vi "W7XBolo2017_Flo.vi"(1 "FPGA VI\nReference In":refnum<k20>) -> (0 "FPGA VI Reference Out":refnum<k20>)   [LabVIEW 2014]
uses:
  <vilib>/Platform/TimedLoop/XDataNode/timing_clust.ctl
  <vilib>/Platform/TimedLoop/XDataNode/nitl_modes.ctl
  <vilib>/Platform/TimedLoop/XDataNode/wakeup.ctl
  <vilib>/userdefined/High Color/nirio_resource_hc.ctl
  <vilib>/DAQmx/write.llb/DAQmx Write (Analog 1D DBL NChan 1Samp).vi
  <vilib>/FPGAPlugInAG/PCI-7813R/niLvFpga_Open_PCI-7813R.vi
  <vilib>/Utility/error.llb/Error Cluster From Error Code.vi
  <vilib>/rvi/errors/niLvFpgaAdjustHostInterfaceError.vi
  <vilib>/Utility/file.llb/Read From Spreadsheet File (I64).vi
  <vilib>/Utility/file.llb/Read From Spreadsheet File (DBL).vi
  <vilib>/DAQmx/create/channels.llb/DAQmx Create Channel (AO-Voltage-Basic).vi
  <vilib>/DAQmx/miscellaneous.llb/DAQmx Fill In Error Info.vi
  <vilib>/rvi/interface/common/niFpgaWaitOnOcc.vi
  <vilib>/httpClient/POSTBuffer.vi
  <vilib>/FPGAPlugInAG/PCI-7813R/niLvFpga_Close_PCI-7813R.vi
  <vilib>/Platform/TimedLoop/XDataNode/XDataNode.xnode
  <vilib>/rvi/interface/nirviOpenFPGA/nirviOpenFPGA.xnode
  FPGA Bitfiles/W7XBolo2017_FPGATarget_fmain2014_DACRangeVoltage.lvbitx
  f_main_2014.vi
  <vilib>/rvi/interface/nirviReadWriteControl/nirviReadWriteControl.xnode
  <vilib>/rvi/interface/nirviMethod/nirviMethod.xnode
  <vilib>/rvi/interface/nirviCloseFPGA/nirviCloseFPGA.xnode
  <vilib>/Platform/TimedLoop/XDataNode/XDNodeRunTimeDep.lvlib
  <vilib>/Analysis/NI_AALBase.lvlib
  <vilib>/httpClient/LabVIEWHTTPClient.lvlib
  <resource>/objmgr/daqmx.rc
  <vilib>/DAQmx/configure/timing.llb/DAQmx Timing (Sample Clock).vi
  <vilib>/DAQmx/write.llb/DAQmx Write (Analog 2D DBL NChan NSamp).vi
  NiFpgaLv.dll
  <vilib>/FPGAPlugInAG/PCI-7813R/niLvFpga_AcknowledgeIrq_PCI-7813R.vi
  <vilib>/FPGAPlugInAG/PCI-7813R/niLvFpga_ConfigureFifo_PCI-7813R.vi
  <vilib>/rvi/errors/niLvFpgaMergeErrorWithErrorCode.vi
panel:
  out "Time until Acqusition":dbl(slide)=60.0 scale=0.0..60.0
  out "DAQ Timer":dbl
  in  "Tab Control 7":T1(tab)
  in  "FreqSelRing":u16(ring)=1 items=["0.8 ms", "1.6 ms", "3.2 ms", "6.4 ms", "12.8 ms", "19.2 ms"]
  in  "SecondFilter":bool=TRUE
  out "SampleTime":sgl=0.0016
  in  "Global DAC Range Setting":u8(knob)=3 scale=0.0..3.0
  out "No. of Samples:":u32=26000
  out "Measured Time for DAQ [ms]":u32
  out "Take file for DAC?":bool
  in  "?":bool=TRUE
  out "Take Input for DAC?":bool
  out "single channel voltage":dbl format="%#_13g"
  in  "DAC and AD Settings":i32(slide)=3 scale=0.0..3.0
  out "Time of Acqusition [s]":dbl=40.0
  out "predicted time [ms] to finalize DAQ":dbl
  out "real time P_rad":dbl format="%#_13g"
  in  "single channel signal factor":dbl=20000.0
  out "voltage on\nsingle channel AO":bool=TRUE
  in  "single channel number":i64=7
  out "loop status":bool
  in  "Auto ECRH Time\nor manual control":bool=TRUE
  out "ECRH duration":dbl=30.0
  in  "manual & default\nDAQ time":dbl=30.0
  out "time needed to\nfind ECRH duration":i64
  in  "SavGol side points":i32=10
  in  "order polynomial":i32=2
  in  "RTPRad voltage factor":dbl=1.0
  out "voltage out state":string
  out "voltage errorsource":string
  out "AO error":errorcluster
  in  "source clock":tag="OnboardClock"
  in  "RegenMode":i32(ring)=10158 items=["Allow Regeneration"=10097, "Do Not Allow Regeneration"=10158]
  in  "AO.DataXferMech 2":i32(ring)=10054 items=["DMA"=10054, "Interrupts"=10204, "Programmed I/O"=10264, "USB Bulk"=12590]
  in  "AO.DataXferReqCond 2":i32(ring)=10242 items=["Onboard Memory Empty"=10235, "Onboard Memory Half Full or Less"=10239, "Onboard Memory Less than Full"=10242]
  in  "sample mode":i32(ring)=10123 items=["Finite Samples"=10178, "Continuous Samples"=10123, "Hardware Timed Single Point"=12522]
  in  "Manual Timing of AO":dbl=100000.0
  out "watchdog loop counter":i32
  out "loop counter":i32
  in  "SkipVoltageOut":bool
  out "Percentage of PC buffer occupied":u8(slide) scale=0.0..100.0
  out "Percentage of OnBoard buffer occupied":u8(slide) scale=0.0..100.0
  out "PC Buffer SpaceAvail":u32
  out "How many \"Write Chunk\" (periods of latency)\nstored in the PC buffer + board buffer?":dbl
  out "How many samples stored in the \nPC buffer + board buffer?":dbl
  in  "Samples per channel to write\n(write chunk)":u32=14
  in  "samples per channel":i32=28
  out "Output.OnbrdBufSize":u32
  out "PC Buffer CurrWritePos 2":dbl
  out "AO output loop timing":dbl
  out "Board TotalSampPerChanGenerated":dbl
  out "How many seconds to empty the \nPC buffer+ board buffer? 2":dbl
  out "RTPVO current val":dbl
  out "SCVO current val":dbl
  in  "Use Voltage or Power for\nsingel channel AO?":bool=TRUE
  in  "voltage watchdog stop":bool
  out "Output.BufSize":u32
  in  "Path to channel selection file":path=path "C:/Users/Administrator/Desktop/short.channel_selection.dat"
  out "file import":i64[][](array[numeric])
  in  "channel selection input":i32[][](array[numeric])=[[1]]
  in  "Read Channel Selection from file":bool=TRUE
  out "Channel Selection\nfrom input?":bool
  out "final channel selection":i64[][](array[numeric])=[[0], [1], [2], [3], [4], [5], [6], [7], [8], [9], [10], [11], [12], [13], [14], [15], [16], [17], [18], [19], [20], [21], [22], [23], [24], [25], [26], [27], [28], [29], [30], [31]]
  out "final channel\nselection size":i32
  in  "Trigger Source":i32(slide)=1 scale=0.0..3.0
  in  "Set Manual Time [ns]":i64=1503619200000000000
  out "Presamples If -1, then no trigger detected)":i32
  out "DAQ wait time (should be = TWT":i32=-1
  out "Countdown Time":u32
  out "Calibration Time":u32
  out "Total wait time (TWT) Typically 59 s":u32
  in  "Pre-start time (ms) of\nDAQ Typically set to 1000 ms":i32=10000
  in  "Fixed T-60sec before T1 = T0":i32=60000
  in  "Wait-Time until Trigger; published on CODAC":u32=10000
  out "current epoch time timestamp":timestamp
  out "Number of nanoseconds with offset to 1904":i64
  in  "samples to exclude":u32=1000
  out "final trigger time":i64
  out "last trigger time by codac":i64
  out "start time":i64
  out "T-Start [for Display)\nShould be -1 [s]":sgl=-1.0
  out "DAQ Start (epoch) [ns]":i64
  out "Downtime after T0 until DAQ [ns]":i64
  in  "timing of plots fix factor":sgl=1.0
  in  "AddOn time":dbl=5.0
  in  "Tau00":dbl[](array[numeric])=[0.11537597448635277, 0.11755685958822219, 0.1164214694473907, 0.11697577239117866, 0.110451, 0.12010942076824872, 0.11766714993048435, 0.11910426529905502, 0.10999582403545866, 0.11118469600664964, 0.10580731993585431, 0.11217289808087993, 0.11223398365603839, 0.11204749607224823, 0.11263624992738425, 0.11091290284745299, 0.11721868902521211, 0.11737061531613151, 0.11788987597885038, 0.11600007869942867, 0.11334307549251021, 0.11228572042130423, 0.1129521332802642, 0.11724104097990388, 0.11740306056822605, 0.11529467898123245, 0.11828175507687082, 0.11829012392284373, 0.11773460668621359, 0.1155776803231521, 0.11650421728110884, 0.11571658330095998, 0.11068789319935994, 0.10986016888144867, 0.10999340462233435, 0.11095550249493497, 0.11143937038853975, 0.11095468517729823, 0.11130783288802211, 0.11084408945769118, 0.10830137260394793, 0.10662335345199567, 0.10535002662491703, 0.10738515206651872, 0.10772145508062766, 0.1053368317440755, 0.10408446186375701, 0.10449038510758271, 0.11178895597256559, 0.11021628063681403, 0.11220331344682449, 0.11111721341359461, 0.10889811436206044, 0.11638094730098773, 0.11290278568076087, 0.11205006536853761, 0.1094907553786962, 0.11634433136641531, 0.11037702264320227, 0.1104223688763365, 0.11352480237507033, 0.11341744936097128, 0.10916961452972393, 0.11332789199343518, 0.11107001747086552, 0.1083853978889723, 0.11029711206697901, 0.11063487469805744, 0.10926615257922916, 0.10988377001368325, 0.10782095764307568, 0.1073886205272185, 0.10829341805096283, 0.10953345610425252, 0.10953147401563214, 0.10933747673483066, 0.1093210854374169, 0.10892908051404164, 0.10841565534876087, 0.10934867623657209, 0.11431979794745441, 0.11469548527952493, 0.11256319960938391, 0.11004758193350624, 0.1086775698186096, 0.10860163257332957, 0.10972644811806966, 0.1244329993560779, 0.10848514148619942, 0.10753497988240919, 0.11378450261362759, 0.11397799701939393, 0.10865166632049855, 0.10955778865143037, 0.11184264538711042, 0.11080028199806266, 0.11230419705417591, 0.11150150302047147, 0.10940920103499238, 0.0, 0.11018788195565775, 0.1109851624674225, 0.10888498891279576, 0.10950524535111039, 0.11209787924272374, 0.11180887164622381, 0.1110290995583749, 0.11040609393156747, 0.1103438351320269, 0.1101975468642728, 0.10923728746964355, 0.0, 0.11021638606642407, 0.0, 0.0, 0.0, 0.0, 0.0, 0.0, 0.0, 0.5609466646481899, 0.0, 0.0, 0.0, 0.0, 0.0, 0.0, 0.4058686463981613, 0.11537597448635277]
  in  "Kappa00":dbl[](array[numeric])=[0.0008396193201719739, 0.0008193409803026575, 0.0008327489337370494, 0.0008094925878469488, 0.00039367506543457065, 0.0008063058560714545, 0.0008451910365158945, 0.0007992358755606012, 0.0008323076933152601, 0.0008570762215527662, 0.0007628861690345087, 0.0008061906602308296, 0.0008540424353779365, 0.0008301118976821594, 0.0008577435335519969, 0.0008553747566925557, 0.000838644207815748, 0.0008273548270536888, 0.0008111923709406437, 0.0008317040544888235, 0.0002062919117538751, 0.0007971782754034694, 0.0007777938427968141, 0.0007983063012770449, 0.0007902138174646686, 0.0007777700527572154, 0.0008086241703327105, 0.0007894905085128677, 0.0008499052168857277, 0.0008231536154986703, 0.0008290108212352768, 0.0008015771948583539, 0.0004219784890145567, 0.0008028223447312654, 0.0007908997677950409, 0.0007688640721813007, 0.0007923143974006498, 0.0007943700234243013, 0.000794807683089336, 0.0007644407575630641, 0.0008256914284962689, 0.0008464663657085921, 0.0008525498714753285, 0.0008605939917038706, 0.0008075301142063146, 0.0008582080819176783, 0.0008833831995156997, 0.0008817750426330745, 0.0008736825873144331, 0.0008712555197947145, 0.0008599116319459445, 0.0008597288697454142, 0.0008850439198466119, 0.0008360600624626481, 0.0008729149198757765, 0.0008652970161905564, 0.000878176403644396, 0.000814669724061475, 0.0008492936703496222, 0.0008335090067364612, 0.0009020306039280142, 0.0009060889736233363, 0.000873120149823901, 0.0008865804075398461, 0.0008218319952538781, 0.0008647381541051004, 0.0008535415687509321, 0.000868609807906937, 0.0008544506047017487, 0.0008552184337763689, 0.0008772351584693919, 0.0008899531428744609, 0.0009049492537694576, 0.000908105157129488, 0.0009441675693280472, 0.0008666158415307141, 0.0008904383660716827, 0.00090533600441176, 0.0009193630525411423, 0.0009209094258700529, 0.0008671616817531277, 0.0008573033056411677, 0.0008894545060438134, 0.0008393076570230061, 0.0008809839906701387, 0.0008713273912310079, 0.0008529389904228485, 0.0008798583497112145, 0.0007606961064025662, 0.0007618681674480262, 0.0008830002472907413, 0.0008434447500347438, 0.0008157810403546725, 0.0008170412330426688, 0.000817539692314199, 0.0008060567476264818, 0.0007745714382802376, 0.0007738842512393123, 0.0007910139604008742, -1.9640688433259297e-10, 0.000780575223559956, 0.0007962779122750964, 0.000790630439080113, 0.0008189866992119251, 0.0008220353590981327, 0.0008259174124746273, 0.0008237041516630779, 0.0008128375228315313, 0.0008025139618430593, 0.0007891459070721132, 0.0007835394415130632, 1.4659311061625464e-11, 0.0007713911232202254, -1.136328152026204e-11, 7.33972615530204e-11, -5.807996136265078e-12, 1.50989391544806e-10, -2.091237015882531e-11, -2.2968171315336452e-11, 3.2003514158147334e-12, -1.18410213996469e-13, 3.9907860061368183e-13, 1.2900003061146403e-11, -7.996494711993759e-11, 1.2728268766879732e-10, -2.7124534936566837e-11, -1.0618681361847593e-11, 1.1300143559461795e-05]
  in  "RB000":dbl[](array[numeric])=[964.4665558152926, 984.0412138536651, 1001.0627256989599, 1012.7898525309201, 986.7279110070629, 993.5830261423998, 1133.718466702734, 1026.065541032409, 981.7525515631839, 976.6051330676225, 975.1369773387203, 983.6003740876943, 945.3052421117454, 944.0131212191011, 937.9865397688445, 924.775520494105, 1002.3909240348048, 1016.474188810108, 1008.3024841336951, 997.8517562562979, 1396.1357804303618, 1011.7052948010587, 1006.0858095523904, 1000.525119034801, 1016.071205963885, 1008.5531713944379, 1001.2101495655734, 1012.9539707105694, 909.9522463978296, 921.8611396886308, 930.8535575645451, 937.6736260749049, 1835.253905213153, 905.3151174073253, 915.4686408360067, 932.2842954450018, 878.6376527118448, 888.8892103361444, 896.5962281010978, 917.195767017641, 953.2009542047422, 949.8476734916919, 945.7180214798805, 934.1303098026676, 944.4309270141721, 922.393020385211, 908.2770101975661, 902.8479184676862, 997.7185120044248, 1004.633250147941, 1012.2992174178987, 1022.8972656361334, 988.1138139759116, 1012.5096483256309, 926.7526927543831, 940.6499588809413, 987.4981539235332, 1030.6093168535383, 996.69488158787, 998.6770565199763, 937.2653710614366, 942.0245103372197, 975.0990877775471, 954.8089604337308, 987.3564837474132, 941.2547128561528, 982.5095895382428, 979.0417371038707, 995.2373497220817, 994.8506309175264, 989.7979732647505, 986.9344569144992, 979.4724674608722, 951.8026661804106, 928.3096097998925, 980.4648125251251, 967.8736951300871, 960.399052288677, 950.3474867516031, 931.7877057694141, 925.6104123406642, 925.2905333073797, 925.2586242376997, 996.0089625341668, 969.8590336679081, 973.5395443351913, 978.7443359479869, 1329.6132687126426, 951.8837808548863, 946.7262849537287, 933.7058147126331, 940.8228530266879, 876.367589172054, 864.1420943242144, 855.6188139335973, 854.7591574173059, 955.1936774096923, 969.1826763753277, 970.8033011923455, 0.0, 935.2179320514933, 937.6581182076873, 940.1867678977421, 939.4080093580444, 850.4194498630884, 857.7406858104588, 867.3881837894808, 884.270800315495, 892.6618762043922, 899.3995556852765, 915.5186423922648, 0.0, 919.5685811076437, 0.0, 0.0, 0.0, 0.0, 0.0, 0.0, 0.0, 0.0, 0.0, 0.0, 0.0, 0.0, 0.0, 0.0, 0.0]
  in  "Switch to fixed \nCalibration Values":bool
  in  "Clear all Values \nfrom Beginning":bool
  in  "Cancel Button":bool
  out "Actual Depth":u32=256
  in  "Trigger No Choice from MDS+ Website\n0 for old 1 during OP":i32
  in  "AD 7730 Bit Settings":i32(slide) scale=0.0..1.0
  out "CODAC trigger time":i64
  out "date/time string":string
  out "Sucessfull HTTP return?":bool
  out "progId":dbl
  in  "Tab Control":T2(tab)
  out "real time P_rad array":dbl[](array[numeric])
  out "all plot":cluster{cluster{dbl, "element":dbl}[]}[](graph)
  out "full P_rad [MW] HBC":dbl[](array[numeric])
  out "single channel voltage array":dbl[](array[numeric])
  out "full P_rad [MW] VBC":dbl[](array[numeric])
  in  "Tab Control 4":enum32{"1 to 64", "65 to 128"}(tab)
  out "Raw 33-64":T3={"Channels 33 - 40"={"tstart"=-1.0, "FPGSampleTime"=0.0007999999797903001, []}, "Channels 41 - 48"={"tstart"=-1.0, "FPGSampleTime"=0.0007999999797903001, []}, "Channels 49 - 56"={"tstart"=-1.0, "FPGSampleTime"=0.0007999999797903001, []}, "Channels 57 - 64"={"tstart"=-1.0, "FPGSampleTime"=0.0007999999797903001, []}}
  out "Raw 1-32":T4={"Channels 1- 8"={"tstart"=-1.0, "FPGSampleTime"=0.0007999999797903001, []}, "Channels 9 - 16"={"tstart"=-1.0, "FPGSampleTime"=0.0007999999797903001, []}, "Channels 17 - 24"={"tstart"=-1.0, "FPGSampleTime"=0.0007999999797903001, []}, "Channels 25 - 32"={"tstart"=-1.0, "FPGSampleTime"=0.0007999999797903001, []}}
  out "Raw 97 - 128":T5
  out "Raw 65 - 97":T6={"Channels 65 - 71"={"tstart"=-1.0, "FPGSampleTime"=0.0007999999797903001, []}, "Channels 73 - 80"={"tstart"=0.0, "FPGSampleTime"=0.0, []}, "Channels 81 - 88"={"tstart"=0.0, "FPGSampleTime"=0.0, []}, "Channels 89- 96"={"tstart"=0.0, "FPGSampleTime"=0.0, []}}
  in  "Tab Control 13":enum32{"1 to 64", "65 to 128"}(tab)
  out "Adjusted 33-64":T3={"Channels 33 - 40"={"tstart"=-1.0, "FPGSampleTime"=0.0007999999797903001, []}, "Channels 41 - 48"={"tstart"=-1.0, "FPGSampleTime"=0.0007999999797903001, []}, "Channels 49 - 56"={"tstart"=-1.0, "FPGSampleTime"=0.0007999999797903001, []}, "Channels 57 - 64"={"tstart"=-1.0, "FPGSampleTime"=0.0007999999797903001, []}}
  out "Adjusted 1-32":T4={"Channels 1- 8"={"tstart"=-1.0, "FPGSampleTime"=0.0007999999797903001, []}, "Channels 9 - 16"={"tstart"=-1.0, "FPGSampleTime"=0.0007999999797903001, []}, "Channels 17 - 24"={"tstart"=-1.0, "FPGSampleTime"=0.0007999999797903001, []}, "Channels 25 - 32"={"tstart"=-1.0, "FPGSampleTime"=0.0007999999797903001, []}}
  out "Adjusted 97 - 129":T5
  out "Adjusted 65 - 98":T6={"Channels 65 - 71"={"tstart"=-1.0, "FPGSampleTime"=0.0007999999797903001, []}, "Channels 73 - 80"={"tstart"=0.0, "FPGSampleTime"=0.0, []}, "Channels 81 - 88"={"tstart"=0.0, "FPGSampleTime"=0.0, []}, "Channels 89- 96"={"tstart"=0.0, "FPGSampleTime"=0.0, []}}
  in  "Tab Control 6":enum32{"1 to 64", "65 to 128"}(tab)
  out "Pow 33-64":T3
  out "Pow 1-32":T4={"Channels 1- 8"={"tstart"=-1.0, "FPGSampleTime"=0.0007999999797903001, []}, "Channels 9 - 16"={"tstart"=-1.0, "FPGSampleTime"=0.0007999999797903001, []}, "Channels 17 - 24"={"tstart"=0.0, "FPGSampleTime"=0.0, []}, "Channels 25 - 32"={"tstart"=0.0, "FPGSampleTime"=0.0, []}}
  out "Pow 97 - 128":T5
  out "Pow 65 - 96":T6={"Channels 65 - 71"={"tstart"=-1.0, "FPGSampleTime"=0.0007999999797903001, []}, "Channels 73 - 80"={"tstart"=0.0, "FPGSampleTime"=0.0, []}, "Channels 81 - 88"={"tstart"=0.0, "FPGSampleTime"=0.0, []}, "Channels 89- 96"={"tstart"=0.0, "FPGSampleTime"=0.0, []}}
  out "full P_rad plot":T7(graph)
  out "CalibRefFoilFit path":string
  out "BoloCalibRefFoilFit Satus":bool
  out "Offset path":string
  out "Offset Status":bool
  out "RTau Path":string
  out "RTau Status":bool
  out "MKappa path":string
  out "RRes path":string
  out "MTau path":string
  out "RRes Status":bool
  out "MKappa Status":bool
  out "MTau status":bool
  out "BoloPower path":string
  out "QSBParms path":string
  out "BoloSignal path":string
  out "CalibMeasFoilCurrent path":string
  out "CalibRefFoilCurrent path":string
  out "MRes path":string
  out "RKappa path":string
  out "RKappa Status":bool
  out "CalibRefFoilCurrent status":bool
  out "CalibMeasFoilCurrent status":bool
  out "MRes status":bool
  out "BoloSignal status":bool
  out "QSBParms status":bool
  out "BoloPower status":bool
  out "SingleChannelFeedback status":bool
  out "SingleChannelFeedback path":string
  out "ChannelSelection status":bool
  out "ChannelSelection path":string
  out "Bolo_HBCmPrad path":string
  out "Bolo_HBCmPrad status":bool
  out "CalibMeasFoilFit path":string
  out "CalibMeasFoilFit status":bool
  out "Bolo_VBCPrad status":bool
  out "Bolo_VBCPrad path":string
  out "RT_P_rad path":string
  out "RT_P_rad status":bool
  out "MessStatus 65-96":bool[](array[boolean])
  out "MessStatus 97-128":bool[](array[boolean])
  out "MessStatus 33-64":bool[](array[boolean])
  out "MessStatus 1-32":bool[](array[boolean])
  out "RefStatus 97-128":bool[](array[boolean])
  out "RefStatus 1-32":bool[](array[boolean])
  out "RefStatus 33-64":bool[](array[boolean])
  out "RefStatus 65-96":bool[](array[boolean])
  out "voltage status":bool
  out "result":bool
  out "FilterTimeOut":bool
  out "Fehler READ U+P":bool
  out "Fehler":bool
  out "Timed Out":bool
  out "BoloAdjusted path":string
  out "BoloSignal status 2":bool
  in  "Tab Control 14":T8(tab)=enum."Parlog"
  out "BoloSignalErrorOut 2":errorcluster
  out "body Parlog 18":string
  out "headers parms 18":string
  out "headers 18":string
  out "body 18":string
  in  "Tab Control 12":T9(tab)=enum."Parlog"
  out "RT_P_rad ErrorOut":errorcluster
  out "body Parlog 17":string
  out "headers 17":string
  out "body 17":string
  out "headers parms 17":string
  in  "Tab Control 31":T10(tab)=enum."Parlog"
  out "parms error out":errorcluster
  out "QSB Parms Out body chanDesc":string
  out "QSB Parms Out headers chanDesc":string
  in  "Tab Control 30":T11(tab)=enum."Parlog"
  out "CalibMeasFoilFit 2":errorcluster
  out "body Parlog":string
  out "headers parms":string
  out "body":string
  out "headers":string
  in  "Tab Control 29":T12(tab)=enum."Parlog"
  out "RKappaErrorOut":errorcluster
  out "body Parlog 3":string
  out "headers parms 3":string
  out "body 3":string
  out "headers 3":string
  in  "Tab Control 28":enum32{"MTau ErrorOut", "Parlog", "Datastream"}(tab)=enum."Parlog"
  out "MTauErrorOut":errorcluster
  out "body Parlog 16":string
  out "headers parms 16":string
  out "body 16":string
  out "headers 16":string
  in  "Tab Control 27":enum32{"MRes ErrorOut", "Parlog", "Datastream"}(tab)=enum."Parlog"
  out "MResErrorOut":errorcluster
  out "body Parlog 6":string
  out "headers parms 6":string
  out "body 6":string
  out "headers 6":string
  in  "Tab Control 26":T13(tab)=enum."Parlog"
  out "BoloPowerRawErrorOut":errorcluster
  out "body Parlog 10":string
  out "headers parms 10":string
  out "body 10":string
  out "headers 10":string
  in  "Tab Control 25":T14(tab)=enum."Parlog"
  out "CalibMeasFoilCurrentErrorOut":errorcluster
  out "body Parlog 7":string
  out "headers parms 7":string
  out "body 7":string
  out "headers 7":string
  in  "Tab Control 24":T15(tab)=enum."Parlog"
  out "BoloSignalErrorOut":errorcluster
  out "body Parlog 9":string
  out "headers parms 9":string
  out "body 9":string
  out "headers 9":string
  in  "Tab Control 23":T16(tab)=enum."Parlog"
  out "CalibRefFoilCurrentErrorOut":errorcluster
  out "body Parlog 8":string
  out "headers parms 8":string
  out "body 8":string
  out "headers 8":string
  in  "Tab Control 22":T17(tab)=enum."Parlog"
  out "BoloCalibRefFoilFitErrorOut":errorcluster
  out "body Parlog 11":string
  out "headers parms 11":string
  out "body 11":string
  out "headers 11":string
  in  "Tab Control 21":enum32{"RRes ErrorOut", "Parlog", "Datastream"}(tab)=enum."Parlog"
  out "RResErrorOut":errorcluster
  out "body Parlog 5":string
  out "headers parms 5":string
  out "body 5":string
  out "headers 5":string
  in  "Tab Control 20":T18(tab)=enum."Parlog"
  out "OffsetErrorOut":errorcluster
  out "body Parlog 15":string
  out "headers parms 15":string
  out "body 15":string
  out "headers 15":string
  in  "Tab Control 19":T19(tab)=enum."Parlog"
  out "MKappaErrorOut":errorcluster
  out "body Parlog 2":string
  out "headers parms 2":string
  out "body 2":string
  out "headers 2":string
  in  "Tab Control 8":T20(tab)=enum."Parlog"
  out "ChannelSelection ErrorOut":errorcluster
  out "ChannelSelection body Parlog":string
  out "ChannelSelection headers parms":string
  out "ChannelSelection body":string
  out "ChannelSelection headers":string
  out "error out":errorcluster
  out "error out Cal":errorcluster
  in  "chanDescs":T21(array[cluster])=[{"name"="HBCm_U30_01", "active"=1, "physicalQuantity"={"type"="A"}}, {"name"="HBCm_U30_02", "active"=1, "physicalQuantity"={"type"="A"}}, {"name"="HBCm_U30_03", "active"=1, "physicalQuantity"={"type"="A"}}, {"name"="HBCm_U30_04", "active"=1, "physicalQuantity"={"type"="A"}}, {"name"="HBCm_U30_05", "active"=1, "physicalQuantity"={"type"="A"}}, {"name"="HBCm_U30_06", "active"=1, "physicalQuantity"={"type"="A"}}, {"name"="HBCm_U30_07", "active"=1, "physicalQuantity"={"type"="A"}}, {"name"="HBCm_U30_08", "active"=1, "physicalQuantity"={"type"="A"}}, {"name"="HBCm_U30_09", "active"=1, "physicalQuantity"={"type"="A"}}, {"name"="HBCm_U30_10", "active"=1, "physicalQuantity"={"type"="A"}}, {"name"="HBCm_U30_11", "active"=1, "physicalQuantity"={"type"="A"}}, {"name"="HBCm_U30_12", "active"=1, "physicalQuantity"={"type"="A"}}, {"name"="HBCm_U30_013", "active"=1, "physicalQuantity"={"type"="A"}}, {"name"="HBCm_U30_14", "active"=1, "physicalQuantity"={"type"="A"}}, {"name"="HBCm_U30_15", "active"=1, "physicalQuantity"={"type"="A"}}, {"name"="HBCm_U30_16", "active"=1, "physicalQuantity"={"type"="A"}}, {"name"="HBCm_U30_17", "active"=1, "physicalQuantity"={"type"="A"}}, {"name"="HBCm_U30_18", "active"=1, "physicalQuantity"={"type"="A"}}, {"name"="HBCm_U30_19", "active"=1, "physicalQuantity"={"type"="A"}}, {"name"="HBCm_U30_20", "active"=1, "physicalQuantity"={"type"="A"}}, {"name"="HBCm_U30_21", "active"=1, "physicalQuantity"={"type"="A"}}, {"name"="HBCm_U30_22", "active"=1, "physicalQuantity"={"type"="A"}}, {"name"="HBCm_U30_23", "active"=1, "physicalQuantity"={"type"="A"}}, {"name"="HBCm_U30_24", "active"=1, "physicalQuantity"={"type"="A"}}, {"name"="HBCm_U30_25", "active"=1, "physicalQuantity"={"type"="A"}}, {"name"="HBCm_U30_26", "active"=1, "physicalQuantity"={"type"="A"}}, {"name"="HBCm_U30_27", "active"=1, "physicalQuantity"={"type"="A"}}, {"name"="HBCm_U30_28", "active"=1, "physicalQuantity"={"type"="A"}}, {"name"="HBCm_U30_29", "active"=1, "physicalQuantity"={"type"="A"}}, {"name"="HBCm_U30_30", "active"=1, "physicalQuantity"={"type"="A"}}, {"name"="HBCm_U30_31", "active"=1, "physicalQuantity"={"type"="A"}}, {"name"="HBCm_U30_32", "active"=1, "physicalQuantity"={"type"="A"}}, {"name"="VBCm_V21_01", "active"=1, "physicalQuantity"={"type"="A"}}, {"name"="VBCm_V21_02", "active"=1, "physicalQuantity"={"type"="A"}}, {"name"="VBCm_V21_03", "active"=1, "physicalQuantity"={"type"="A"}}, {"name"="VBCm_V21_04", "active"=1, "physicalQuantity"={"type"="A"}}, {"name"="VBCm_V21_05", "active"=1, "physicalQuantity"={"type"="A"}}, {"name"="VBCm_V21_06", "active"=1, "physicalQuantity"={"type"="A"}}, {"name"="VBCm_V21_07", "active"=1, "physicalQuantity"={"type"="A"}}, {"name"="VBCm_V21_08", "active"=1, "physicalQuantity"={"type"="A"}}, {"name"="VBCm_V21_09", "active"=1, "physicalQuantity"={"type"="A"}}, {"name"="VBCm_V21_10", "active"=1, "physicalQuantity"={"type"="A"}}, {"name"="VBCm_V21_11", "active"=1, "physicalQuantity"={"type"="A"}}, {"name"="VBCm_V21_12", "active"=1, "physicalQuantity"={"type"="A"}}, {"name"="VBCm_V21_13", "active"=1, "physicalQuantity"={"type"="A"}}, {"name"="VBCm_V21_14", "active"=1, "physicalQuantity"={"type"="A"}}, {"name"="VBCm_V21_15", "active"=1, "physicalQuantity"={"type"="A"}}, {"name"="VBCm_V21_16", "active"=1, "physicalQuantity"={"type"="A"}}, {"name"="VBCm_V21_17", "active"=1, "physicalQuantity"={"type"="A"}}, {"name"="VBCm_V21_18", "active"=1, "physicalQuantity"={"type"="A"}}, {"name"="VBCm_V21_19", "active"=1, "physicalQuantity"={"type"="A"}}, {"name"="VBCm_V21_20", "active"=1, "physicalQuantity"={"type"="A"}}, {"name"="VBCm_V21_21", "active"=1, "physicalQuantity"={"type"="A"}}, {"name"="VBCm_V21_22", "active"=1, "physicalQuantity"={"type"="A"}}, {"name"="VBCm_V21_23", "active"=1, "physicalQuantity"={"type"="A"}}, {"name"="VBCm_V21_24", "active"=1, "physicalQuantity"={"type"="A"}}, {"name"="VBCm_V21_25", "active"=1, "physicalQuantity"={"type"="A"}}, {"name"="VBCm_V21_26", "active"=1, "physicalQuantity"={"type"="A"}}, {"name"="VBCm_V21_27", "active"=1, "physicalQuantity"={"type"="A"}}, {"name"="VBCm_V21_28", "active"=1, "physicalQuantity"={"type"="A"}}, {"name"="VBCm_V21_29", "active"=1, "physicalQuantity"={"type"="A"}}, {"name"="VBCm_V21_30", "active"=1, "physicalQuantity"={"type"="A"}}, {"name"="VBCm_V21_31", "active"=1, "physicalQuantity"={"type"="A"}}, {"name"="VBCm_V21_32", "active"=1, "physicalQuantity"={"type"="A"}}, {"name"="VBCm_V21_33", "active"=1, "physicalQuantity"={"type"="A"}}, {"name"="VBCm_V21_34", "active"=1, "physicalQuantity"={"type"="A"}}, {"name"="VBCm_V21_35", "active"=1, "physicalQuantity"={"type"="A"}}, {"name"="VBCm_V21_36", "active"=1, "physicalQuantity"={"type"="A"}}, {"name"="VBCm_V21_37", "active"=1, "physicalQuantity"={"type"="A"}}, {"name"="VBCm_V21_38", "active"=1, "physicalQuantity"={"type"="A"}}, {"name"="VBCm_V21_39", "active"=1, "physicalQuantity"={"type"="A"}}, {"name"="VBCm_V21_40", "active"=1, "physicalQuantity"={"type"="A"}}, {"name"="VBCs_V21_01", "active"=1, "physicalQuantity"={"type"="A"}}, {"name"="VBCs_V21_02", "active"=1, "physicalQuantity"={"type"="A"}}, {"name"="VBCs_V21_03", "active"=1, "physicalQuantity"={"type"="A"}}, {"name"="VBCs_V21_04", "active"=1, "physicalQuantity"={"type"="A"}}, {"name"="VBCs_V21_05", "active"=1, "physicalQuantity"={"type"="A"}}, {"name"="VBCs_V21_06", "active"=1, "physicalQuantity"={"type"="A"}}, {"name"="VBCs_V21_07", "active"=1, "physicalQuantity"={"type"="A"}}, {"name"="VBCs_V21_08", "active"=1, "physicalQuantity"={"type"="A"}}, {"name"="HBCs_U30_01", "active"=1, "physicalQuantity"={"type"="A"}}, {"name"="HBCs_U30_02", "active"=1, "physicalQuantity"={"type"="A"}}, {"name"="HBCs_U30_03", "active"=1, "physicalQuantity"={"type"="A"}}, {"name"="HBCs_U30_04", "active"=1, "physicalQuantity"={"type"="A"}}, {"name"="HBCs_U30_05", "active"=1, "physicalQuantity"={"type"="A"}}, {"name"="HBCs_U30_06", "active"=1, "physicalQuantity"={"type"="A"}}, {"name"="HBCs_U30_07", "active"=1, "physicalQuantity"={"type"="A"}}, {"name"="HBCs_U30_08", "active"=1, "physicalQuantity"={"type"="A"}}, {"name"="HBCs_U30_09", "active"=1, "physicalQuantity"={"type"="A"}}, {"name"="HBCs_U30_10", "active"=1, "physicalQuantity"={"type"="A"}}, {"name"="HBCs_U30_11", "active"=1, "physicalQuantity"={"type"="A"}}, {"name"="HBCs_U30_12", "active"=1, "physicalQuantity"={"type"="A"}}, {"name"="HBCs_U30_13", "active"=1, "physicalQuantity"={"type"="A"}}, {"name"="HBCs_U30_14", "active"=1, "physicalQuantity"={"type"="A"}}, {"name"="HBCs_U30_15", "active"=1, "physicalQuantity"={"type"="A"}}, {"name"="HBCs_U30_16", "active"=1, "physicalQuantity"={"type"="A"}}]
  in  "Tab Control 9":T22(tab)=enum."Parlog"
  out "Bolo_VBCPrad ErrorOut":errorcluster
  out "body Parlog 14":string
  out "headers parms 14":string
  out "body 14":string
  out "headers 14":string
  in  "Tab Control 11":enum32{"RTau ErrorOut", "Parlog", "Datastream"}(tab)=enum."Parlog"
  out "RTauErrorOut":errorcluster
  out "body Parlog 4":string
  out "headers parms 4":string
  out "body 4":string
  out "headers 4":string
  in  "Tab Control 18":T23(tab)=enum."Parlog"
  out "SingleChannelFeedbackErrorOut":errorcluster
  out "headers parms 12":string
  out "body Parlog 12":string
  out "body 12":string
  out "headers 12":string
  in  "Tab Control 10":T24(tab)=enum."Parlog"
  out "Bolo_HBCmPrad ErrorOut":errorcluster
  out "body Parlog 13":string
  out "headers parms 13":string
  out "body 13":string
  out "headers 13":string
  out "QSB Parms JSON string":string
  out "ChannelSelectionJSON":string
  out "SingleChannelFeedbackJSON":string
  out "PowerRawJSON":string
  out "BoloSignalJSON":string
  out "CalibRefFoilFitJSON":string
  out "MResJSON":string
  out "MKappaJSON":string
  out "CalibMeasFoilCurrentJSON":string
  out "RKappaJSON":string
  out "MTauJSON":string
  out "CalibMeasFoilFit":string
  out "CalibRefFoilCurrentJSON":string
  out "RResJSON":string
  out "RTauJSON":string
  out "OffsetJSON":string
  out "DimensionsD":i64[](array[numeric])
  out "DimensionsC":i64[](array[numeric])
  out "DimensionsB":i64[](array[numeric])
  out "DimensionsA":i64[](array[numeric])
  out "cluster array":T25(array[cluster])
  out "reduced cluster array":T26(array[cluster])
  out "cluster":T27
  out "reduced cluster":T28
  out "chanDescsInd":T21(array[cluster])=[{"name"="HBCm_U30_01", "active"=1, "physicalQuantity"={"type"="A"}}, {"name"="HBCm_U30_02", "active"=1, "physicalQuantity"={"type"="A"}}, {"name"="HBCm_U30_03", "active"=1, "physicalQuantity"={"type"="A"}}, {"name"="HBCm_U30_04", "active"=1, "physicalQuantity"={"type"="A"}}, {"name"="HBCm_U30_05", "active"=1, "physicalQuantity"={"type"="A"}}, {"name"="HBCm_U30_06", "active"=1, "physicalQuantity"={"type"="A"}}, {"name"="HBCm_U30_07", "active"=1, "physicalQuantity"={"type"="A"}}, {"name"="HBCm_U30_08", "active"=1, "physicalQuantity"={"type"="A"}}, {"name"="HBCm_U30_09", "active"=1, "physicalQuantity"={"type"="A"}}, {"name"="HBCm_U30_10", "active"=1, "physicalQuantity"={"type"="A"}}, {"name"="HBCm_U30_11", "active"=1, "physicalQuantity"={"type"="A"}}, {"name"="HBCm_U30_12", "active"=1, "physicalQuantity"={"type"="A"}}, {"name"="HBCm_U30_013", "active"=1, "physicalQuantity"={"type"="A"}}, {"name"="HBCm_U30_14", "active"=1, "physicalQuantity"={"type"="A"}}, {"name"="HBCm_U30_15", "active"=1, "physicalQuantity"={"type"="A"}}, {"name"="HBCm_U30_16", "active"=1, "physicalQuantity"={"type"="A"}}, {"name"="HBCm_U30_17", "active"=1, "physicalQuantity"={"type"="A"}}, {"name"="HBCm_U30_18", "active"=1, "physicalQuantity"={"type"="A"}}, {"name"="HBCm_U30_19", "active"=1, "physicalQuantity"={"type"="A"}}, {"name"="HBCm_U30_20", "active"=1, "physicalQuantity"={"type"="A"}}, {"name"="HBCm_U30_21", "active"=1, "physicalQuantity"={"type"="A"}}, {"name"="HBCm_U30_22", "active"=1, "physicalQuantity"={"type"="A"}}, {"name"="HBCm_U30_23", "active"=1, "physicalQuantity"={"type"="A"}}, {"name"="HBCm_U30_24", "active"=1, "physicalQuantity"={"type"="A"}}, {"name"="HBCm_U30_25", "active"=1, "physicalQuantity"={"type"="A"}}, {"name"="HBCm_U30_26", "active"=1, "physicalQuantity"={"type"="A"}}, {"name"="HBCm_U30_27", "active"=1, "physicalQuantity"={"type"="A"}}, {"name"="HBCm_U30_28", "active"=1, "physicalQuantity"={"type"="A"}}, {"name"="HBCm_U30_29", "active"=1, "physicalQuantity"={"type"="A"}}, {"name"="HBCm_U30_30", "active"=1, "physicalQuantity"={"type"="A"}}, {"name"="HBCm_U30_31", "active"=1, "physicalQuantity"={"type"="A"}}, {"name"="HBCm_U30_32", "active"=1, "physicalQuantity"={"type"="A"}}, {"name"="VBCm_V21_01", "active"=1, "physicalQuantity"={"type"="A"}}, {"name"="VBCm_V21_02", "active"=1, "physicalQuantity"={"type"="A"}}, {"name"="VBCm_V21_03", "active"=1, "physicalQuantity"={"type"="A"}}, {"name"="VBCm_V21_04", "active"=1, "physicalQuantity"={"type"="A"}}, {"name"="VBCm_V21_05", "active"=1, "physicalQuantity"={"type"="A"}}, {"name"="VBCm_V21_06", "active"=1, "physicalQuantity"={"type"="A"}}, {"name"="VBCm_V21_07", "active"=1, "physicalQuantity"={"type"="A"}}, {"name"="VBCm_V21_08", "active"=1, "physicalQuantity"={"type"="A"}}, {"name"="VBCm_V21_09", "active"=1, "physicalQuantity"={"type"="A"}}, {"name"="VBCm_V21_10", "active"=1, "physicalQuantity"={"type"="A"}}, {"name"="VBCm_V21_11", "active"=1, "physicalQuantity"={"type"="A"}}, {"name"="VBCm_V21_12", "active"=1, "physicalQuantity"={"type"="A"}}, {"name"="VBCm_V21_13", "active"=1, "physicalQuantity"={"type"="A"}}, {"name"="VBCm_V21_14", "active"=1, "physicalQuantity"={"type"="A"}}, {"name"="VBCm_V21_15", "active"=1, "physicalQuantity"={"type"="A"}}, {"name"="VBCm_V21_16", "active"=1, "physicalQuantity"={"type"="A"}}, {"name"="VBCm_V21_17", "active"=1, "physicalQuantity"={"type"="A"}}, {"name"="VBCm_V21_18", "active"=1, "physicalQuantity"={"type"="A"}}, {"name"="VBCm_V21_19", "active"=1, "physicalQuantity"={"type"="A"}}, {"name"="VBCm_V21_20", "active"=1, "physicalQuantity"={"type"="A"}}, {"name"="VBCm_V21_21", "active"=1, "physicalQuantity"={"type"="A"}}, {"name"="VBCm_V21_22", "active"=1, "physicalQuantity"={"type"="A"}}, {"name"="VBCm_V21_23", "active"=1, "physicalQuantity"={"type"="A"}}, {"name"="VBCm_V21_24", "active"=1, "physicalQuantity"={"type"="A"}}, {"name"="VBCm_V21_25", "active"=1, "physicalQuantity"={"type"="A"}}, {"name"="VBCm_V21_26", "active"=1, "physicalQuantity"={"type"="A"}}, {"name"="VBCm_V21_27", "active"=1, "physicalQuantity"={"type"="A"}}, {"name"="VBCm_V21_28", "active"=1, "physicalQuantity"={"type"="A"}}, {"name"="VBCm_V21_29", "active"=1, "physicalQuantity"={"type"="A"}}, {"name"="VBCm_V21_30", "active"=1, "physicalQuantity"={"type"="A"}}, {"name"="VBCm_V21_31", "active"=1, "physicalQuantity"={"type"="A"}}, {"name"="VBCm_V21_32", "active"=1, "physicalQuantity"={"type"="A"}}, {"name"="VBCm_V21_33", "active"=1, "physicalQuantity"={"type"="A"}}, {"name"="VBCm_V21_34", "active"=1, "physicalQuantity"={"type"="A"}}, {"name"="VBCm_V21_35", "active"=1, "physicalQuantity"={"type"="A"}}, {"name"="VBCm_V21_36", "active"=1, "physicalQuantity"={"type"="A"}}, {"name"="VBCm_V21_37", "active"=1, "physicalQuantity"={"type"="A"}}, {"name"="VBCm_V21_38", "active"=1, "physicalQuantity"={"type"="A"}}, {"name"="VBCm_V21_39", "active"=1, "physicalQuantity"={"type"="A"}}, {"name"="VBCm_V21_40", "active"=1, "physicalQuantity"={"type"="A"}}, {"name"="VBCs_V21_01", "active"=1, "physicalQuantity"={"type"="A"}}, {"name"="VBCs_V21_02", "active"=1, "physicalQuantity"={"type"="A"}}, {"name"="VBCs_V21_03", "active"=1, "physicalQuantity"={"type"="A"}}, {"name"="VBCs_V21_04", "active"=1, "physicalQuantity"={"type"="A"}}, {"name"="VBCs_V21_05", "active"=1, "physicalQuantity"={"type"="A"}}, {"name"="VBCs_V21_06", "active"=1, "physicalQuantity"={"type"="A"}}, {"name"="VBCs_V21_07", "active"=1, "physicalQuantity"={"type"="A"}}, {"name"="VBCs_V21_08", "active"=1, "physicalQuantity"={"type"="A"}}, {"name"="HBCs_U30_01", "active"=1, "physicalQuantity"={"type"="A"}}, {"name"="HBCs_U30_02", "active"=1, "physicalQuantity"={"type"="A"}}, {"name"="HBCs_U30_03", "active"=1, "physicalQuantity"={"type"="A"}}, {"name"="HBCs_U30_04", "active"=1, "physicalQuantity"={"type"="A"}}, {"name"="HBCs_U30_05", "active"=1, "physicalQuantity"={"type"="A"}}, {"name"="HBCs_U30_06", "active"=1, "physicalQuantity"={"type"="A"}}, {"name"="HBCs_U30_07", "active"=1, "physicalQuantity"={"type"="A"}}, {"name"="HBCs_U30_08", "active"=1, "physicalQuantity"={"type"="A"}}, {"name"="HBCs_U30_09", "active"=1, "physicalQuantity"={"type"="A"}}, {"name"="HBCs_U30_10", "active"=1, "physicalQuantity"={"type"="A"}}, {"name"="HBCs_U30_11", "active"=1, "physicalQuantity"={"type"="A"}}, {"name"="HBCs_U30_12", "active"=1, "physicalQuantity"={"type"="A"}}, {"name"="HBCs_U30_13", "active"=1, "physicalQuantity"={"type"="A"}}, {"name"="HBCs_U30_14", "active"=1, "physicalQuantity"={"type"="A"}}, {"name"="HBCs_U30_15", "active"=1, "physicalQuantity"={"type"="A"}}, {"name"="HBCs_U30_16", "active"=1, "physicalQuantity"={"type"="A"}}]
  out "chanDescs_defaultInd":T21(array[cluster])=[{"name"="HBCm_U30_01", "active"=1, "physicalQuantity"={"type"="A"}}, {"name"="HBCm_U30_02", "active"=1, "physicalQuantity"={"type"="A"}}, {"name"="HBCm_U30_03", "active"=1, "physicalQuantity"={"type"="A"}}, {"name"="HBCm_U30_04", "active"=1, "physicalQuantity"={"type"="A"}}, {"name"="HBCm_U30_05", "active"=1, "physicalQuantity"={"type"="A"}}, {"name"="HBCm_U30_06", "active"=1, "physicalQuantity"={"type"="A"}}, {"name"="HBCm_U30_07", "active"=1, "physicalQuantity"={"type"="A"}}, {"name"="HBCm_U30_08", "active"=1, "physicalQuantity"={"type"="A"}}, {"name"="HBCm_U30_09", "active"=1, "physicalQuantity"={"type"="A"}}, {"name"="HBCm_U30_10", "active"=1, "physicalQuantity"={"type"="A"}}, {"name"="HBCm_U30_11", "active"=1, "physicalQuantity"={"type"="A"}}, {"name"="HBCm_U30_12", "active"=1, "physicalQuantity"={"type"="A"}}, {"name"="HBCm_U30_13", "active"=1, "physicalQuantity"={"type"="A"}}, {"name"="HBCm_U30_14", "active"=1, "physicalQuantity"={"type"="A"}}, {"name"="HBCm_U30_15", "active"=1, "physicalQuantity"={"type"="A"}}, {"name"="HBCm_U30_16", "active"=1, "physicalQuantity"={"type"="A"}}, {"name"="HBCm_U30_17", "active"=1, "physicalQuantity"={"type"="A"}}, {"name"="HBCm_U30_18", "active"=1, "physicalQuantity"={"type"="A"}}, {"name"="HBCm_U30_19", "active"=1, "physicalQuantity"={"type"="A"}}, {"name"="HBCm_U30_20", "active"=1, "physicalQuantity"={"type"="A"}}, {"name"="HBCm_U30_21", "active"=1, "physicalQuantity"={"type"="A"}}, {"name"="HBCm_U30_22", "active"=1, "physicalQuantity"={"type"="A"}}, {"name"="HBCm_U30_23", "active"=1, "physicalQuantity"={"type"="A"}}, {"name"="HBCm_U30_24", "active"=1, "physicalQuantity"={"type"="A"}}, {"name"="HBCm_U30_25", "active"=1, "physicalQuantity"={"type"="A"}}, {"name"="HBCm_U30_26", "active"=1, "physicalQuantity"={"type"="A"}}, {"name"="HBCm_U30_27", "active"=1, "physicalQuantity"={"type"="A"}}, {"name"="HBCm_U30_28", "active"=1, "physicalQuantity"={"type"="A"}}, {"name"="HBCm_U30_29", "active"=1, "physicalQuantity"={"type"="A"}}, {"name"="HBCm_U30_30", "active"=1, "physicalQuantity"={"type"="A"}}, {"name"="HBCm_U30_31", "active"=1, "physicalQuantity"={"type"="A"}}, {"name"="HBCm_U30_32", "active"=1, "physicalQuantity"={"type"="A"}}, {"name"="VBCm_V21_01", "active"=1, "physicalQuantity"={"type"="A"}}, {"name"="VBCm_V21_02", "active"=1, "physicalQuantity"={"type"="A"}}, {"name"="VBCm_V21_03", "active"=1, "physicalQuantity"={"type"="A"}}, {"name"="VBCm_V21_04", "active"=1, "physicalQuantity"={"type"="A"}}, {"name"="VBCm_V21_05", "active"=1, "physicalQuantity"={"type"="A"}}, {"name"="VBCm_V21_06", "active"=1, "physicalQuantity"={"type"="A"}}, {"name"="VBCm_V21_07", "active"=1, "physicalQuantity"={"type"="A"}}, {"name"="VBCm_V21_08", "active"=1, "physicalQuantity"={"type"="A"}}, {"name"="VBCm_V21_09", "active"=1, "physicalQuantity"={"type"="A"}}, {"name"="VBCm_V21_10", "active"=1, "physicalQuantity"={"type"="A"}}, {"name"="VBCm_V21_11", "active"=1, "physicalQuantity"={"type"="A"}}, {"name"="VBCm_V21_12", "active"=1, "physicalQuantity"={"type"="A"}}, {"name"="VBCm_V21_13", "active"=1, "physicalQuantity"={"type"="A"}}, {"name"="VBCm_V21_14", "active"=1, "physicalQuantity"={"type"="A"}}, {"name"="VBCm_V21_15", "active"=1, "physicalQuantity"={"type"="A"}}, {"name"="VBCm_V21_16", "active"=1, "physicalQuantity"={"type"="A"}}, {"name"="VBCm_V21_17", "active"=1, "physicalQuantity"={"type"="A"}}, {"name"="VBCm_V21_18", "active"=1, "physicalQuantity"={"type"="A"}}, {"name"="VBCm_V21_19", "active"=1, "physicalQuantity"={"type"="A"}}, {"name"="VBCm_V21_20", "active"=1, "physicalQuantity"={"type"="A"}}, {"name"="VBCm_V21_21", "active"=1, "physicalQuantity"={"type"="A"}}, {"name"="VBCm_V21_22", "active"=1, "physicalQuantity"={"type"="A"}}, {"name"="VBCm_V21_23", "active"=1, "physicalQuantity"={"type"="A"}}, {"name"="VBCm_V21_24", "active"=1, "physicalQuantity"={"type"="A"}}, {"name"="VBCm_V21_25", "active"=1, "physicalQuantity"={"type"="A"}}, {"name"="VBCm_V21_26", "active"=1, "physicalQuantity"={"type"="A"}}, {"name"="VBCm_V21_27", "active"=1, "physicalQuantity"={"type"="A"}}, {"name"="VBCm_V21_28", "active"=1, "physicalQuantity"={"type"="A"}}, {"name"="VBCm_V21_29", "active"=1, "physicalQuantity"={"type"="A"}}, {"name"="VBCm_V21_30", "active"=1, "physicalQuantity"={"type"="A"}}, {"name"="VBCm_V21_31", "active"=1, "physicalQuantity"={"type"="A"}}, {"name"="VBCm_V21_32", "active"=1, "physicalQuantity"={"type"="A"}}, {"name"="VBCm_V21_33", "active"=1, "physicalQuantity"={"type"="A"}}, {"name"="VBCm_V21_34", "active"=1, "physicalQuantity"={"type"="A"}}, {"name"="VBCm_V21_35", "active"=1, "physicalQuantity"={"type"="A"}}, {"name"="VBCm_V21_36", "active"=1, "physicalQuantity"={"type"="A"}}, {"name"="VBCm_V21_37", "active"=1, "physicalQuantity"={"type"="A"}}, {"name"="VBCm_V21_38", "active"=1, "physicalQuantity"={"type"="A"}}, {"name"="VBCm_V21_39", "active"=1, "physicalQuantity"={"type"="A"}}, {"name"="VBCm_V21_40", "active"=1, "physicalQuantity"={"type"="A"}}, {"name"="VBCs_V21_01", "active"=1, "physicalQuantity"={"type"="A"}}, {"name"="VBCs_V21_02", "active"=1, "physicalQuantity"={"type"="A"}}, {"name"="VBCs_V21_03", "active"=1, "physicalQuantity"={"type"="A"}}, {"name"="VBCs_V21_04", "active"=1, "physicalQuantity"={"type"="A"}}, {"name"="VBCs_V21_05", "active"=1, "physicalQuantity"={"type"="A"}}, {"name"="VBCs_V21_06", "active"=1, "physicalQuantity"={"type"="A"}}, {"name"="VBCs_V21_07", "active"=1, "physicalQuantity"={"type"="A"}}, {"name"="VBCs_V21_08", "active"=1, "physicalQuantity"={"type"="A"}}, {"name"="HBCs_U30_01", "active"=1, "physicalQuantity"={"type"="A"}}, {"name"="HBCs_U30_02", "active"=1, "physicalQuantity"={"type"="A"}}, {"name"="HBCs_U30_03", "active"=1, "physicalQuantity"={"type"="A"}}, {"name"="HBCs_U30_04", "active"=1, "physicalQuantity"={"type"="A"}}, {"name"="HBCs_U30_05", "active"=1, "physicalQuantity"={"type"="A"}}, {"name"="HBCs_U30_06", "active"=1, "physicalQuantity"={"type"="A"}}, {"name"="HBCs_U30_07", "active"=1, "physicalQuantity"={"type"="A"}}, {"name"="HBCs_U30_08", "active"=1, "physicalQuantity"={"type"="A"}}, {"name"="HBCs_U30_09", "active"=1, "physicalQuantity"={"type"="A"}}, {"name"="HBCs_U30_10", "active"=1, "physicalQuantity"={"type"="A"}}, {"name"="HBCs_U30_11", "active"=1, "physicalQuantity"={"type"="A"}}, {"name"="HBCs_U30_12", "active"=1, "physicalQuantity"={"type"="A"}}, {"name"="HBCs_U30_13", "active"=1, "physicalQuantity"={"type"="A"}}, {"name"="HBCs_U30_14", "active"=1, "physicalQuantity"={"type"="A"}}, {"name"="HBCs_U30_15", "active"=1, "physicalQuantity"={"type"="A"}}, {"name"="HBCs_U30_16", "active"=1, "physicalQuantity"={"type"="A"}}, {"name"="Test96", "active"=1, "physicalQuantity"={"type"="A"}}, {"name"="Test97", "active"=0, "physicalQuantity"={"type"=""}}]
  out "chanDescs_ArrayClust":T29(array[cluster])=[{"chanDescs"=[{"name"="E_Chan_1", "active"=1}, {"name"="E_Chan_2", "active"=1}, {"name"="E_Chan_3", "active"=1}, {"name"="E_Chan_4", "active"=1}, {"name"="E_Chan_5", "active"=1}, {"name"="E_Chan_6", "active"=1}, {"name"="E_Chan_7", "active"=1}, {"name"="E_Chan_8", "active"=1}, {"name"="E_Chan_9", "active"=1}, {"name"="E_Chan_10", "active"=1}, {"name"="E_Chan_11", "active"=1}, {"name"="E_Chan_12", "active"=1}, {"name"="E_Chan_13", "active"=1}, {"name"="E_Chan_14", "active"=1}, {"name"="E_Chan_15", "active"=1}, {"name"="E_Chan_16", "active"=1}, {"name"="E_Chan_17", "active"=1}, {"name"="E_Chan_18", "active"=1}, {"name"="E_Chan_19", "active"=1}, {"name"="E_Chan_20", "active"=1}, {"name"="E_Chan_21", "active"=1}, {"name"="E_Chan_22", "active"=1}, {"name"="E_Chan_23", "active"=1}, {"name"="E_Chan_24", "active"=1}, {"name"="E_Chan_25", "active"=1}, {"name"="E_Chan_26", "active"=1}, {"name"="E_Chan_27", "active"=1}, {"name"="E_Chan_28", "active"=1}, {"name"="E_Chan_29", "active"=1}, {"name"="E_Chan_30", "active"=1}, {"name"="E_Chan_31", "active"=1}, {"name"="E_Chan_32", "active"=1}, {"name"="E_Chan_33", "active"=1}, {"name"="E_Chan_34", "active"=1}, {"name"="E_Chan_35", "active"=1}, {"name"="E_Chan_36", "active"=1}, {"name"="E_Chan_37", "active"=1}, {"name"="E_Chan_38", "active"=1}, {"name"="E_Chan_39", "active"=1}, {"name"="E_Chan_40", "active"=1}, {"name"="E_Chan_41", "active"=1}, {"name"="E_Chan_42", "active"=1}, {"name"="E_Chan_43", "active"=1}, {"name"="E_Chan_44", "active"=1}, {"name"="E_Chan_45", "active"=1}, {"name"="E_Chan_46", "active"=1}, {"name"="E_Chan_47", "active"=1}, {"name"="E_Chan_48", "active"=1}, {"name"="E_Chan_49", "active"=1}, {"name"="E_Chan_50", "active"=1}, {"name"="E_Chan_51", "active"=1}, {"name"="E_Chan_52", "active"=1}, {"name"="E_Chan_53", "active"=1}, {"name"="E_Chan_54", "active"=1}, {"name"="E_Chan_55", "active"=1}, {"name"="E_Chan_56", "active"=1}, {"name"="E_Chan_57", "active"=1}, {"name"="E_Chan_58", "active"=1}, {"name"="E_Chan_59", "active"=1}, {"name"="E_Chan_60", "active"=1}, {"name"="E_Chan_61", "active"=1}, {"name"="E_Chan_62", "active"=1}, {"name"="E_Chan_63", "active"=1}, {"name"="E_Chan_64", "active"=1}, {"name"="E_Chan_65", "active"=1}, {"name"="E_Chan_66", "active"=1}, {"name"="E_Chan_67", "active"=1}, {"name"="E_Chan_68", "active"=1}, {"name"="E_Chan_69", "active"=1}, {"name"="E_Chan_70", "active"=1}, {"name"="E_Chan_71", "active"=1}, {"name"="E_Chan_72", "active"=1}, {"name"="E_Chan_73", "active"=1}, {"name"="E_Chan_74", "active"=1}, {"name"="E_Chan_75", "active"=1}, {"name"="E_Chan_76", "active"=1}, {"name"="E_Chan_77", "active"=1}, {"name"="E_Chan_78", "active"=1}, {"name"="E_Chan_79", "active"=1}, {"name"="E_Chan_80", "active"=1}, {"name"="E_Chan_81", "active"=1}, {"name"="E_Chan_82", "active"=1}, {"name"="E_Chan_83", "active"=1}, {"name"="E_Chan_84", "active"=1}, {"name"="E_Chan_85", "active"=1}, {"name"="E_Chan_86", "active"=1}, {"name"="E_Chan_87", "active"=1}, {"name"="E_Chan_88", "active"=1}, {"name"="E_Chan_89", "active"=1}, {"name"="E_Chan_90", "active"=1}, {"name"="E_Chan_91", "active"=1}, {"name"="E_Chan_92", "active"=1}, {"name"="E_Chan_93", "active"=1}, {"name"="E_Chan_94", "active"=1}, {"name"="E_Chan_95", "active"=1}, {"name"="E_Chan_96", "active"=1}, {"name"="E_Chan_97", "active"=1}, {"name"="E_Chan_98", "active"=1}, {"name"="E_Chan_99", "active"=1}, {"name"="E_Chan_100", "active"=1}, {"name"="E_Chan_101", "active"=1}, {"name"="E_Chan_102", "active"=1}, {"name"="E_Chan_103", "active"=1}, {"name"="E_Chan_104", "active"=1}, {"name"="E_Chan_105", "active"=1}, {"name"="E_Chan_106", "active"=1}, {"name"="E_Chan_107", "active"=1}, {"name"="E_Chan_108", "active"=1}, {"name"="E_Chan_109", "active"=1}, {"name"="E_Chan_110", "active"=1}, {"name"="E_Chan_111", "active"=1}, {"name"="E_Chan_112", "active"=1}, {"name"="E_Chan_113", "active"=1}, {"name"="E_Chan_114", "active"=1}, {"name"="E_Chan_115", "active"=1}, {"name"="E_Chan_116", "active"=1}, {"name"="E_Chan_117", "active"=1}, {"name"="E_Chan_118", "active"=1}, {"name"="E_Chan_119", "active"=1}, {"name"="E_Chan_120", "active"=1}, {"name"="E_Chan_121", "active"=1}, {"name"="E_Chan_122", "active"=1}, {"name"="E_Chan_123", "active"=1}, {"name"="E_Chan_124", "active"=1}, {"name"="E_Chan_125", "active"=1}, {"name"="E_Chan_126", "active"=1}, {"name"="E_Chan_127", "active"=1}, {"name"="E_Chan_128", "active"=1}]}]
  out "Bolo_HBCmPrad JSON":string
  out "DimensionA2":u32
  out "Bolo_VBCPradJson":string
  out "RT_P_rad Json":string
  out "BoloSignalJSON 2":string
  out "variables cluster":T30
  out "RangeIndex":u8[](array[numeric])
  out "DACbits 2":u16[](array[numeric])
  out "x*2^n":sgl[](array[numeric])
  in  "input DAC settings":i64[](array[numeric])=[3, 3, 3, 3, 3, 3, 3, 3, 3, 3, 3, 3, 3, 3, 3, 3, 3, 3, 3, 3, 3, 3, 3, 3, 3, 3, 3, 3, 3, 3, 3, 3, 3, 3, 3, 3, 3, 3, 3, 3, 3, 3, 3, 3, 3, 3, 3, 3, 3, 3, 3, 3, 3, 3, 3, 3, 3, 3, 3, 3, 3, 3, 3, 3, 3, 3, 3, 3, 3, 3, 3, 3, 3, 3, 3, 3, 3, 3, 3, 3, 3, 3, 3, 3, 3, 3, 3, 3, 3, 3, 3, 3, 3, 3, 3, 3, 3, 3, 3, 3, 3, 3, 3, 3, 3, 3, 3, 3, 3, 3, 3, 3, 3, 3, 3, 3, 3, 3, 3, 3, 3, 3, 3, 3, 3, 3, 0, 0]
  out "full DAC\nfile input":i64[][](array[numeric])=[[3], [3], [3], [3], [3], [3], [3], [3], [3], [3], [3], [3], [3], [3], [3], [3], [3], [3], [3], [3], [3], [3], [3], [3], [3], [3], [3], [3], [3], [3], [3], [3], [3], [3], [3], [3], [3], [3], [3], [3], [3], [3], [3], [3], [3], [3], [3], [3], [3], [3], [3], [3], [3], [3], [3], [3], [3], [3], [3], [3], [3], [3], [3], [3], [3], [3], [3], [3], [3], [3], [3], [3], [3], [3], [3], [3], [3], [3], [3], [3], [3], [3], [3], [3], [3], [3], [3], [3], [3], [3], [3], [3], [3], [3], [3], [3], [3], [3], [3], [3], [3], [3], [3], [3], [3], [3], [3], [3], [3], [3], [3], [3], [3], [3], [3], [3], [3], [3], [3], [3], [3], [3], [3], [3], [3], [3]]
  out "DAC settings":i64[](array[numeric])=[3, 3, 3, 3, 3, 3, 3, 3, 3, 3, 3, 3, 3, 3, 3, 3, 3, 3, 3, 3, 3, 3, 3, 3, 3, 3, 3, 3, 3, 3, 3, 3, 3, 3, 3, 3, 3, 3, 3, 3, 3, 3, 3, 3, 3, 3, 3, 3, 3, 3, 3, 3, 3, 3, 3, 3, 3, 3, 3, 3, 3, 3, 3, 3, 3, 3, 3, 3, 3, 3, 3, 3, 3, 3, 3, 3, 3, 3, 3, 3, 3, 3, 3, 3, 3, 3, 3, 3, 3, 3, 3, 3, 3, 3, 3, 3, 3, 3, 3, 3, 3, 3, 3, 3, 3, 3, 3, 3, 3, 3, 3, 3, 3, 3, 3, 3, 3, 3, 3, 3, 3, 3, 3, 3, 3, 3, 0, 0]
  out "size(s)":i32
  in  "DAC settings file location":path=path "C:/Users/Administrator/Desktop/dac_settings.dat"
  out "volume element":sgl
  out "channel selected":i64
  out "iterator":i32
  out "V_Cam":dbl
  in  "Path to kbolott and volume data file":path=path "C:/Users/Administrator/Desktop/kbolott_and_volume_all_PV_new.dat"
  in  "Read geometry from file?":bool
  out "kbolott_and_volume":dbl[][](array[numeric])=[[1e-05, 1e-05], [9.8364458e-05, 1.8160732], [0.00029863964, 770.25441], [0.00053910452, 1653.5432], [0.00071569496, 2554.7619], [0.00083348142, 3356.1809], [0.00092645429, 4021.9678], [0.00099241932, 4570.4466], [0.0010332482, 4989.6792], [0.0010552469, 5170.4882], [0.0010669981, 5192.5645], [0.001071534, 5152.6222], [0.0010766644, 5109.6704], [0.0010841289, 5094.9972], [0.0010884845, 5078.237], [0.0010888843, 5058.9416], [0.0010882289, 5056.581], [0.0010872861, 5078.1684], [0.0010832221, 5096.5196], [0.0010760805, 5113.7904], [0.0010685167, 5141.4566], [0.0010644166, 5189.7831], [0.0010539441, 5182.7365], [0.0010337779, 5034.6928], [0.00098716411, 4625.8518], [0.00091599422, 4090.3707], [0.00082376071, 3438.9665], [0.00070194108, 2659.5109], [0.00051785958, 1753.3355], [0.00030745544, 937.82125], [0.00014081292, 59.55205], [1e-05, 1e-05], [0.0, 0.0], [0.0, 0.0], [0.0, 0.0], [0.0, 0.0], [0.0, 0.0], [0.0, 0.0], [0.0, 0.0], [0.0, 0.0], [0.0, 0.0], [0.0, 0.0], [0.0, 0.0], [0.0, 0.0], [0.0, 0.0], [0.0, 0.0], [0.0, 0.0], [0.0, 0.0], [0.0019134875, 3474.3085], [0.0020594744, 3690.1455], [0.002175929, 3861.3028], [0.0022530617, 3956.5918], [0.0023492529, 4057.9903], [0.0024581424, 4205.0841], [0.0025383764, 4324.9746], [0.0025876415, 4417.9525], [0.0026676725, 4566.0612], [0.0027635964, 4770.6296], [0.0028188521, 4914.295], [0.0028263806, 4970.0105], [0.0028491244, 5014.7926], [0.0028762033, 5060.279], [0.0028430703, 4969.1072], [0.0027058578, 4592.2853], [0.0019047772, 4936.5706], [0.0023594746, 6388.5028], [0.0025094117, 6336.5413], [0.002569351, 6048.9284], [0.0026367277, 5794.3031], [0.002714522, 5668.1597], [0.0027530637, 5505.217], [0.0027520905, 5312.6378], [0.0027781484, 5183.8321], [0.0028283925, 5165.5044], [0.0028425709, 5118.655], [0.00281436, 5016.5122], [0.0027996491, 4909.784], [0.0027993913, 4845.125], [0.0027603692, 4728.4661], [0.0026886073, 4585.7454], [0.0026437627, 4495.4419], [0.0026242501, 4486.7206], [0.0025685332, 4434.986], [0.0024747416, 4324.8822], [0.0023915919, 4209.8149], [0.002319616, 4111.844], [0.0022042921, 3923.4955], [0.0020485146, 3644.5259], [0.0024033884, 3597.1969], [0.002066694, 2566.1598], [0.0017718795, 1878.4004], [0.0015136288, 1414.3006], [0.0013043692, 1094.5581], [0.0011378765, 882.65731], [0.00097324167, 712.97006], [0.00080739571, 571.52867], [0.0, 0.0], [0.0, 0.0], [0.0, 0.0], [0.0, 0.0], [0.0, 0.0], [0.0, 0.0], [0.0, 0.0], [0.0, 0.0], [0.0, 0.0], [0.0, 0.0], [0.0, 0.0], [0.0, 0.0], [0.0, 0.0], [0.0, 0.0], [0.0, 0.0], [0.0, 0.0], [0.0, 0.0], [0.0, 0.0], [0.0, 0.0], [0.0, 0.0], [0.0, 0.0], [0.0, 0.0], [0.0, 0.0], [0.0, 0.0], [0.0, 0.0], [0.0, 0.0], [0.0, 0.0], [0.0, 0.0], [0.0, 0.0], [0.0, 0.0], [0.0, 0.0], [0.0, 0.0]]
  in  "VBCrPath":string="C:\\LABVIEW\\bolometer_labview\\NationalInstruments\\final\\BLV\\bolo_files\\standard_camVBCr_kbolott_and_volum_PV_new_.dat"
  in  "VBClPath":string="C:\\LABVIEW\\bolometer_labview\\NationalInstruments\\final\\BLV\\bolo_files\\standard_camVBCl_kbolott_and_volum_PV_new_.dat"
  in  "SavePath":string="C:\\LABVIEW\\bolometer_labview\\NationalInstruments\\final\\BLV\\bolo_files\\standard_cam_kbolott_and_volume_PV_new.dat"
  in  "HBCmPath":string="C:\\LABVIEW\\bolometer_labview\\NationalInstruments\\final\\BLV\\bolo_files\\standard_camHBCm_kbolott_and_volum_PV_new_.dat"
  out "Nsample array":dbl[](array[numeric])
  out "tau_fact":dbl[](array[numeric])
  out "F_ch":dbl[](array[numeric])
  in  "Tab Control 2":T31(tab)
  out "Offset 1-32":T4
  out "Offset 33-64":T3
  out "Offset 65 - 96":T6
  out "Offset 97 - 128":T5
  out "Mean (mV)":dbl[](array[numeric])=[-0.7403271408984438, -8.260093046352267, -8.918947572819889, -9.772275222465396, 0.30864745762664825, -0.6537256027804688, 79.99756187200546, 4.153005430940539, 7.643410503398627, -11.824992547743022, -14.697624578140676, 11.989870643243194, -8.775463779456913, 7.996481790207326, 8.106088914908469, -10.8637940203771, -12.059611966833472, 11.933022578246891, -6.146464895457029, -14.951843526214361, -0.002441406195430318, 6.242419389076531, 3.5611279467120767, 3.2575269085355103, 8.824575318954885, -7.361447674687952, -7.832151234149933, 7.266919030807912, -5.7468848787248135, 7.514682772103697, 5.840900921728462, -6.99057364044711, 79.99756187200546, -6.54301010677591, -9.606794172897935, 12.265525130555034, 12.906237763352692, -16.981191482394934, 13.987873554229736, -16.583854978904128, 1.392072725808248, 1.014677724102512, 2.4519091872498393, -2.9702612278051674, 15.86502225510776, -16.213782219216228, -15.602055666036904, 17.943933019414544, 3.8411009963601828, -9.436445392668247, 9.988481301814318, -6.0668189390562475, -1.9699560110457244, 4.278476700186729, -4.146425690501928, -5.190747133456171, -11.578285955823958, -5.565600541885942, -8.58544656727463, 6.866428219247609, -1.7924145732540637, -2.5657324735075235, -10.45345223788172, -6.23921628203243, 3.750788521952927, -18.172458792105317, -4.7267457586713135, 3.3571435594931245, -12.573710858821869, 9.11560804862529, 6.793176222126931, -3.880092795006931, 1.7657519394997507, -16.396104218438268, -10.506586869247258, 12.012434140779078, -8.395295393653214, 13.449138316325843, 17.604008730500937, -4.315998600330204, -3.6457983299624175, 5.335459100082517, 10.846701556816697, -4.911674967035651, -8.819763222709298, -8.540051245130599, -8.416257471777499, -5.678584035951644, -2.246835907921195, 2.759648502105847, 8.595751833170652, -7.270273599773645, 12.40836443938315, -12.00804919283837, -11.766723623499274, 9.407106788828969, -13.477368192747235, 12.26231449842453, 11.896674795076251, 0.723403328913264, 5.334943951573223, -8.783747594803572, -12.08735079318285, 14.564279926009476, 3.3106738957576454, -8.276560293510556, -8.709924166090786, 7.743080863263458, 1.6942675670143217, -0.2319506806670688, 1.5145385509822518, -5.742541505023837, -3.7815917376428843, -6.238308107946068, -5.504038091748953, -6.393525378312916, -6.460983901284635, -5.044728995766491, -5.857170409057289, -5.038603504188359, -6.4506298690102994, -5.754794927313924, -5.584150397218764, -7.321149886120111, -6.3962524347007275, -5.240952145308256, -5.635815440677106, 0.007434081865085318] format="%10.6f"
  out "Peak to Peak \n      (microV)":dbl[](array[numeric])=[4.882807843387127, 7.323920726776123, 4.882924258708954, 7.3248520493507385, 7.32421176508069, 14.64842353016138, 0.0, 9.765848517417908, 7.323920726776123, 7.3248520493507385, 4.882924258708954, 4.882924258708954, 7.323920726776123, 7.323920726776123, 4.882924258708954, 7.323920726776123, 4.882924258708954, 7.323920726776123, 7.324386388063431, 4.882924258708954, 0.0, 17.08976924419403, 4.882924258708954, 4.882924258708954, 7.323920726776123, 4.882924258708954, 9.764917194843292, 7.324386388063431, 12.206844985485077, 12.206844985485077, 7.324386388063431, 12.206844985485077, 0.0, 4.882458597421646, 4.882924258708954, 7.323920726776123, 7.3248520493507385, 7.323920726776123, 7.3248520493507385, 7.323920726776123, 7.324153557419777, 7.324269972741604, 7.324386388063431, 7.324386388063431, 7.323920726776123, 7.323920726776123, 14.647841453552246, 4.883855581283569, 7.324153557419777, 9.764917194843292, 7.323920726776123, 4.882924258708954, 4.8826914280653, 7.324386388063431, 9.765848517417908, 4.882924258708954, 7.323920726776123, 4.882458597421646, 7.323920726776123, 4.882458597421646, 4.882807843387127, 4.882924258708954, 7.3248520493507385, 21.972693502902985, 7.324153557419777, 7.323920726776123, 4.882924258708954, 7.324386388063431, 4.881992936134338, 4.881992936134338, 7.324386388063431, 7.324153557419777, 4.882807843387127, 4.881992936134338, 4.882924258708954, 4.882924258708954, 4.882924258708954, 4.881992936134338, 4.883855581283569, 4.882924258708954, 14.648539945483208, 7.324386388063431, 9.764917194843292, 7.323920726776123, 2.4419277906417847, 4.882924258708954, 4.882924258708954, 17.08976924419403, 4.882924258708954, 7.324153557419777, 4.882924258708954, 4.882924258708954, 7.323920726776123, 7.3248520493507385, 4.882924258708954, 4.882924258708954, 4.882924258708954, 7.3248520493507385, 4.882924258708954, 12.207019608467817, 7.324386388063431, 7.3248520493507385, 4.882924258708954, 7.323920726776123, 4.8826914280653, 4.882924258708954, 7.323920726776123, 7.323920726776123, 12.206961400806904, 4.882807843387127, 7.324153557419777, 83.00784975290298, 4.882924258708954, 100.09761899709702, 78.12539115548134, 78.12492549419403, 102.53908112645149, 75.68346336483955, 80.56638762354851, 122.0703125, 124.51177462935448, 80.56638762354851, 73.24246689677238, 90.33177047967911, 100.09761899709702, 124.51177462935448, 107.42153972387314, 4.882812390860636] format="%10.6f"
  out "StandardDeviation\n        (microV)":dbl[](array[numeric])=[1.3178064258400095, 1.3688848831831322, 1.0548084889226834, 1.2443223788848128, 1.59705142451057, 2.1744180062456038, 0.0, 2.030907639822008, 1.4483318171262458, 1.3229571557909583, 1.2288836017876232, 1.2019938667489987, 1.6031305992410694, 1.35056610905436, 1.2530645848264554, 1.31429956038145, 1.301997989212934, 1.3131709250589028, 1.2628189981428979, 1.2669901739210172, 0.0, 4.080886284109347, 1.2567152102849821, 1.4707879333305944, 1.3416244798708823, 1.2520654762466035, 1.1621411168699292, 1.6578588547989066, 1.938046373613482, 2.079945506020762, 1.4679482663126044, 2.4969349290910765, 0.0, 1.0377770470837968, 1.2053373518397679, 1.5233752130424645, 1.3873401592850336, 1.267911229300545, 1.7115725574627663, 1.672160871996824, 1.31871324161832, 1.5078466986453507, 1.3255947803386752, 1.3234413836801455, 1.4582847768773897, 1.5889487622848673, 2.6401680134333327, 1.5048596710786637, 1.4965932721457103, 2.11396581521971, 1.4492389700535926, 1.211021821317672, 1.088402229453829, 1.3027070893090829, 1.4943343873331378, 1.4711708684534495, 1.3873984679166236, 1.2231989233359766, 1.750523642577629, 1.3005922812196373, 1.1374552706732324, 1.1815869583592162, 1.4007793076850847, 4.196818432173733, 1.4374726206484196, 1.301960871939451, 1.4138890627406235, 1.2793913840230886, 1.1582161699882094, 1.2446473197964343, 1.2727841087979408, 1.481376523299904, 1.1972532239373488, 1.2198889335548715, 1.2546566558212389, 1.1531193277012952, 1.187455631517667, 1.3206467676139966, 1.281944644592881, 1.2570827474942263, 2.3910904638517647, 1.293707722094206, 1.7982859830900162, 1.3108731674959755, 1.207149905736413, 1.055707411180379, 1.2675066394274768, 3.273099711139876, 1.2863146235478906, 1.436305758467038, 1.122934834107274, 1.2029844769162397, 1.3032295933995295, 1.3235878742068965, 1.2342866127368863, 1.3107689142935, 1.2663205551311498, 1.2853884007170449, 1.1427512718670383, 1.947567144456653, 1.4146814196041755, 1.380297985065612, 1.2885583594980254, 1.3919624137077236, 1.266897046896499, 1.334428389718664, 1.3030643785056581, 1.2724759213760508, 2.1440161624517597, 0.9733550133977411, 1.3482751717255381, 15.274697451280197, 1.3247041442068581, 17.914749263968652, 13.28265778988492, 12.530637398975736, 19.41423181887618, 15.192128480144538, 14.38807309896394, 17.91942492957816, 18.58907441753092, 14.545750999364511, 14.751446890349179, 14.532230763324675, 18.646006130017184, 20.34445520211265, 19.670686718256125, 1.2376147585754236] format="%10.7f"
  out "Offsets":sgl[](array[numeric])=[-0.0007403271, -0.008260093, -0.008918948, -0.009772276, 0.00030864746, -0.0006537256, 0.07999756, 0.0041530053, 0.0076434105, -0.0118249925, -0.014697624, 0.011989871, -0.008775463, 0.007996482, 0.008106089, -0.010863794, -0.012059612, 0.011933022, -0.006146465, -0.014951844, -2.4414062e-06, 0.0062424196, 0.003561128, 0.003257527, 0.008824576, -0.007361448, -0.007832151, 0.007266919, -0.0057468847, 0.0075146826, 0.005840901, -0.006990574, 0.07999756, -0.00654301, -0.009606794, 0.012265525, 0.0129062375, -0.016981192, 0.013987874, -0.016583854, 0.0013920728, 0.0010146777, 0.0024519092, -0.0029702613, 0.015865022, -0.016213782, -0.015602056, 0.017943934, 0.003841101, -0.009436445, 0.009988481, -0.0060668187, -0.001969956, 0.004278477, -0.0041464255, -0.0051907473, -0.011578286, -0.0055656005, -0.0085854465, 0.006866428, -0.0017924146, -0.0025657325, -0.010453452, -0.0062392163, 0.0037507885, -0.01817246, -0.0047267457, 0.0033571436, -0.012573711, 0.009115608, 0.0067931763, -0.0038800929, 0.001765752, -0.016396103, -0.010506587, 0.012012434, -0.008395296, 0.013449138, 0.017604008, -0.0043159984, -0.0036457984, 0.005335459, 0.010846701, -0.004911675, -0.008819764, -0.008540051, -0.008416258, -0.005678584, -0.002246836, 0.0027596485, 0.008595752, -0.0072702738, 0.012408365, -0.0120080495, -0.011766723, 0.009407107, -0.013477368, 0.012262315, 0.0118966745, 0.00072340335, 0.005334944, -0.008783747, -0.012087351, 0.0145642795, 0.0033106739, -0.00827656, -0.008709924, 0.007743081, 0.0016942676, -0.00023195067, 0.0015145385, -0.0057425415, -0.0037815918, -0.0062383083, -0.005504038, -0.0063935253, -0.006460984, -0.005044729, -0.0058571706, -0.0050386037, -0.00645063, -0.005754795, -0.0055841506, -0.00732115, -0.0063962527, -0.005240952, -0.0056358157, 7.434082e-06]
  out "BoloSignalRaw Sizes (debug)":i32[](array[numeric])
  in  "Tab Control 5":T32(tab)
  out "MessCal 17-32":T33
  out "MessCal 1-16":T34
  out "MessCal 49 - 64":T35
  out "MessCal 33 - 49":T36
  out "MessCal 81 - 96":T37
  out "MessCal 65 - 80":T38
  out "MessCal 113 - 128":T39
  out "MessCal 97 - 112":T40
  out "RMESS":dbl[](array[numeric])=[964.4665558152926, 984.0412138536651, 1001.0627256989599, 1012.7898525309201, 986.7279110070629, 993.5830261423998, 1133.718466702734, 1026.065541032409, 981.7525515631839, 976.6051330676225, 975.1369773387203, 983.6003740876943, 945.3052421117454, 944.0131212191011, 937.9865397688445, 924.775520494105, 1002.3909240348048, 1016.474188810108, 1008.3024841336951, 997.8517562562979, 1396.1357804303618, 1011.7052948010587, 1006.0858095523904, 1000.525119034801, 1016.071205963885, 1008.5531713944379, 1001.2101495655734, 1012.9539707105694, 909.9522463978296, 921.8611396886308, 930.8535575645451, 937.6736260749049, 1835.253905213153, 905.3151174073253, 915.4686408360067, 932.2842954450018, 878.6376527118448, 888.8892103361444, 896.5962281010978, 917.195767017641, 953.2009542047422, 949.8476734916919, 945.7180214798805, 934.1303098026676, 944.4309270141721, 922.393020385211, 908.2770101975661, 902.8479184676862, 997.7185120044248, 1004.633250147941, 1012.2992174178987, 1022.8972656361334, 988.1138139759116, 1012.5096483256309, 926.7526927543831, 940.6499588809413, 987.4981539235332, 1030.6093168535383, 996.69488158787, 998.6770565199763, 937.2653710614366, 942.0245103372197, 975.0990877775471, 954.8089604337308, 987.3564837474132, 941.2547128561528, 982.5095895382428, 979.0417371038707, 995.2373497220817, 994.8506309175264, 989.7979732647505, 986.9344569144992, 979.4724674608722, 951.8026661804106, 928.3096097998925, 980.4648125251251, 967.8736951300871, 960.399052288677, 950.3474867516031, 931.7877057694141, 925.6104123406642, 925.2905333073797, 925.2586242376997, 996.0089625341668, 969.8590336679081, 973.5395443351913, 978.7443359479869, 1329.6132687126426, 951.8837808548863, 946.7262849537287, 933.7058147126331, 940.8228530266879, 876.367589172054, 864.1420943242144, 855.6188139335973, 854.7591574173059, 955.1936774096923, 969.1826763753277, 970.8033011923455, 0.0, 935.2179320514933, 937.6581182076873, 940.1867678977421, 939.4080093580444, 850.4194498630884, 857.7406858104588, 867.3881837894808, 884.270800315495, 892.6618762043922, 899.3995556852765, 915.5186423922648, 0.0, 919.5685811076437, 0.0, 0.0, 0.0, 0.0, 0.0, 0.0, 0.0, 0.0, 0.0, 0.0, 0.0, 0.0, 0.0, 0.0, 0.0]
  out "KappaM":dbl[](array[numeric])=[0.0008396193201719739, 0.0008193409803026575, 0.0008327489337370494, 0.0008094925878469488, 0.00089368, 0.0008063058560714545, 0.0008451910365158945, 0.0007992358755606012, 0.0008323076933152601, 0.0008570762215527662, 0.0007628861690345087, 0.0008061906602308296, 0.0008540424353779365, 0.0008301118976821594, 0.0008577435335519969, 0.0008553747566925557, 0.000838644207815748, 0.0008273548270536888, 0.0008111923709406437, 0.0008317040544888235, 0.0002062919117538751, 0.0007971782754034694, 0.0007777938427968141, 0.0007983063012770449, 0.0007902138174646686, 0.0007777700527572154, 0.0008086241703327105, 0.0007894905085128677, 0.0008499052168857277, 0.0008231536154986703, 0.0008290108212352768, 0.0008015771948583539, 0.0004219784890145567, 0.0008028223447312654, 0.0007908997677950409, 0.0007688640721813007, 0.0007923143974006498, 0.0007943700234243013, 0.000794807683089336, 0.0007644407575630641, 0.0008256914284962689, 0.0008464663657085921, 0.0008525498714753285, 0.0008605939917038706, 0.0008075301142063146, 0.0008582080819176783, 0.0008833831995156997, 0.0008817750426330745, 0.0008736825873144331, 0.0008712555197947145, 0.0008599116319459445, 0.0008597288697454142, 0.0008850439198466119, 0.0008360600624626481, 0.0008729149198757765, 0.0008652970161905564, 0.000878176403644396, 0.000814669724061475, 0.0008492936703496222, 0.0008335090067364612, 0.0009020306039280142, 0.0009060889736233363, 0.000873120149823901, 0.0008865804075398461, 0.0008218319952538781, 0.0008647381541051004, 0.0008535415687509321, 0.000868609807906937, 0.0008544506047017487, 0.0008552184337763689, 0.0008772351584693919, 0.0008899531428744609, 0.0009049492537694576, 0.000908105157129488, 0.0009441675693280472, 0.0008666158415307141, 0.0008904383660716827, 0.00090533600441176, 0.0009193630525411423, 0.0009209094258700529, 0.0008671616817531277, 0.0008573033056411677, 0.0008894545060438134, 0.0008393076570230061, 0.0008809839906701387, 0.0008713273912310079, 0.0008529389904228485, 0.0008798583497112145, 0.0007606961064025662, 0.0007618681674480262, 0.0008830002472907413, 0.0008434447500347438, 0.0008157810403546725, 0.0008170412330426688, 0.000817539692314199, 0.0008060567476264818, 0.0007745714382802376, 0.0007738842512393123, 0.0007910139604008742, -1.9640688433259297e-10, 0.000780575223559956, 0.0007962779122750964, 0.000790630439080113, 0.0008189866992119251, 0.0008220353590981327, 0.0008259174124746273, 0.0008237041516630779, 0.0008128375228315313, 0.0008025139618430593, 0.0007891459070721132, 0.0007835394415130632, 1.4659311061625464e-11, 0.0007713911232202254, -1.136328152026204e-11, 7.33972615530204e-11, -5.807996136265078e-12, 1.50989391544806e-10, -2.091237015882531e-11, -2.2968171315336452e-11, 3.2003514158147334e-12, -1.18410213996469e-13, 3.9907860061368183e-13, 1.2900003061146403e-11, -7.996494711993759e-11, 1.2728268766879732e-10, -2.7124534936566837e-11, -1.0618681361847593e-11, 1.1300143559461795e-05] format="%10.4e"
  out "TauM":dbl[](array[numeric])=[0.11537597448635277, 0.11755685958822219, 0.1164214694473907, 0.11697577239117866, 0.3604506191165193, 0.12010942076824872, 0.11766714993048435, 0.11910426529905502, 0.10999582403545866, 0.11118469600664964, 0.10580731993585431, 0.11217289808087993, 0.11223398365603839, 0.11204749607224823, 0.11263624992738425, 0.11091290284745299, 0.11721868902521211, 0.11737061531613151, 0.11788987597885038, 0.11600007869942867, 0.11334307549251021, 0.11228572042130423, 0.1129521332802642, 0.11724104097990388, 0.11740306056822605, 0.11529467898123245, 0.11828175507687082, 0.11829012392284373, 0.11773460668621359, 0.1155776803231521, 0.11650421728110884, 0.11571658330095998, 0.11068789319935994, 0.10986016888144867, 0.10999340462233435, 0.11095550249493497, 0.11143937038853975, 0.11095468517729823, 0.11130783288802211, 0.11084408945769118, 0.10830137260394793, 0.10662335345199567, 0.10535002662491703, 0.10738515206651872, 0.10772145508062766, 0.1053368317440755, 0.10408446186375701, 0.10449038510758271, 0.11178895597256559, 0.11021628063681403, 0.11220331344682449, 0.11111721341359461, 0.10889811436206044, 0.11638094730098773, 0.11290278568076087, 0.11205006536853761, 0.1094907553786962, 0.11634433136641531, 0.11037702264320227, 0.1104223688763365, 0.11352480237507033, 0.11341744936097128, 0.10916961452972393, 0.11332789199343518, 0.11107001747086552, 0.1083853978889723, 0.11029711206697901, 0.11063487469805744, 0.10926615257922916, 0.10988377001368325, 0.10782095764307568, 0.1073886205272185, 0.10829341805096283, 0.10953345610425252, 0.10953147401563214, 0.10933747673483066, 0.1093210854374169, 0.10892908051404164, 0.10841565534876087, 0.10934867623657209, 0.11431979794745441, 0.11469548527952493, 0.11256319960938391, 0.11004758193350624, 0.1086775698186096, 0.10860163257332957, 0.10972644811806966, 0.1244329993560779, 0.10848514148619942, 0.10753497988240919, 0.11378450261362759, 0.11397799701939393, 0.10865166632049855, 0.10955778865143037, 0.11184264538711042, 0.11080028199806266, 0.11230419705417591, 0.11150150302047147, 0.10940920103499238, 0.0, 0.11018788195565775, 0.1109851624674225, 0.10888498891279576, 0.10950524535111039, 0.11209787924272374, 0.11180887164622381, 0.1110290995583749, 0.11040609393156747, 0.1103438351320269, 0.1101975468642728, 0.10923728746964355, 0.0, 0.11021638606642407, 0.0, 0.0, 0.0, 0.0, 0.0, 0.0, 0.0, 0.5609466646481899, 0.0, 0.0, 0.0, 0.0, 0.0, 0.0, 0.4058686463981613] format="%10.4f"
  in  "Tab Control 3":T32(tab)=enum."97 to 128"
  out "RefCal 17-32":T33
  out "RefCal 1-16":T34
  out "RefCal 49 - 64":T35
  out "RefCal 33 - 48":T36
  out "RefCal 65 - 80":T38
  out "RefCal 81 - 96":T37
  out "RefCal 113 - 128":T39
  out "RefCal 97 - 112":T40
  out "TauR":dbl[](array[numeric]) caption="TauM" format="%10.4f"
  out "KappaR":dbl[](array[numeric]) format="%10.4e"
  out "RREF":dbl[](array[numeric])
  in  "stop":bool
  out "Acquired Samples:":u32(slide) scale=-1.0..26000.0
  out "state":string="Wait for Start"
  # "Largest Offset ~ 20 mV; 40 mV Range should work for all channels"
  # "Sample Rate Settings"
  # "FilterSelection"
  # "Epoch POSIX time from start of VI"
  # "Set manual time above"
  # "Get last trigger from  http://sv-coda-wsvc-3/last_trigger"
  # "Get UTC Time not working"
  # "WENDELSTEIN - 7-X Bolometer DAQ System                 v1741"
  # "v2018@pih"
  # "DAC Range shown for check:"
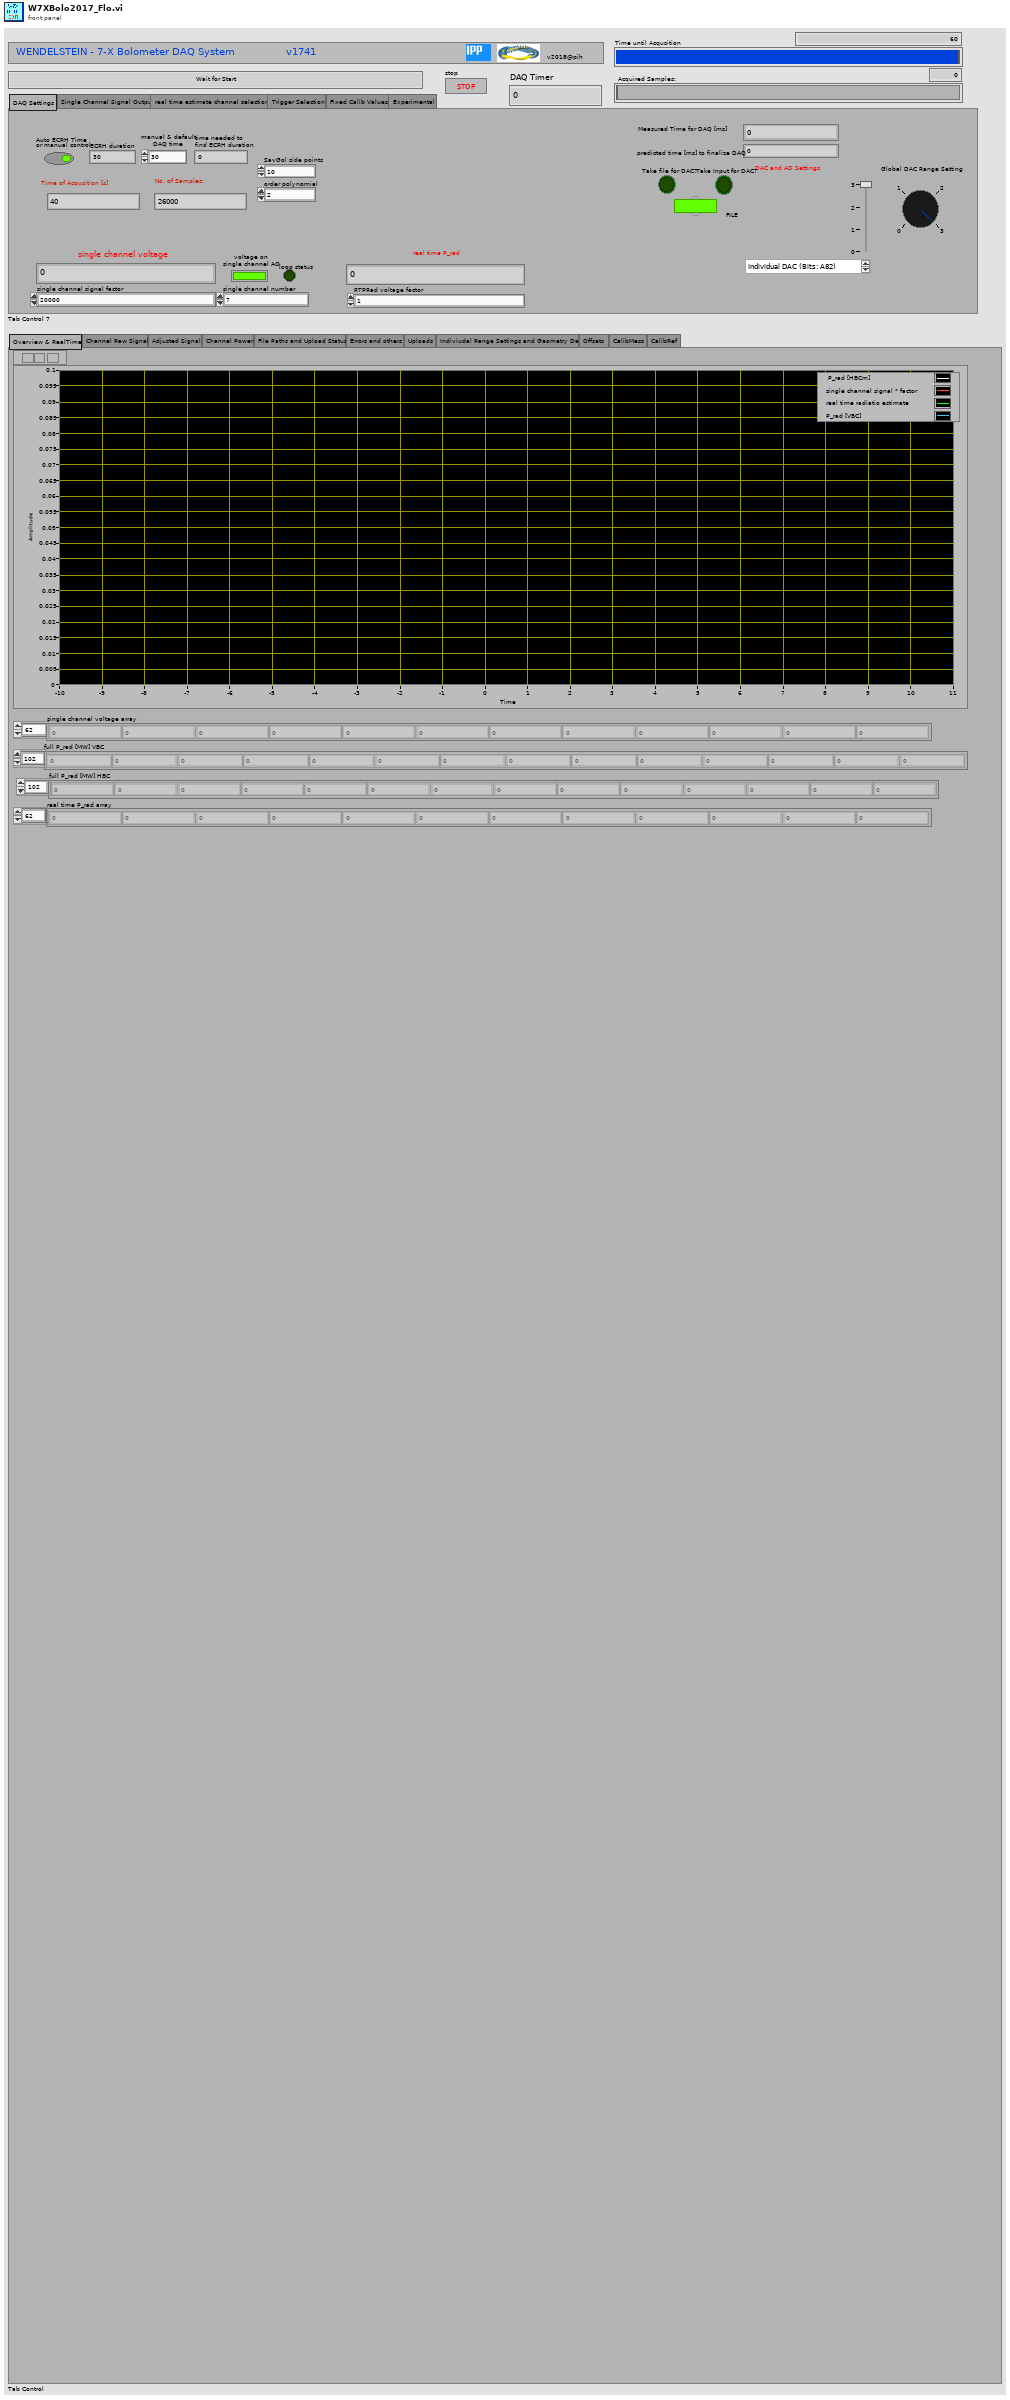
[diagram p1: front panel]
types:
  T1 = enum32{"DAQ Settings", "Single Channel Signal Output", "real time estimate channel selection", "Trigger Selection", "Fixed Calib Values", "Experimental"}
  T2 = enum32{"Overview & RealTime", "Channel Raw Signal", "Adjusted Signal", "Channel Power", "File Paths and Upload Status", "Errors and others", "Uploads", "Indiviudal Range Settings and Geometry Data", "Offsets", "CalibMess", "CalibRef"}
  T3 = cluster{"Channels 33 - 40":cluster{"tstart":dbl, "FPGSampleTime":dbl, dbl[][]}, "Channels 41 - 48":cluster{"tstart":dbl, "FPGSampleTime":dbl, dbl[][]}, "Channels 49 - 56":cluster{"tstart":dbl, "FPGSampleTime":dbl, dbl[][]}, "Channels 57 - 64":cluster{"tstart":dbl, "FPGSampleTime":dbl, dbl[][]}}
  T4 = cluster{"Channels 1- 8":cluster{"tstart":dbl, "FPGSampleTime":dbl, dbl[][]}, "Channels 9 - 16":cluster{"tstart":dbl, "FPGSampleTime":dbl, dbl[][]}, "Channels 17 - 24":cluster{"tstart":dbl, "FPGSampleTime":dbl, dbl[][]}, "Channels 25 - 32":cluster{"tstart":dbl, "FPGSampleTime":dbl, dbl[][]}}
  T5 = cluster{"Channels 97 - 104":cluster{"tstart":dbl, "FPGSampleTime":dbl, dbl[][]}, "Channels 105 - 112":cluster{"tstart":dbl, "FPGSampleTime":dbl, dbl[][]}, "Channels 113 - 120":cluster{"tstart":dbl, "FPGSampleTime":dbl, dbl[][]}, "Channels 121 - 128":cluster{"tstart":dbl, "FPGSampleTime":dbl, dbl[][]}}
  T6 = cluster{"Channels 65 - 71":cluster{"tstart":dbl, "FPGSampleTime":dbl, dbl[][]}, "Channels 73 - 80":cluster{"tstart":dbl, "FPGSampleTime":dbl, dbl[][]}, "Channels 81 - 88":cluster{"tstart":dbl, "FPGSampleTime":dbl, dbl[][]}, "Channels 89- 96":cluster{"tstart":dbl, "FPGSampleTime":dbl, dbl[][]}}
  T7 = cluster{"Nsample array":dbl[], "full P_rad [MW] HBC":dbl[]}
  T8 = enum32{"BoloAdjusted ErrorOut", "Parlog", "Datastream"}
  T9 = enum32{"RT_P_rad ErrorOut", "Parlog", "Datastream"}
  T10 = enum32{"QSB parms ErrorOut", "Parlog", "Datastream"}
  T11 = enum32{"CalibMeasFoilFit ErrorOut", "Parlog", "Datastream"}
  T12 = enum32{"RKappa ErrorOut", "Parlog", "Datastream"}
  T13 = enum32{"BoloPowerRaw ErrorOut", "Parlog", "Datastream"}
  T14 = enum32{"CalibMeasFoilCurrent ErrorOut", "Parlog", "Datastream"}
  T15 = enum32{"BoloSignal ErrorOut", "Parlog", "Datastream"}
  T16 = enum32{"CalibRefFoilCurrent ErrorOut", "Parlog", "Datastream"}
  T17 = enum32{"BoloCalibRefFoilFit ErrorOut", "Parlog", "Datastream"}
  T18 = enum32{"Offset ErrorOut", "Parlog", "Datastream"}
  T19 = enum32{"MKappa ErrorOut", "Parlog", "Datastream"}
  T20 = enum32{"ChannelSelection ErrorOut", "Parlog", "Datastream"}
  T21 = cluster{"name":string, "active":i32, "physicalQuantity":cluster{"type":string}}[]
  T22 = enum32{"VBCPrad ErrorOut", "Parlog", "Datastream"}
  T23 = enum32{"SingleChannelFeedback ErrorOut", "Parlog", "Datastream"}
  T24 = enum32{"HBCmPrad ErrorOut", "Parlog", "Datastream"}
  T25 = cluster{"sample_period":dbl, "sample_rate":dbl, "pulse_length":dbl, "detector":string, "Nchannels":i16, "ADCbits":i16, "BridgeVoltage (V)":sgl, "DAC Range Setting":u8, "AD 7730 Bit Settings":i32, "DAC and AD Settings":i32, "chanDescs":cluster{"name":string, "active":i32, "physicalQuantity":cluster{"type":string}}[], "start time":i64, "Pre-start time (ms) of DAQ Typically set to 1000 ms":i32, "Measured Time for DAQ [ms] ":u32, "single channel number":i64, "maximum voltage @ 10MW single channel":dbl, "ExptSampleFrequency (Hz)":sgl, "single channel voltage factor":dbl, "CalibSampleFrequency (Hz)":sgl, "predicted time [ms] to finalize DAQ":dbl, "CalStep1 (V)":string, "CalStep2 (V)":string, "data string":string}[]
  T26 = cluster{"sample_period":dbl, "sample_rate":dbl, "pulse_length":dbl, "detector":string, "Nchannels":i16, "ADCbits":i16, "BridgeVoltage (V)":sgl, "DAC Range Setting":u8, "AD 7730 Bit Settings":i32, "DAC and AD Settings":i32, "start time":i64, "Pre-start time (ms) of DAQ Typically set to 1000 ms":i32, "Measured Time for DAQ [ms] ":u32, "single channel number":i64, "maximum voltage @ 10MW single channel":dbl, "ExptSampleFrequency (Hz)":sgl, "single channel voltage factor":dbl, "CalibSampleFrequency (Hz)":sgl, "predicted time [ms] to finalize DAQ":dbl, "CalStep1 (V)":string, "CalStep2 (V)":string, "data string":string}[]
  T27 = cluster{"sample_period":dbl, "sample_rate":dbl, "pulse_length":dbl, "detector":string, "Nchannels":i16, "ADCbits":i16, "BridgeVoltage (V)":sgl, "DAC Range Setting":u8, "AD 7730 Bit Settings":i32, "DAC and AD Settings":i32, "chanDescs":cluster{"name":string, "active":i32, "physicalQuantity":cluster{"type":string}}[], "start time":i64, "Pre-start time (ms) of DAQ Typically set to 1000 ms":i32, "Measured Time for DAQ [ms] ":u32, "single channel number":i64, "maximum voltage @ 10MW single channel":dbl, "ExptSampleFrequency (Hz)":sgl, "single channel voltage factor":dbl, "CalibSampleFrequency (Hz)":sgl, "predicted time [ms] to finalize DAQ":dbl, "CalStep1 (V)":string, "CalStep2 (V)":string, "data string":string}
  T28 = cluster{"sample_period":dbl, "sample_rate":dbl, "pulse_length":dbl, "detector":string, "Nchannels":i16, "ADCbits":i16, "BridgeVoltage (V)":sgl, "DAC Range Setting":u8, "AD 7730 Bit Settings":i32, "DAC and AD Settings":i32, "start time":i64, "Pre-start time (ms) of DAQ Typically set to 1000 ms":i32, "Measured Time for DAQ [ms] ":u32, "single channel number":i64, "maximum voltage @ 10MW single channel":dbl, "ExptSampleFrequency (Hz)":sgl, "single channel voltage factor":dbl, "CalibSampleFrequency (Hz)":sgl, "predicted time [ms] to finalize DAQ":dbl, "CalStep1 (V)":string, "CalStep2 (V)":string, "data string":string}
  T29 = cluster{"chanDescs":cluster{"name":string, "active":i32}[]}[]
  T30 = cluster{"rawscal":dbl[], "scale mv":sgl[], "sum scal":dbl[], "tau/dt":dbl[], "F_ch":dbl[], "tau_fact":dbl[], "kbolott_volume":dbl[][], "Vcam":dbl, "scale mv transf":sgl[], "single channel signal factor":dbl, "RTPRad voltage factor":dbl, "SampleTime":sgl, "mean":dbl[], "taum":dbl[], "final channel selection":i64[][], "channel number":i32, "single channel number":i64, "samples to exclude":u32}
  T31 = enum32{"1 to 32", "33 to 64", "65 to 96", "97 to128"}
  T32 = enum32{"1 to 32", "33 to 64", "65 to 96", "97 to 128"}
  T33 = cluster{"Channels 17 - 20":cluster{"tstart":sgl, "dt":sgl, "OutArray":dbl[][]}, "Channels 21 - 24":cluster{"tstart":sgl, "dt":sgl, "OutArray":dbl[][]}, "Channels 25 - 28":cluster{"tstart":sgl, "dt":sgl, "OutArray":dbl[][]}, "Channels 29 - 32":cluster{"tstart":sgl, "dt":sgl, "OutArray":dbl[][]}}
  T34 = cluster{"Channels 1- 4":cluster{"tstart":sgl, "dt":sgl, "OutArray":dbl[][]}, "Channels 5 - 8":cluster{"tstart":sgl, "dt":sgl, "OutArray":dbl[][]}, "Channels 9 - 12":cluster{"tstart":sgl, "dt":sgl, "OutArray":dbl[][]}, "Channels 13 - 16":cluster{"tstart":sgl, "dt":sgl, "OutArray":dbl[][]}}
  T35 = cluster{"Channels 49 - 52":cluster{"tstart":sgl, "dt":sgl, "OutArray":dbl[][]}, "Channels 53 - 56":cluster{"tstart":sgl, "dt":sgl, "OutArray":dbl[][]}, "Channels 57 - 60":cluster{"tstart":sgl, "dt":sgl, "OutArray":dbl[][]}, "Channels 61 - 64":cluster{"tstart":sgl, "dt":sgl, "OutArray":dbl[][]}}
  T36 = cluster{"Channels 33 - 36":cluster{"tstart":sgl, "dt":sgl, "OutArray":dbl[][]}, "Channels 37 - 40":cluster{"tstart":sgl, "dt":sgl, "OutArray":dbl[][]}, "Channels 41 - 44":cluster{"tstart":sgl, "dt":sgl, "OutArray":dbl[][]}, "Channels 45 - 48":cluster{"tstart":sgl, "dt":sgl, "OutArray":dbl[][]}}
  T37 = cluster{"Channels 81 - 84":cluster{"tstart":sgl, "dt":sgl, "OutArray":dbl[][]}, "Channels 85 - 88":cluster{"tstart":sgl, "dt":sgl, "OutArray":dbl[][]}, "Channels 89 - 92":cluster{"tstart":sgl, "dt":sgl, "OutArray":dbl[][]}, "Channels 93 - 96":cluster{"tstart":sgl, "dt":sgl, "OutArray":dbl[][]}}
  T38 = cluster{"Channels 65 - 68":cluster{"tstart":sgl, "dt":sgl, "OutArray":dbl[][]}, "Channels 69 - 72":cluster{"tstart":sgl, "dt":sgl, "OutArray":dbl[][]}, "Channels 73 - 76":cluster{"tstart":sgl, "dt":sgl, "OutArray":dbl[][]}, "Channels 77 - 80":cluster{"tstart":sgl, "dt":sgl, "OutArray":dbl[][]}}
  T39 = cluster{"Channels 113 - 116":cluster{"tstart":sgl, "dt":sgl, "OutArray":dbl[][]}, "Channels 117 - 120":cluster{"tstart":sgl, "dt":sgl, "OutArray":dbl[][]}, "Channels 121 - 124":cluster{"tstart":sgl, "dt":sgl, "OutArray":dbl[][]}, "Channels 125 - 128":cluster{"tstart":sgl, "dt":sgl, "OutArray":dbl[][]}}
  T40 = cluster{"Channels 97 - 100":cluster{"tstart":sgl, "dt":sgl, "OutArray":dbl[][]}, "Channels 101 - 104":cluster{"tstart":sgl, "dt":sgl, "OutArray":dbl[][]}, "Channels 104 - 108":cluster{"tstart":sgl, "dt":sgl, "OutArray":dbl[][]}, "Channels 109 - 112":cluster{"tstart":sgl, "dt":sgl, "OutArray":dbl[][]}}
  T41 = cluster{"tstart":sgl, "dt":sgl, "OutArray":dbl[][]}
  T42 = cluster{"Channels 9 - 12":cluster{"tstart":sgl, "dt":sgl, "OutArray":dbl[][]}, "Channels 9 - 12":cluster{"tstart":sgl, "dt":sgl, "OutArray":dbl[][]}, "Channels 9 - 12":cluster{"tstart":sgl, "dt":sgl, "OutArray":dbl[][]}, "Channels 9 - 12":cluster{"tstart":sgl, "dt":sgl, "OutArray":dbl[][]}}
  T43 = typedef "nirio_resource_hc.ctl" = tag
  T44 = typedef "XDNodeRunTimeDep.lvlib/timing_clust.ctl" = cluster{"Expected End [f-1]":u64, "Actual End [f-1]":u64, "Finished Late? [f-1]":bool, "Expected End [i-1]":u64, "Actual End [i-1]":u64, "Finished Late? [i-1]":bool, "Expected Start [i]":u64, "Actual Start [i]":u64, "Expected Start [f]":u64, "Actual Start [f]":u64, "Source Name":string, "Structure Name":string, "Period":i64, "Deadline":i64, "Offset":i64, "Start":i64, "Priority":i32, "Timeout":i32, "Mode":T45, "Wakeup Reason":T46, "Error":errorcluster, "Source Type":string, "Secondary Source Type":string, "Global End Time":u64, "Global Start Time":u64, "Frame Duration":u64, "Iteration Duration":u64, "Assigned CPU":i32, "I/O Scan Engine Mode":u32}
  T45 = typedef "XDNodeRunTimeDep.lvlib/nitl_modes.ctl" = enum32{"No Change", "Process missed periods, maintain original phase", "Discard missed periods, maintain original phase", "Process missed periods, ignore original phase", "Discard missed periods, ignore original phase"}
  T46 = typedef "XDNodeRunTimeDep.lvlib/wakeup.ctl" = enum32{"Normal", "Aborted", "Asynchronous wakeup", "Timing source error", "Timed loop error", "Timeout"}
  T47 = cluster{"Channels 33 - 40":cluster{"tstart":dbl, "FPGSampleTime":dbl, dbl[][]}, "Channels 41 - 48":cluster{"tstart":dbl, "FPGSampleTime":dbl, dbl[][]}, "Channels 49 - 56":cluster{"tstart":dbl, "FPGSampleTime":dbl, dbl[][]}, "Channels 57 - 58":cluster{"tstart":dbl, "FPGSampleTime":dbl, dbl[][]}}
  T48 = cluster{"Array":dbl[], sgl[], "Array 2":dbl[], "Tau00":dbl[], "F_ch":dbl[], "tau_fact":dbl[], "all rows":dbl[][], dbl, sgl[], "single channel signal factor":dbl, "RTPRad voltage factor":dbl, "SampleTime":sgl, dbl[], "ArrayOutput":dbl[], "all rows":i64[][], i32, "single channel number":i64, "samples to exclude":u32}
  T49 = cluster{"real time P_rad":refnum<vi>, "real time P_rad array":refnum<vi>, "single channel voltage":refnum<vi>, "single channel voltage array":refnum<vi>}
  T50 = cluster{"Channels 1- 8":cluster{"tstart":sgl, "dt":sgl, "OutArray":dbl[][]}, "Channels 9 - 16":cluster{"tstart":sgl, "dt":sgl, "OutArray":dbl[][]}, "Channels 17 - 24":cluster{"tstart":sgl, "dt":sgl, "OutArray":dbl[][]}, "Channels 25 - 32":cluster{"tstart":sgl, "dt":sgl, "OutArray":dbl[][]}}
  T51 = cluster{"Channels 33 - 40":cluster{"tstart":sgl, "dt":sgl, "OutArray":dbl[][]}, "Channels 41 - 48":cluster{"tstart":sgl, "dt":sgl, "OutArray":dbl[][]}, "Channels 49 - 56":cluster{"tstart":sgl, "dt":sgl, "OutArray":dbl[][]}, "Channels 57 - 58":cluster{"tstart":sgl, "dt":sgl, "OutArray":dbl[][]}}
  T52 = typedef "LabVIEWHTTPClient.lvlib/ClientHandle.ctl" = refnum<k1>
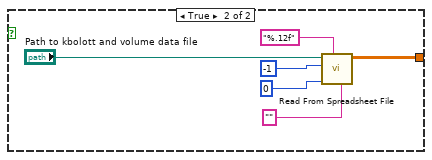
[diagram p2: hidden frame]
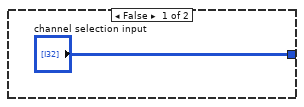
[diagram p4: hidden frame]
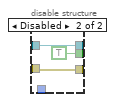
[diagram p6: hidden frame]
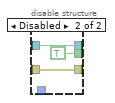
[diagram p7: hidden frame]
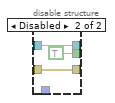
[diagram p8: hidden frame]
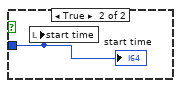
[diagram p9: hidden frame]
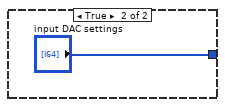
[diagram p12: hidden frame]
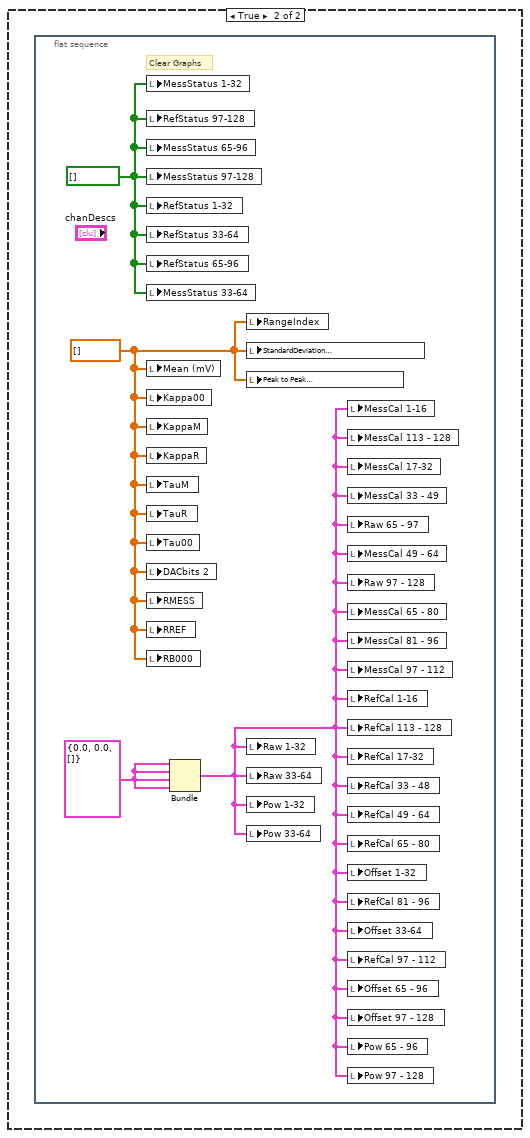
[diagram p14: hidden frame]
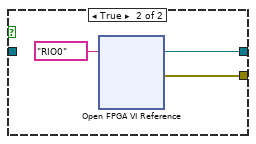
[diagram p15: hidden frame]
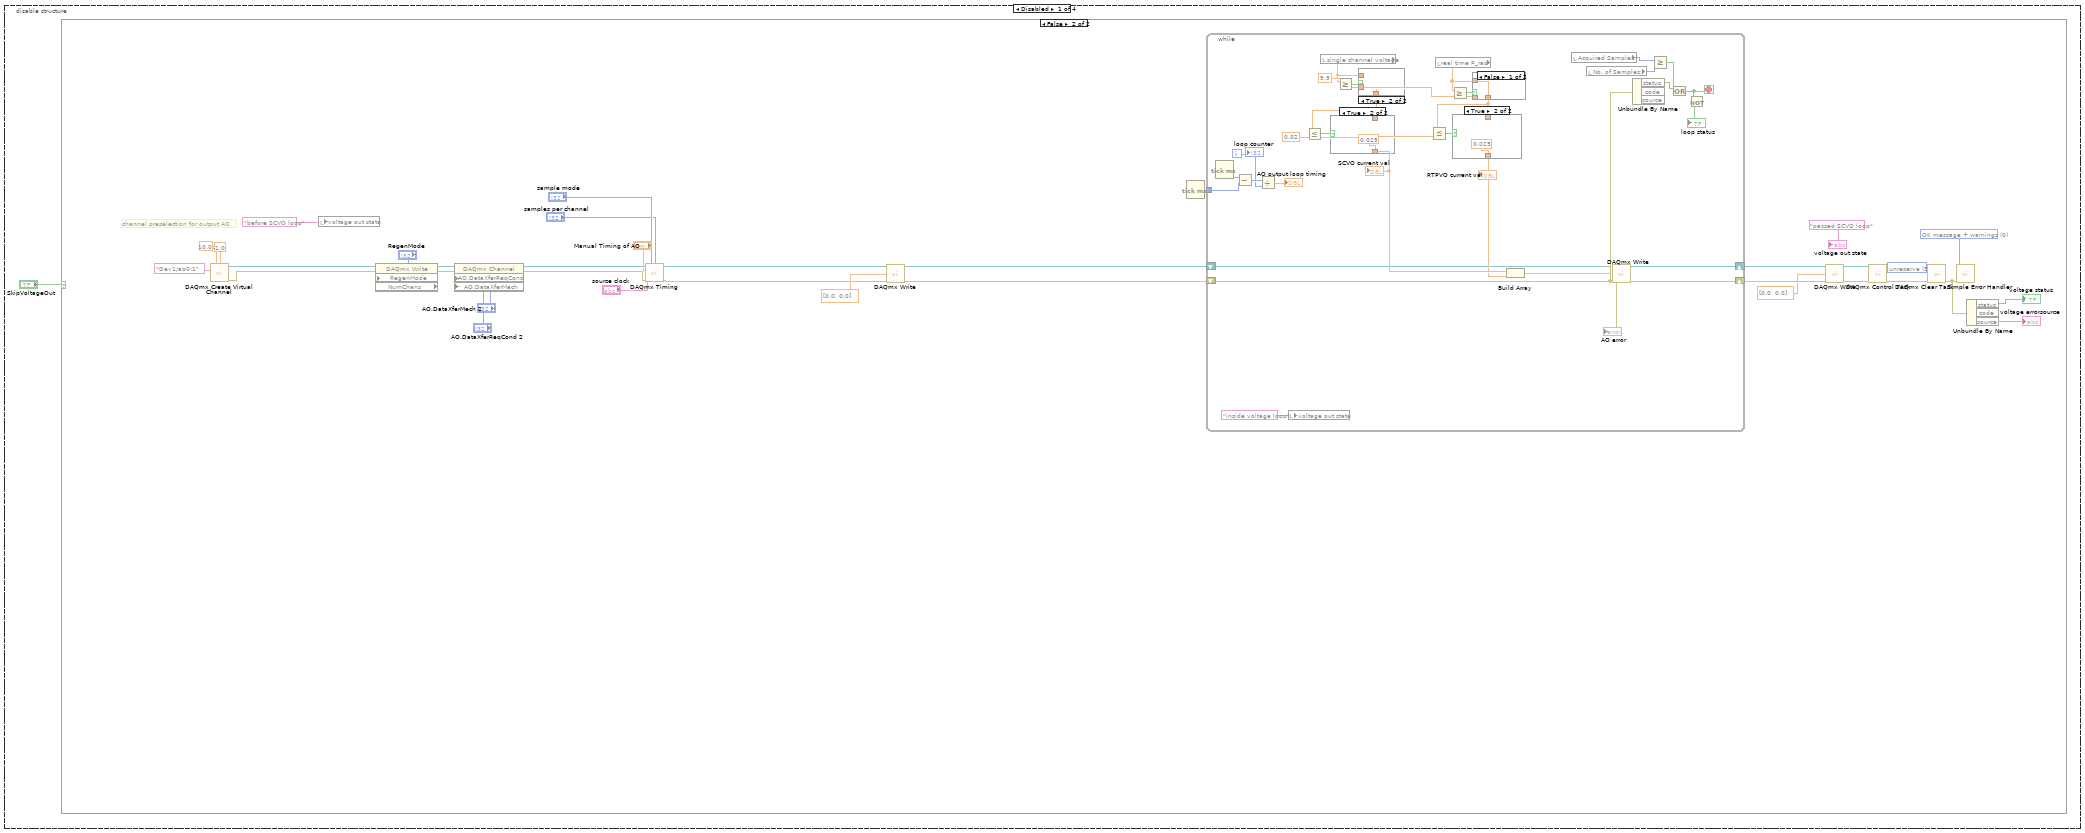
[diagram p17: hidden frame]
diagram:
  w152 = i64 -1000000000  # Ns per Sec
  # "#Timing \n\nAC measurements\n2.5 kHz\nwith SKIP=1 \n\n= 5MHz/16/(3*37+14)"
  # "#Timing \n\nAC measurements\n1.25 kHz\nwith SKIP=0 \n\n= 5MHz/16/250"
  # "#Timing \n\nAC measurements\n2.083 kHz\nwith SKIP=1 \n\n= 5MHz/16/(3*45+15)"
  # "back to synch state"
  # "A (IFS at 80mV) ++ 8 (IZS at input range) ++ C (SZS at input range) ++ 2 (CCM)"
  # "xEXXX (1110)    1 1 1        System Full-Scale Calibration\n====================================================================\nFull-Scale System Calibration Mode. This activates full-scale system calibration on the selected input\nchannel. Calibration is performed at the selected gain on the input voltage provided at the analog input\nduring this calibration sequence. This input voltage should remain stable for the duration of the calibra-\ntion. When this full-scale system calibration is complete, the part updates the contents of the appropriate\nGain Calibration Register and returns to Sync Mode with MD2, MD1 and MD0 returning to 0, 0, 0.\nThe RDY output and bit go high when calibration is initiated and return low when this full-scale calibra-\ntion is complete to indicate that the part is back in Sync Mode and ready for further operations.\n\nCalibration on externally-applied input voltage with PGA set for selected input range. The input applied is assumed\nto be the full-scale of the system. If ac = 1, the system continues to use ac excitation for the duration of the\ncalibration. This calibration should be preceded by a System Zero-Scale or Internal Zero-Scale calibration. The\nGain Calibration Register for the selected channel is updated at the end of this calibration sequence."
  # "xCXXX (1100)    1 1 0        System Zero-Scale Calibration\n=====================================================================\nZero-Scale System Calibration Mode. This activates zero scale system calibration on the channel selected\nby CH1 and CH0 of the Mode Register. Calibration is performed at the selected gain on the input volt-\nage provided at the analog input during this calibration sequence. This input voltage should remain\nstable for the duration of the calibration. When this zero-scale system calibration is complete, the part\nupdates the contents of the appropriate Offset Calibration Register and returns to Sync Mode with MD2,\nMD1 and MD0 returning to 0, 0, 0. The RDY output and bit go high when calibration is initiated and\nreturn low when this zero-scale calibration is complete to indicate that the part is back in Sync Mode and\nready for further operations.\n\nCalibration on externally applied input voltage with PGA set for selected input range. The input applied is assumed\nto be the zero scale of the system. If ac = 1, the system continues to use ac excitation for the duration of the\ncalibration. For full system calibration, this System Zero-Scale calibration should be performed first. For applications\nwhich require a System Zero-Scale and Internal Full-Scale calibration, this calibration should be preceded by the\nInternal Full-Scale calibration. The Offset Calibration Register for the selected channel is updated at the end of\nthis calibration sequence."
  # "xAXXX (1010)    1 0 1        Internal Full-Scale Calibration\n=====================================================================\nFull-Scale Self-Calibration Mode. This activates full-scale self-calibration on the channel selected by\nCH1 and CH0 of the Mode Register. This full-scale self-calibration is performed at the selected gain on\nan internally-generated full-scale signal. When this full-scale self-calibration is complete, the part updates\nthe contents of the appropriate Gain Calibration Register and Offset Calibration Register and returns to\nSync Mode with MD2, MD1 and MD0 returning to 0, 0, 0. The RDY output and bit go high when\ncalibration is initiated and return low when this full-scale self-calibration is complete to indicate that the\npart is back in Sync Mode and ready for further operations\n\nCalibration on internally-generated input full-scale with PGA set for selected input range. The ac bit is ignored for\nthis calibration sequence. The sequence is performed with dc excitation. The Gain Calibration Register for the\nselected channel is updated at the end of this calibration sequence. It is recommended that internal full-scale\ncalibrations are performed on the 80 mV range, regardless of the subsequent operating range, to optimize the post-\ncalibration gain error. This calibration should be followed by either an Internal Zero-Scale or System Zero-Scale\ncalibration. This zero-scale calibration should be performed at the operating input range."
  # "x8XXX (1000)    1 0 0       Internal Zero-Scale Calibration\n========================================================================\nZero-Scale Self-Calibration Mode. This activates zero-scale self-calibration on the channel selected by\nCH1 and CH0 of the Mode Register. This zero-scale self-calibration is performed at the selected gain on\ninternally shorted (zeroed) inputs. When this zero-scale self-calibration is complete, the part updates the\ncontents of the appropriate Offset Calibration Register and returns to Sync Mode with MD2, MD1 and\nMD0 returning to 0, 0, 0. The RDY output and bit go high when calibration is initiated and return low\nwhen this zero-scale self-calibration is complete to indicate that the part is back in Sync Mode and ready\nfor further operations.\n\nCalibration on internal shorted input with PGA set for selected input range. The ac bit is ignored for this calibra-\ntion sequence. The sequence is performed with dc excitation. The Offset Calibration Register for the selected channel is\nupdated at the end of this calibration sequence. For full selfcalibration, this calibration should be preceded by an Internal\nFull-Scale calibration. For applications which require an Internal Zero-Scale and System Full-Scale calibration, this\nInternal Zero-Scale calibration should be performed first."
  # "x6XXX (0110)    0 1 1        Power-Down (Standby) Mode\n============================================================\nPower-Down (Standby) Mode. In this mode, the AD7730 goes into its power-down or standby state.\nPlacing the part in this mode is equivalent to exerting the STANDBY input pin. However, exerting\nSTANDBY does not actually force these mode bits to 0, 1, 1."
  # "x4XXX (0100)    0 1 0        Single Conversion Mode\n===============================================================\nSingle Conversion Mode. In this mode, the AD7730 performs a single conversion, updates the Data\nRegister, returns to the Sync Mode and resets the mode bits to 0, 0, 0. The result of the single conversion\non the AD7730 in this mode will not be provided until the full settling time of the filter has elapsed."
  # "x2XXX (0010)    0 0 1        Continuous Conversion Mode\n==============================================================\nContinuous Conversion Mode. In this mode, the AD7730 is continuously processing data and providing\nconversion results to the Data Register at the programmed output update rate (as determined by the\nFilter Register). For most applications, this would be the normal operating mode of the AD7730"
  # "x0XXX (0000)    0 0 0        Sync (Idle) Mode Power-On/Reset Default\n=============================================================\nSync (Idle) Mode. In this mode, the modulator and filter are held in reset mode and the AD7730 is not\nprocessing any new samples or data. Placing the part in this mode is equivalent to exerting the SYNC\ninput pin. However, exerting the SYNC pin does not actually force these mode bits to 0, 0, 0. The part\nreturns to this mode after a calibration or after a conversion in Single Conversion Mode. This is the\ndefault condition of these bits after Power-On/Reset."
  # "HEX (BIN)          BINARY    STATUS\n=========================================\nx8XXX (1000)    1 0 0        Internal Zero-Scale Calibration\n\nx9XXX (1001)    1 0 0        Internal Zero-Scale Calibration\n\nxAXXX (1010)    1 0 1        Internal Full-Scale Calibration\n\nxBXXX (1011)    1 0 1        Internal Full-Scale Calibration\n\nxCXXX (1100)    1 1 0        System Zero-Scale Calibration\n\nxDXXX (1101)    1 1 0        System Zero-Scale Calibration\n\nxEXXX (1110)    1 1 1       System Full-Scale Calibration\n\nxFXXX (1111)    1 1 1        System Full-Scale Calibration\n\nx0XXX (0000)    0 0 0       Sync (Idle) Mode Power-On/Reset Default\n\nx1XXX (0001)    0 0 0       Sync (Idle) Mode Power-On/Reset Default\n\nx2XXX (0010)    0 0 1       Continuous Conversion Mode\n\nx3XXX (0011)    0 0 1       Continuous Conversion Mode\n\nx4XXX (0100)    0 1 0       Single Conversion Mode\n\nx5XXX (0101)    0 1 0       Single Conversion Mode\n\nx6XXX (0110)    0 1 1       Power-Down (Standby) Mode\n\nx7XXX (0111)    0 1 1       Power-Down (Standby) Mode"
  # "Negative Sample Time [ns]"
  # "Index von dem Sample\nals der Trigger empfangen wurde"
  # "T1 Trigger\nkommt hier"
  # "A=> Internal full scale calibration\n8=> Internal zero scale calibration\nC=> System Zero scale Calibration\n2=> Continuous conversion\n\n5V reference\n80 mV scale\nChannel 1 input (voltage at bridge)\nMaster clock disable\n\np.15 7730 manual"
  # "AC 1.25 kHz Frequenz\nSKIP=0"
  n1 = call <vilib>:"High Resolution Relative Seconds.vi"() -> ("relative seconds"=w157:dbl)
  n2 = flat-sequence {
    tunnel: [w220] -> w158
    tunnel: ["FPGA VI\nReference In"] -> w180
    tunnel: [w221] -> w178
    tunnel: w158 -> [w221]
    frame #0 {
      n3 = Tick Count (ms)() -> (millisecond timer value=w220:u32)
    }
    frame #1 {
      n4 = case shown="False" "Clear all Values \nfrom Beginning" {
        frame False {
        }
        frame True {
          n5 = flat-sequence {
            frame #0 {
              w225 = bool[] [] ("MessStatus 1-32")
              w224 = dbl[] [] ("Kappa00")
              w227 = T41 {"tstart"=0.0, "dt"=0.0, "OutArray"=[]} ("Channels 9 - 12")
              # "Clear Graphs"
              n6 = local write "MessStatus 1-32"(w225) -> ()
              n7 = local write "RefStatus 97-128"(w225) -> ()
              n8 = local write "MessStatus 65-96"(w225) -> ()
              n9 = local write "MessStatus 97-128"(w225) -> ()
              n10 = local write "RefStatus 1-32"(w225) -> ()
              n11 = local write "RefStatus 33-64"(w225) -> ()
              n12 = local write "RefStatus 65-96"(w225) -> ()
              n13 = local write "MessStatus 33-64"(w225) -> ()
              n14 = local write "Mean (mV)"(w224) -> ()
              n15 = local write "Kappa00"(w224) -> ()
              n16 = local write "KappaM"(w224) -> ()
              n17 = local write "KappaR"(w224) -> ()
              n18 = local write "TauM"(w224) -> ()
              n19 = local write "TauR"(w224) -> ()
              n20 = local write "Tau00"(w224) -> ()
              n21 = local write "DACbits 2"(w224) -> ()
              n22 = local write "RMESS"(w224) -> ()
              n23 = local write "RREF"(w224) -> ()
              n24 = local write "RB000"(w224) -> ()
              n25 = Bundle("Channels 9 - 12"=w227, "Channels 9 - 12"=w227, "Channels 9 - 12"=w227, "Channels 9 - 12"=w227) -> (w226:T42)  [unwired: 1 in]
              n26 = local write "RangeIndex"(w224) -> ()
              n27 = local write "StandardDeviation\n        (microV)"(w224) -> ()
              n28 = local write "Peak to Peak \n      (microV)"(w224) -> ()
              n29 = local write "Raw 1-32"(w226) -> ()
              n30 = local write "Raw 33-64"(w226) -> ()
              n31 = local write "Pow 1-32"(w226) -> ()
              n32 = local write "Pow 33-64"(w226) -> ()
              n33 = local write "MessCal 1-16"(w226) -> ()
              n34 = local write "MessCal 113 - 128"(w226) -> ()
              n35 = local write "MessCal 17-32"(w226) -> ()
              n36 = local write "MessCal 33 - 49"(w226) -> ()
              n37 = local write "Raw 65 - 97"(w226) -> ()
              n38 = local write "MessCal 49 - 64"(w226) -> ()
              n39 = local write "Raw 97 - 128"(w226) -> ()
              n40 = local write "MessCal 65 - 80"(w226) -> ()
              n41 = local write "MessCal 81 - 96"(w226) -> ()
              n42 = local write "MessCal 97 - 112"(w226) -> ()
              n43 = local write "RefCal 1-16"(w226) -> ()
              n44 = local write "RefCal 113 - 128"(w226) -> ()
              n45 = local write "RefCal 17-32"(w226) -> ()
              n46 = local write "RefCal 33 - 48"(w226) -> ()
              n47 = local write "RefCal 49 - 64"(w226) -> ()
              n48 = local write "RefCal 65 - 80"(w226) -> ()
              n49 = local write "Offset 1-32"(w226) -> ()
              n50 = local write "RefCal 81 - 96"(w226) -> ()
              n51 = local write "Offset 33-64"(w226) -> ()
              n52 = local write "RefCal 97 - 112"(w226) -> ()
              n53 = local write "Offset 65 - 96"(w226) -> ()
              n54 = local write "Offset 97 - 128"(w226) -> ()
              n55 = local write "Pow 65 - 96"(w226) -> ()
              n56 = local write "Pow 97 - 128"(w226) -> ()
            }
          }
        }
      }
    }
  }
  n57 = disable-structure shown="Enabled" {
    disable-tunnel: w157 -> [w228 _]
    frame Enabled {
      n58 = while {
        tunnel: w228 -> [w236]
        i -> [w246]
        stop <- w247 stop-if-true
        n59 = local read "Fixed T-60sec before T1 = T0"() -> (w232:i32)
        n60 = local read "Pre-start time (ms) of\nDAQ Typically set to 1000 ms"() -> (w242:i32)
        n61 = Divide(x=w232, y=1000) -> (x/y=w230:dbl)
        n62 = Divide(x=w242, y=1000) -> (x/y=w239:dbl)
        n63 = To Quad Integer(1:w239) -> (0:w240:i64)
        n64 = To Quad Integer(1:w230) -> (0:w229:i64)
        n65 = Subtract(x=w229, y=w240) -> (x-y=w237:i64)
        n66 = call <vilib>:"High Resolution Relative Seconds.vi"() -> ("relative seconds"=w234:dbl)
        n67 = To Double Precision Float(number=w237) -> (double precision float=w238:dbl)
        n68 = Add(x=w236, y=w238) -> (x+y=w235:dbl)
        n69 = Subtract(x=w235, y=w234) -> (x-y=→"Time until Acqusition":dbl)
        n70 = Get Date/Time In Seconds() -> (seconds since 1Jan1904=w253:timestamp)
        "current epoch time timestamp" <- w253
        n71 = To Quad Integer(1:w253) -> (0:w255:i64)
        n72 = Subtract(x=w255, y=2082844800) -> (x-y=w251:i64)
        n73 = Multiply(x=1000000000, y=w251) -> (x*y=w243:i64)
        "Number of nanoseconds with offset to 1904" <- w243
        n74 = Wait Until Next ms Multiple(millisecond multiple=1) -> ()  [unwired: 1 out]
        n75 = local read "state"() -> (w248:string)
        n76 = Equal?(x="Acquiring Data...", y=w248) -> (x = y?=w247:bool)
        n77 = Equal?(x=w246, y=0) -> (x = y?=w244:bool)
        n78 = case shown="False" w244 {
          tunnel: w243 -> [_ w256]
          frame False {
          }
          frame True {
            n79 = local write "start time"(w256) -> ()
            "start time" <- w256
          }
        }
      }
    }
    frame Disabled {
    }
  }
  n80 = disable-structure shown="Enabled" {
    frame Enabled {
      n81 = Not(x="?") -> (.not. x?=w260:bool)
      "Take Input for DAC?" <- w260
      n82 = case shown="False" w260 {
        tunnel: "DAC settings file location" -> [w268 _]
        tunnel: [w262 "input DAC settings"] -> w257
        frame False {
          n83 = call-poly <vilib>:"Read From Spreadsheet File.vi"("format (%d)"="%d", "max characters/row  (no limit:0)"=58, "number of rows (all:-1)"=-1, "file path (dialog if empty)"=w268) -> ("all rows"=w263:i64[][])  [unwired: 3 in, 4 out]
          "full DAC\nfile input" <- w263
          n84 = Reshape Array(w263, 128 ("dimension size")) -> (w262:i64[])
        }
        frame True {
        }
      }
      "DAC settings" <- w257
      n85 = local write "input DAC settings"(w257) -> ()
      n86 = Array Size(array=w257) -> (size(s)=→"size(s)":i32)
      "Take file for DAC?" <- "?"
    }
    frame Disabled {
    }
  }
  n87 = disable-structure shown="Enabled" {
    disable-tunnel: [w271 _] -> w57
    disable-tunnel: [w270 _] -> w56
    frame Enabled {
      n88 = Not(x="Read Channel Selection from file") -> (.not. x?=→"Channel Selection\nfrom input?":bool)
      n89 = case shown="True" "Read Channel Selection from file" {
        tunnel: ["channel selection input" w277] -> w271
        frame False {
        }
        frame True {
          n90 = call-poly <vilib>:"Read From Spreadsheet File.vi"("delimiter (\\t)"="\t" ("delimiter (\\t)"), "format (%d)"="%d", "max characters/row  (no limit:0)"=0, "start of read offset (chars.:0)"=0, "number of rows (all:-1)"=-1, "file path (dialog if empty)"="Path to channel selection file") -> ("all rows"=w277:i64[][])  [unwired: 1 in, 4 out]
          "file import" <- w277
        }
      }
      "final channel selection" <- w271
      n91 = Array Size(array=w271) -> (size(s)=w273:i32[])
      n92 = local write "final channel selection"(w271) -> ()
      n93 = Index Array(array=w273, index=0) -> (element=w270:i32)
      "final channel\nselection size" <- w270
    }
    frame Disabled {
    }
  }
  n94 = Not A Number/Path/Refnum?(number/path/refnum=w180) -> (NaN/Path/Refnum?=w179:bool)
  n95 = disable-structure shown="Enabled" {
    disable-tunnel: [w284 _] -> w55
    frame Enabled {
      n96 = case shown="False" "Read geometry from file?" {
        tunnel: [w286 w291] -> w284
        frame False {
          n97 = call "load_kbolott_volume.vi"("HBCmPath"="HBCmPath", "SavePath"="SavePath", "VBClPath"="VBClPath", "VBCrPath"="VBCrPath") -> ("output"=w286:dbl[][])  [unwired: 1 in]
        }
        frame True {
          n98 = call-poly <vilib>:"Read From Spreadsheet File.vi"("delimiter (\\t)"="" ("delimiter (\\t)"), "format (%.3f)"="%.12f", "max characters/row  (no limit:0)"=0, "number of rows (all:-1)"=-1, "file path (dialog if empty)"="Path to kbolott and volume data file") -> ("all rows"=w291:dbl[][])  [unwired: 2 in, 4 out]
        }
      }
      "kbolott_and_volume" <- w284
      n99 = local write "kbolott_and_volume"(w284) -> ()
    }
    frame Disabled {
    }
  }
  n100 = case shown="False" w179 {
    tunnel: [w297 w299] -> w183
    tunnel: [_ w298] -> w182
    tunnel: w180 -> [w297 _]
    frame False {
    }
    frame True {
      n101 = xnode "Open FPGA VI Reference"("resource name"=T43 "RIO0") -> ("FPGA VI Reference Out"=w299:refnum<k20>, "error out"=w298:errorcluster)  [unwired: 1 in]
    }
  }
  "error out" <- w182
  n102 = flat-sequence {
    tunnel: "Cancel" ("name (unnamed)") -> [w310]
    tunnel: "Transferred1" ("name (unnamed)") -> [w309]
    tunnel: u32 0 -> [w308]
    tunnel: FALSE -> [w307]
    tunnel: [w306] -> w210
    tunnel: [w305] -> w209
    tunnel: [w304] -> w208
    tunnel: [w303] -> w207
    tunnel: [u32 0] -> w181
    frame #0 {
      n103 = local write "stop"(FALSE ("stop")) -> ()
      n104 = RT FIFO Create(0:w309, 1:w308) -> (8:w303:refnum<k33>, 11:w304:errorcluster)  [unwired: 2 in, 5 out]
      n105 = RT FIFO Create(0:w310, 1:w307) -> (8:w306:refnum<k33>, 11:w305:errorcluster)  [unwired: 3 in, 4 out]
    }
  }
  n106 = xnode "Read/Write Control"("FPGA VI Reference In"=w183, "error in"=w182, "cancel"=TRUE ("clrFifo"), "Test"=FALSE) -> ("FPGA VI Reference Out"=w219:refnum<k20>, "error out"=w218:errorcluster)
  n107 = flat-sequence {
    tunnel: w219 -> [w317]
    tunnel: w218 -> [w316]
    tunnel: [w315] -> w217
    tunnel: [w314] -> w216
    frame #0 {
      n108 = xnode "Invoke Method"("FPGA VI Reference In"=w317, "error in"=w316, "IRQ Number(s)"=i32[] [0, 1, 2, 3]) -> ("FPGA VI Reference Out"=w315:refnum<k20>, "error out"=w314:errorcluster)
      n109 = Wait (ms)(milliseconds to wait=u32 100) -> ()  [unwired: 1 out]
      "state" <- "Start (100 ms)" ("state")
    }
  }
  n110 = node-c288() -> (w202:T44)  [unwired: 1 in, 4 out]
  n111 = timed-loop {
    tunnel: w210 -> [w328]
    tunnel: w209 -> [w327]
    tunnel: w208 -> [w326]
    tunnel: w207 -> [w325]
    shift-right: [w324] -> _
    shift-left: w181 -> [w318]
    tunnel: [w323] -> w204
    tunnel: [w322] -> w203
    tunnel: [w321] -> w206
    tunnel: [w320] -> w205
    timing: w202 -> [_]
    timing-out: [_] -> w201
    stop <- "stop" stop-if-true
    n112 = RT FIFO Read(0:w325, 1:w318, 3:w326) -> (8:w321:refnum<k33>, 9:w324:u32, 11:w320:errorcluster)  [unwired: 3 out]
    n113 = RT FIFO Write(0:w328, 1:"Cancel Button", 3:w327) -> (8:w323:refnum<k33>, 11:w322:errorcluster)  [unwired: 1 in, 3 out]
    "Acquired Samples:" <- w318
  }
  n114 = flat-sequence {
    tunnel: w216 -> [w333]
    tunnel: [w332] -> w198
    tunnel: w217 -> [w334]
    tunnel: [w335] -> w185
    frame #0 {
      n115 = local write "state"("Reset" ("state")) -> ()
      n116 = call "hReset2014.vi"("error in"=w333, "FPGA VI Reference In"=w334) -> ("error out"=w332:errorcluster, "FPGA VI Reference Out"=w335:refnum<k20>)  [unwired: 4 in]
    }
  }
  n117 = node-c288(w201) -> ()  [unwired: 1 out]
  n118 = call "hFilterReg2014.vi"("error in"=w198, "Filter Modus"=u16 61 ("t"), "Frequenz"=u8 79 ("AC 1kHz Frequenz\nSKIP=0"), "FPGA VI Reference In"=w185) -> ("error out"=w188:errorcluster, "Timed Out"=w194:bool, "FPGA VI Reference Out"=w187:refnum<k20>)  [unwired: 1 in]
  "FilterTimeOut" <- w194
  n119 = flat-sequence {
    tunnel: w206 -> [w341]
    tunnel: w205 -> [w340]
    tunnel: w204 -> [w339]
    tunnel: w203 -> [w338]
    frame #0 {
      n120 = RT FIFO Delete(0:w341, 3:w340) -> ()  [unwired: 1 in, 1 out]
      n121 = RT FIFO Delete(0:w339, 3:w338) -> ()  [unwired: 1 in, 1 out]
      n122 = local write "stop"(FALSE ("stop")) -> ()
    }
  }
  n123 = disable-structure shown="Enabled" {
    disable-tunnel: [w347 TRUE ("Timeout")] -> w196
    disable-tunnel: [w346 w350] -> w192
    disable-tunnel: [w345 w348] -> w190
    disable-tunnel: w188 -> [w344 w348]
    disable-tunnel: w187 -> [w343 w350]
    disable-tunnel: u16 41144 -> [w342 _]
    frame Enabled {
      n124 = call "hModeReg2014.vi"("error in"=w344, "Mode"=w342, "FPGA VI Reference In"=w343) -> ("error out"=w345:errorcluster, "Timeout"=w347:bool, "FPGA VI Reference Out"=w346:refnum<k20>)  [unwired: 2 in]
    }
    frame Disabled {
    }
  }
  n125 = disable-structure shown="Enabled" {
    disable-tunnel: [w356 TRUE ("Timeout")] -> w197
    disable-tunnel: w192 -> [w355 w359]
    disable-tunnel: [w354 w359] -> w191
    disable-tunnel: w190 -> [w353 w357]
    disable-tunnel: [w352 w357] -> w189
    disable-tunnel: u16 32952 -> [w351 _]
    frame Enabled {
      n126 = call "hModeReg2014.vi"("error in"=w353, "Mode"=w351, "FPGA VI Reference In"=w355) -> ("error out"=w352:errorcluster, "Timeout"=w356:bool, "FPGA VI Reference Out"=w354:refnum<k20>)  [unwired: 2 in]
    }
    frame Disabled {
    }
  }
  n127 = disable-structure shown="Enabled" {
    disable-tunnel: [w365 TRUE ("Timeout")] -> w195
    disable-tunnel: w191 -> [w364 w368]
    disable-tunnel: w189 -> [w363 w366]
    disable-tunnel: [w362 w368] -> w161
    disable-tunnel: [w361 w366] -> w160
    disable-tunnel: u16 8376 -> [w360 _]
    frame Enabled {
      n128 = call "hModeReg2014.vi"("error in"=w363, "Mode"=w360, "FPGA VI Reference In"=w364) -> ("error out"=w361:errorcluster, "Timeout"=w365:bool, "FPGA VI Reference Out"=w362:refnum<k20>)  [unwired: 2 in]
    }
    frame Disabled {
    }
  }
  n129 = disable-structure shown="Disabled" {
    disable-tunnel: w161 -> [w372 w374]
    disable-tunnel: w160 -> [w371 w373]
    disable-tunnel: [w370 w373] -> w159
    disable-tunnel: [w369 w374] -> w162
    frame Disabled {
      n130 = call "hModeReg2014.vi"("error in"=w371, "FPGA VI Reference In"=w372) -> ("error out"=w370:errorcluster, "FPGA VI Reference Out"=w369:refnum<k20>)  [unwired: 3 in, 1 out]
    }
    frame Enabled {
    }
  }
  n131 = Compound Arithmetic op=OR(w196, w197, w195, w194) -> (w186:bool)
  "result" <- w186
  n132 = case shown="False" w186 {
    tunnel: [w544 w1659] -> w176
    tunnel: [w543 w1658] -> w215
    tunnel: w162 -> [w682 w1659]
    tunnel: w159 -> [w681 w1658]
    tunnel: [w559 _] -> w119
    tunnel: [w484 _] -> w67
    tunnel: [w585 _] -> w122
    tunnel: [w581 _] -> w90
    tunnel: [w525 _] -> w94
    tunnel: [w390 _] -> w150
    tunnel: [w522 _] -> w147
    tunnel: [w578 _] -> w146
    tunnel: [w577 _] -> w148
    tunnel: [w576 _] -> w145
    tunnel: [w523 _] -> w149
    tunnel: [w486 _] -> w151
    tunnel: w178 -> [w529 _]
    tunnel: [w396 _] -> w153
    tunnel: [w487 _] -> w116
    tunnel: w57 -> [w461 _]
    tunnel: w56 -> [w463 _]
    tunnel: w55 -> [w462 _]
    tunnel: [w391 _] -> w1
    frame False {
      w530 = 5000
      w605 = u8 125  # Frequenz
      w642 = 0.0008 ("FPGSampleTime")
      w637 = 0.0
      w539 = 40.0  # Rcable
      w677 = 10.0  # Rload
      w692 = sgl 0.0004  # dt
      w693 = sgl 0.0  # tstart
      w696 = sgl 0.0004  # dt
      w697 = sgl 0.0  # tstart
      w700 = sgl 80.0 ("Scale(mV)")
      # "pre-allocation of the sample and signal arrays from the subroutine of measurement"
      # "F"
      # "7"
      # "E"
      # "6"
      # "D"
      # "5"
      # "C"
      # "B"
      # "4"
      # "9"
      # "A"
      # "3"
      # "2"
      # "8"
      # "1"
      # "C SZS (input range) ++ E SFS (input range) ++ A IFS (at input range) ++ 8 IZS (input range) ++ 2 CCM"
      # "back to sync state"
      # "offset subtraction on all samples&channels"
      # "A (IFS at 80mV) ++ 8 (IZS at input range) ++ C (SZS at input range) ++ 2 (CCM)"
      # "C (SZS at input range) ++ E (SFS at input range) ++ 8 (IZS at input range) ++ 2 (CCM)"
      # "A (IFS at 80mV) ++ 8 (IZS at input range) ++ C (SZS at input range) ++ 2 (CCM)"
      # "For full selfcalibration, the Internal Zero Scale calibration should be preceded by an Internal\nFull-Scale calibration. For applications which require an Internal Zero-Scale and System Full-Scale calibration, this\nInternal Zero-Scale calibration should be performed first."
      # "System Full-Scale calibration should be preceded by a System Zero-Scale or Internal Zero-Scale calibration. The\nGain Calibration Register for the selected channel is updated at the end of this calibration sequence."
      # "For full system calibration, this System Zero-Scale calibration should be performed first. For applications\nwhich require a System Zero-Scale and Internal Full-Scale calibration, this calibration should be preceded by the\nInternal Full-Scale calibration."
      # "Internal full-scale calibrations are performed on the 80 mV range, and should be followed by either an Internal Zero-Scale or System Zero-Scale\ncalibration. This zero-scale calibration should be performed at the operating input range."
      # "If the interal and system calibration procedures are used in the prior\nDAC range setup, do not subtract the previously measured offset.\n\nThis is ultimately different to the AD7730 acquired offset.\nFrom the manual, concerning the system zero scale calibration:\n\n[...] The input applied is assumed\nto be the zero scale of the system. If ac = 1, the system\ncontinues to use ac excitation for the duration of the\ncalibration. For full system calibration, this System Zero-\nScale calibration should be performed first. For applications\nwhich require a System Zero-Scale and Internal Full-Scale\ncalibration, this calibration should be preceded by the\nInternal Full-Scale calibration. [...]\n\nThough due to the wrong internal wiring, an absolute value\nhas to be taken off the raw signal."
      # "Offset Shift manually disabled because not need for low power discharges"
      # "Local TDMS Data Storage"
      # "Store raw data"
      # "#Offset measurement"
      # "#Range for measurements"
      # "A=> Internal full scale calibration\n8=> Internal zero scale calibration\nC=> System Zero scale Calibration\n2=> Continuous conversion\n\n2.5V reference\n80 mV scale\nChannel 2 input (voltage at shunt)\nMaster clock disable\n\np.15 7730 manual"
      n133 = flat-sequence {
        tunnel: [w1198] -> w542
        tunnel: [w1197] -> w541
        tunnel: w682 -> [w1201]
        tunnel: w681 -> [w1200]
        tunnel: w530 -> [w1206]
        tunnel: [w1205] -> w596
        tunnel: w542 -> [w1208]
        tunnel: w541 -> [w1207]
        tunnel: [w1204] -> w595
        tunnel: [w1214] -> w757
        tunnel: [w1213] -> w756
        tunnel: [w1212] -> w754
        tunnel: w530 -> [w1210]
        tunnel: w596 -> [w1216]
        tunnel: w595 -> [w1215]
        frame #0 {
          n134 = call "hComRegStart2013.vi"("error in"=w1200, "FPGA VI Reference In"=w1201) -> ("error out"=w1197:errorcluster, "Timed Out"=→"Timed Out":bool, "FPGA VI Reference Out"=w1198:refnum<k20>)  [unwired: 3 in]
          n135 = call "Wait3"("Count(mSec)"=u32 3000) -> ()  [unwired: 1 out]
        }
        frame #1 {
          n136 = call "Wait6"("Count(mSec)"=u32 3000) -> ()  [unwired: 1 out]
          n137 = local write "state"("SyncRun (3000 ms)" ("state")) -> ()
          n138 = call "hSync&StartSampling2013.vi"("error in"=w1207, "#Samples"=w1206, "FPGA VI Reference In"=w1208) -> ("error out"=w1205:errorcluster, "FPGA VI Reference Out"=w1204:refnum<k20>)  [unwired: 1 in]
        }
        frame #2 {
          n139 = call "hReadChannelsRTDMA2013.vi"("FPGA VI Reference In"=w1215, "Nsamples"=w1210, "error in"=w1216) -> ("FPGA VI Reference Out"=w1214:refnum<k20>, "Fehler"=→"Fehler":bool, "RawArray"=w1212:i16[][], "error out"=w1213:errorcluster)  [unwired: 2 in]
          n140 = local write "state"("ReadOffset" ("state")) -> ()
        }
      }
      n141 = property on="Acquired Samples:" class="Slide (strict)"("Scale.Range:Maximum"=w530) -> ()  [unwired: 2 in, 2 out]
      n142 = call "hSoftReset2013.vi"("error in"=w756, "FPGA VI Reference In"=w757) -> ("error out"=w603:errorcluster, "FPGA VI Reference Out"=w598:refnum<k20>)  [unwired: 4 in]
      n143 = call "Int2Volt2D.vi"("IntegerArray"=w754, "Scale(mV)"=sgl 80.0) -> ("RealArray"=w537:sgl[][])
      n144 = xnode "Read/Write Control"("FPGA VI Reference In"=w598, "error in"=w603, "HIREF"=TRUE) -> ("FPGA VI Reference Out"=w601:refnum<k20>, "error out"=w600:errorcluster)
      n145 = for {
        tunnel: w537 -> [w1237] mode=indexing
        tunnel: [w1236] -> w632 mode=indexing
        tunnel: [w1235] -> w433 mode=indexing
        tunnel: [w1234] -> w633 mode=indexing
        n146 = Array Subset(array=w1237, index=500, length=1000) -> (w1239:sgl[])
        n147 = Array Max & Min(array=w1239) -> (max value=w1242:sgl, min value=w1243:sgl)  [unwired: 2 out]
        n148 = Subtract(x=w1242, y=w1243) -> (x-y=w1236:sgl)
        n149 = call <vilib>:"Std Deviation and Variance.vi"("X"=w1239, "Weighting (Sample)"=enum16{"Sample", "Population"}."Population") -> ("mean"=w1235:dbl, "standard deviation"=w1234:dbl)  [unwired: 1 out]
      }
      "Offsets" <- w433
      n150 = Array Subset(array=w537, index (row)=0, length (row)=64, index (col)=0) -> (w647:sgl[][])  [unwired: 1 in]
      n151 = Array Subset(array=w537, index (row)=64, length (row)=64, index (col)=0) -> (w643:sgl[][])  [unwired: 1 in]
      n152 = call "Visualize_Signals64.vi"("FPGSampleTime"=w642, "tstart"=w637, "Signals"=w647) -> ("plot(Signals) 33-64"=→"Offset 33-64":T47, "plot(Signals) 1-32"=→"Offset 1-32":T4)  [unwired: 7 in]
      n153 = call "Visualize_Signals64.vi"("FPGSampleTime"=w642, "tstart"=w637, "Signals"=w643) -> ("plot(Signals) 33-64"=→"Offset 97 - 128":T47, "plot(Signals) 1-32"=→"Offset 65 - 96":T4)  [unwired: 7 in]
      n154 = call "hFilterReg2014.vi"("error in"=w600, "Filter Modus"=u16 512 ("t"), "Frequenz"=w605, "FPGA VI Reference In"=w601) -> ("error out"=w599:errorcluster, "FPGA VI Reference Out"=w602:refnum<k20>)  [unwired: 1 in, 1 out]
      n155 = disable-structure shown="Enabled" {
        disable-tunnel: [w1142 w1143] -> w609
        disable-tunnel: [w1141 w1144] -> w608
        disable-tunnel: w602 -> [w1140 w1144]
        disable-tunnel: w599 -> [w1139 w1143]
        disable-tunnel: u16 41017 -> [w1138 _]
        frame Enabled {
          n156 = call "hModeReg2014.vi"("error in"=w1139, "Mode"=w1138, "FPGA VI Reference In"=w1140) -> ("error out"=w1142:errorcluster, "FPGA VI Reference Out"=w1141:refnum<k20>)  [unwired: 2 in, 1 out]
        }
        frame Disabled {
        }
      }
      n157 = disable-structure shown="Enabled" {
        disable-tunnel: w609 -> [w1149 w1150]
        disable-tunnel: w608 -> [w1148 w1151]
        disable-tunnel: [w1147 w1151] -> w607
        disable-tunnel: [w1146 w1150] -> w606
        disable-tunnel: u16 32825 -> [w1145 _]
        frame Enabled {
          n158 = call "hModeReg2014.vi"("error in"=w1149, "Mode"=w1145, "FPGA VI Reference In"=w1148) -> ("error out"=w1146:errorcluster, "FPGA VI Reference Out"=w1147:refnum<k20>)  [unwired: 2 in, 1 out]
        }
        frame Disabled {
        }
      }
      n159 = disable-structure shown="Enabled" {
        disable-tunnel: w607 -> [w1156 w1158]
        disable-tunnel: w606 -> [w1155 w1157]
        disable-tunnel: [w1154 w1158] -> w535
        disable-tunnel: [w1153 w1157] -> w534
        disable-tunnel: u16 8249 -> [w1152 _]
        frame Enabled {
          n160 = call "hModeReg2014.vi"("error in"=w1155, "Mode"=w1152, "FPGA VI Reference In"=w1156) -> ("error out"=w1153:errorcluster, "FPGA VI Reference Out"=w1154:refnum<k20>)  [unwired: 2 in, 1 out]
        }
        frame Disabled {
        }
      }
      n161 = Multiply(x=w633, y=1000000.0 ("Scale")) -> (x*y=→"StandardDeviation\n        (microV)":dbl[])
      n162 = Multiply(x=w632, y=1000000.0 ("Scale")) -> (x*y=→"Peak to Peak \n      (microV)":dbl[])
      n163 = Multiply(x=w433, y=1000.0 ("Scale")) -> (x*y=w486:dbl[])
      "Mean (mV)" <- w486
      n164 = control-ref of="Cancel Button"() -> (w753:refnum<vi>)
      n165 = control-ref of="state"() -> (w752:refnum<vi>)
      n166 = disable-structure shown="Disabled" {
        disable-tunnel: w535 -> [w1163 w1165]
        disable-tunnel: w534 -> [w1162 w1164]
        disable-tunnel: [w1161 w1164] -> w533
        disable-tunnel: [w1160 w1165] -> w532
        disable-tunnel: u16 57 -> [w1159 _]
        frame Disabled {
          n167 = call "hModeReg2014.vi"("error in"=w1162, "Mode"=w1159, "FPGA VI Reference In"=w1163) -> ("error out"=w1161:errorcluster, "FPGA VI Reference Out"=w1160:refnum<k20>)  [unwired: 2 in, 1 out]
        }
        frame Enabled {
        }
      }
      n168 = control-ref of="Acquired Samples:"() -> (w751:refnum<vi>)
      n169 = call "hCalRT2013.vi"("FPGA VI Reference In"=w532, "cancelbutton"=w753, "state"=w752, "Acquired Samples"=w751, "error in"=w533, "Numeric"=10000) -> ("FPGA VI Reference Out"=w679:refnum<k20>, "Ref"=w699:i16[][], "Meas"=w749:i16[][], "error out"=w678:errorcluster)  [unwired: 5 in, 1 out]
      "error out Cal" <- w678
      n170 = case shown="True" "SecondFilter" {
        tunnel: [w1178 w1187] -> w396
        tunnel: [w1177 w1185] -> w594
        tunnel: [w1176 w1186] -> w593
        frame False {
          n171 = disable-structure shown="Enabled" {
            disable-tunnel: [u16 574 ("t") u16 575 ("t")] -> w1176
            disable-tunnel: [u16 37 ("frequenz") u16 45 ("frequenz")] -> w1177
            disable-tunnel: [sgl 0.0004 sgl 0.00048] -> w1178
            frame Enabled {
            }
            frame Disabled {
            }
          }
        }
        frame True {
          n172 = call "FreqSel.vi"("Ring"="FreqSelRing") -> ("Frequency"=w1185:u16, "DLY"=w1186:u16, "SampleTime"=w1187:sgl)  [unwired: 1 out]
        }
      }
      "SampleTime" <- w396
      n173 = call "Int2Volt2D.vi"("IntegerArray"=w699, "Scale(mV)"=w700) -> ("RealArray"=w701:sgl[][])
      n174 = call "Int2Volt2D.vi"("IntegerArray"=w749, "Scale(mV)"=w700) -> ("RealArray"=w750:sgl[][])
      n175 = flat-sequence {
        tunnel: w679 -> [w1227]
        tunnel: w678 -> [w1225]
        tunnel: [w1226] -> w611
        tunnel: [w1224] -> w610
        tunnel: [w1231] -> w574
        tunnel: [w1230] -> w636
        tunnel: w611 -> [w1233]
        tunnel: w610 -> [w1232]
        frame #0 {
          w1221 = FALSE ("RESET")
          n176 = call "Wait"("Count(mSec)"=u16 3000 ("Count(uSec)")) -> ()  [unwired: 1 out]
          n177 = xnode "Read/Write Control"("FPGA VI Reference In"=w1227, "error in"=w1225, "RLY1"=w1221, "RLY2"=w1221, "HIREF"=w1221, "Sprung0"=w1221, "Sprung1"=w1221, "ScanID"=u32 0, "Test"=FALSE, "RESET"=TRUE) -> ("FPGA VI Reference Out"=w1226:refnum<k20>, "error out"=w1224:errorcluster)
          n178 = local write "state"("SoftReset (3000 ms)" ("state")) -> ()
        }
        frame #1 {
          n179 = call "Wait5"("Count(mSec)"=u16 1000 ("Count(uSec)")) -> ()  [unwired: 1 out]
          n180 = xnode "Read/Write Control"("FPGA VI Reference In"=w1233, "error in"=w1232, "RESET"=FALSE) -> ("FPGA VI Reference Out"=w1230:refnum<k20>, "error out"=w1231:errorcluster)
        }
      }
      n181 = case shown="True" "Auto ECRH Time\nor manual control" {
        tunnel: [w768 w782] -> w411
        tunnel: "manual & default\nDAQ time" -> [w768 w769]
        frame False {
        }
        frame True {
          n182 = call "get_ecrh_duration.vi"("default"=w769) -> ("ecrh duration"=w779:dbl, "time needed to find ECRH duration"=→"time needed to\nfind ECRH duration":i64, "date/time string"=→"date/time string":string, "progId"=→"progId":dbl, "last trigger time by codac"=→"CODAC trigger time":i64, "Sucessfull HTTP return?"=→"Sucessfull HTTP return?":bool)  [unwired: 3 in, 2 out]
          "ECRH duration" <- w779
          n183 = To Double Precision Float(number="Pre-start time (ms) of\nDAQ Typically set to 1000 ms") -> (double precision float=w777:dbl)
          n184 = Divide(x=w777, y=1000.0) -> (x/y=w775:dbl)
          n185 = Add(x=w775, y=w779) -> (x+y=w780:dbl)
          n186 = Add(x="AddOn time", y=w780) -> (x+y=w782:dbl)
        }
      }
      "Time of Acqusition [s]" <- w411
      n187 = xnode "Invoke Method"("FPGA VI Reference In"=w636, "error in"=w574, "Requested Depth"=u32 256) -> ("FPGA VI Reference Out"=w575:refnum<k20>, "error out"=w573:errorcluster, "Actual Depth"=→"Actual Depth":u32)
      n188 = local read "input DAC settings"() -> (w538:i64[])
      n189 = call "hFilterReg2014.vi"("error in"=w573, "Filter Modus"=w593, "Frequenz"=w594, "FPGA VI Reference In"=w575) -> ("error out"=w691:errorcluster, "FPGA VI Reference Out"=w690:refnum<k20>)  [unwired: 1 in, 1 out]
      n190 = To Unsigned Byte Integer(number=w538) -> (unsigned 8bit integer=w536:u8[])
      "RangeIndex" <- w536
      n191 = Divide(x=w411, y=w396) -> (x/y=w494:dbl)
      n192 = Round To Nearest(number=w494) -> (nearest integer value=w495:dbl)
      n193 = To Unsigned Long Integer(number=w495) -> (unsigned 32bit integer=w492:u32)
      n194 = Add(x=w492, y="samples to exclude") -> (x+y=w491:u32)
      "No. of Samples:" <- w491
      n195 = case shown="1, Default" "AD 7730 Bit Settings" {
        tunnel: [u16 32904 u16 32952] -> w517
        tunnel: [u16 4232 u16 4280] -> w503
        tunnel: [u16 37000 u16 37048] -> w515
        tunnel: [u16 8328 u16 8376] -> w516
        tunnel: [u16 12424 u16 12472] -> w514
        tunnel: [u16 41096 u16 41144] -> w513
        tunnel: [u16 16520 u16 16568] -> w512
        tunnel: [u16 45192 u16 45240] -> w511
        tunnel: [u16 20616 u16 20664] -> w509
        tunnel: [u16 49288 u16 49336] -> w510
        tunnel: [u16 24712 u16 24760] -> w507
        tunnel: [u16 53384 u16 53432] -> w508
        tunnel: [u16 57480 u16 57528] -> w506
        tunnel: [u16 28808 u16 28856] -> w505
        tunnel: [u16 61576 u16 61624] -> w504
        frame 0 {
        }
        frame 1, Default {
        }
      }
      n196 = case shown="3, Default" "DAC and AD Settings" {
        tunnel: w691 -> [w1462 w1516 w1577 w1621]
        tunnel: w690 -> [w1463 w1517 w1576 w1620]
        tunnel: [w1470 w1524 w1575 w1619] -> w634
        tunnel: [w1474 w1528 w1568 w1612] -> w635
        tunnel: w536 -> [w1461 w1515 _ _]
        tunnel: w503 -> [_ _ _ _]
        tunnel: w517 -> [w1458 _ w1566 _]
        tunnel: w516 -> [w1459 w1513 w1567 w1611]
        tunnel: w515 -> [_ _ _ _]
        tunnel: w514 -> [_ _ _ _]
        tunnel: w513 -> [w1457 _ w1565 _]
        tunnel: w512 -> [_ _ _ _]
        tunnel: w511 -> [_ _ _ _]
        tunnel: w510 -> [_ w1512 _ w1610]
        tunnel: w509 -> [_ _ _ _]
        tunnel: w508 -> [_ _ _ _]
        tunnel: w507 -> [_ _ _ _]
        tunnel: w506 -> [_ _ _ _]
        tunnel: w505 -> [_ _ _ _]
        tunnel: w504 -> [_ _ _ _]
        tunnel: "Global DAC Range Setting" -> [_ _ w1564 w1609]
        frame 3, Default {
          n197 = Initialize Array(u8 3 ("element"), 128 ("dimension size")) -> (w1460:u8[])
          n198 = disable-structure shown="Enabled" {
            disable-tunnel: w1463 -> [w1479 w1481]
            disable-tunnel: w1462 -> [w1478 w1480]
            disable-tunnel: [w1477 w1481] -> w1465
            disable-tunnel: [w1476 w1480] -> w1464
            disable-tunnel: w1461 -> [_ _]
            disable-tunnel: w1460 -> [_ _]
            frame Disabled {
              n199 = call "hModeRegRange2013.vi"("error in"=w1478, "FPGA VI Reference In"=w1479) -> ("error out"=w1476:errorcluster, "FPGA VI Reference Out"=w1477:refnum<k20>)  [unwired: 3 in, 1 out]
            }
            frame Enabled {
            }
          }
          n200 = disable-structure shown="Enabled" {
            disable-tunnel: w1465 -> [w1485 w1487]
            disable-tunnel: w1464 -> [w1484 w1486]
            disable-tunnel: [w1483 w1487] -> w1475
            disable-tunnel: [w1482 w1486] -> w1473
            disable-tunnel: w1461 -> [_ _]
            disable-tunnel: w1460 -> [_ _]
            frame Disabled {
              n201 = call "hModeRegRange2013.vi"("error in"=w1484, "FPGA VI Reference In"=w1485) -> ("error out"=w1482:errorcluster, "FPGA VI Reference Out"=w1483:refnum<k20>)  [unwired: 3 in, 1 out]
            }
            frame Enabled {
            }
          }
          n202 = disable-structure shown="Disabled" {
            disable-tunnel: w1475 -> [w1493 w1495]
            disable-tunnel: w1473 -> [w1492 w1494]
            disable-tunnel: [w1491 w1495] -> w1472
            disable-tunnel: [w1490 w1494] -> w1468
            disable-tunnel: w1460 -> [w1488 _]
            disable-tunnel: w1457 -> [w1489 _]
            frame Enabled {
              n203 = call "hModeRegRange2013.vi"("error in"=w1492, "RangeArray"=w1488, "Mode"=w1489, "FPGA VI Reference In"=w1493) -> ("error out"=w1490:errorcluster, "FPGA VI Reference Out"=w1491:refnum<k20>)  [unwired: 1 in, 1 out]
            }
            frame Disabled {
            }
          }
          n204 = disable-structure shown="Enabled" {
            disable-tunnel: w1472 -> [w1509 w1511]
            disable-tunnel: w1468 -> [w1508 w1510]
            disable-tunnel: [w1507 w1510] -> w1471
            disable-tunnel: [w1506 w1511] -> w1469
            disable-tunnel: w1461 -> [w1505 _]
            disable-tunnel: w1460 -> [_ _]
            disable-tunnel: w1458 -> [w1504 _]
            frame Enabled {
              n205 = call "hModeRegRange2013.vi"("error in"=w1508, "RangeArray"=w1505, "Mode"=w1504, "FPGA VI Reference In"=w1509) -> ("error out"=w1507:errorcluster, "FPGA VI Reference Out"=w1506:refnum<k20>)  [unwired: 1 in, 1 out]
            }
            frame Disabled {
            }
          }
          n206 = disable-structure shown="Enabled" {
            disable-tunnel: [w1500 w1503] -> w1470
            disable-tunnel: w1471 -> [w1499 w1503]
            disable-tunnel: w1469 -> [w1498 w1502]
            disable-tunnel: [w1501 w1502] -> w1474
            disable-tunnel: w1461 -> [w1497 _]
            disable-tunnel: w1460 -> [_ _]
            disable-tunnel: w1459 -> [w1496 _]
            frame Enabled {
              n207 = call "hModeRegRange2013.vi"("error in"=w1499, "RangeArray"=w1497, "Mode"=w1496, "FPGA VI Reference In"=w1498) -> ("error out"=w1500:errorcluster, "FPGA VI Reference Out"=w1501:refnum<k20>)  [unwired: 1 in, 1 out]
            }
            frame Disabled {
            }
          }
        }
        frame 2 {
          n208 = Initialize Array(u8 3 ("element"), 128 ("dimension size")) -> (w1514:u8[])
          n209 = disable-structure shown="Enabled" {
            disable-tunnel: w1517 -> [w1533 w1535]
            disable-tunnel: w1516 -> [w1532 w1534]
            disable-tunnel: [w1531 w1535] -> w1519
            disable-tunnel: [w1530 w1534] -> w1518
            disable-tunnel: w1515 -> [_ _]
            disable-tunnel: w1514 -> [_ _]
            frame Disabled {
              n210 = call "hModeRegRange2013.vi"("error in"=w1532, "FPGA VI Reference In"=w1533) -> ("error out"=w1530:errorcluster, "FPGA VI Reference Out"=w1531:refnum<k20>)  [unwired: 3 in, 1 out]
            }
            frame Enabled {
            }
          }
          n211 = disable-structure shown="Enabled" {
            disable-tunnel: w1519 -> [w1539 w1541]
            disable-tunnel: w1518 -> [w1538 w1540]
            disable-tunnel: [w1537 w1541] -> w1529
            disable-tunnel: [w1536 w1540] -> w1527
            disable-tunnel: w1515 -> [_ _]
            disable-tunnel: w1514 -> [_ _]
            frame Disabled {
              n212 = call "hModeRegRange2013.vi"("error in"=w1538, "FPGA VI Reference In"=w1539) -> ("error out"=w1536:errorcluster, "FPGA VI Reference Out"=w1537:refnum<k20>)  [unwired: 3 in, 1 out]
            }
            frame Enabled {
            }
          }
          n213 = disable-structure shown="Enabled" {
            disable-tunnel: w1529 -> [w1545 w1547]
            disable-tunnel: w1527 -> [w1544 w1546]
            disable-tunnel: [w1543 w1547] -> w1526
            disable-tunnel: [w1542 w1546] -> w1522
            disable-tunnel: w1514 -> [_ _]
            frame Disabled {
              n214 = call "hModeRegRange2013.vi"("error in"=w1544, "FPGA VI Reference In"=w1545) -> ("error out"=w1542:errorcluster, "FPGA VI Reference Out"=w1543:refnum<k20>)  [unwired: 3 in, 1 out]
            }
            frame Enabled {
            }
          }
          n215 = disable-structure shown="Enabled" {
            disable-tunnel: w1526 -> [w1561 w1563]
            disable-tunnel: w1522 -> [w1560 w1562]
            disable-tunnel: [w1559 w1562] -> w1525
            disable-tunnel: [w1558 w1563] -> w1523
            disable-tunnel: w1515 -> [w1557 _]
            disable-tunnel: w1514 -> [_ _]
            disable-tunnel: w1512 -> [w1556 _]
            frame Enabled {
              n216 = call "hModeRegRange2013.vi"("error in"=w1560, "RangeArray"=w1557, "Mode"=w1556, "FPGA VI Reference In"=w1561) -> ("error out"=w1559:errorcluster, "FPGA VI Reference Out"=w1558:refnum<k20>)  [unwired: 1 in, 1 out]
            }
            frame Disabled {
            }
          }
          n217 = disable-structure shown="Enabled" {
            disable-tunnel: [w1552 w1555] -> w1524
            disable-tunnel: w1525 -> [w1551 w1555]
            disable-tunnel: w1523 -> [w1550 w1554]
            disable-tunnel: [w1553 w1554] -> w1528
            disable-tunnel: w1515 -> [w1549 _]
            disable-tunnel: w1514 -> [_ _]
            disable-tunnel: w1513 -> [w1548 _]
            frame Enabled {
              n218 = call "hModeRegRange2013.vi"("error in"=w1551, "RangeArray"=w1549, "Mode"=w1548, "FPGA VI Reference In"=w1550) -> ("error out"=w1552:errorcluster, "FPGA VI Reference Out"=w1553:refnum<k20>)  [unwired: 1 in, 1 out]
            }
            frame Disabled {
            }
          }
        }
        frame 0 {
          n219 = disable-structure shown="Enabled" {
            disable-tunnel: w1577 -> [w1606 w1607]
            disable-tunnel: w1576 -> [w1605 w1608]
            disable-tunnel: [w1604 w1608] -> w1574
            disable-tunnel: [w1603 w1607] -> w1573
            disable-tunnel: w1564 -> [w1602 _]
            disable-tunnel: w1565 -> [w1601 _]
            frame Enabled {
              n220 = call "hModeReg2014.vi"("error in"=w1606, "Range"=w1602, "Mode"=w1601, "FPGA VI Reference In"=w1605) -> ("error out"=w1603:errorcluster, "FPGA VI Reference Out"=w1604:refnum<k20>)  [unwired: 1 in, 1 out]
            }
            frame Disabled {
            }
          }
          n221 = disable-structure shown="Enabled" {
            disable-tunnel: w1574 -> [w1598 w1600]
            disable-tunnel: w1573 -> [w1597 w1599]
            disable-tunnel: [w1596 w1600] -> w1572
            disable-tunnel: [w1595 w1599] -> w1571
            disable-tunnel: w1564 -> [w1594 _]
            disable-tunnel: w1566 -> [w1593 _]
            frame Enabled {
              n222 = call "hModeReg2014.vi"("error in"=w1597, "Range"=w1594, "Mode"=w1593, "FPGA VI Reference In"=w1598) -> ("error out"=w1595:errorcluster, "FPGA VI Reference Out"=w1596:refnum<k20>)  [unwired: 1 in, 1 out]
            }
            frame Disabled {
            }
          }
          n223 = disable-structure shown="Enabled" {
            disable-tunnel: w1572 -> [w1590 w1592]
            disable-tunnel: w1571 -> [w1589 w1591]
            disable-tunnel: [w1588 w1592] -> w1570
            disable-tunnel: [w1587 w1591] -> w1569
            disable-tunnel: w1564 -> [w1586 _]
            frame Disabled {
              n224 = call "hModeReg2014.vi"("error in"=w1589, "Range"=w1586, "FPGA VI Reference In"=w1590) -> ("error out"=w1587:errorcluster, "FPGA VI Reference Out"=w1588:refnum<k20>)  [unwired: 2 in, 1 out]
            }
            frame Enabled {
            }
          }
          n225 = disable-structure shown="Enabled" {
            disable-tunnel: [w1583 w1584] -> w1575
            disable-tunnel: w1570 -> [w1582 w1585]
            disable-tunnel: w1569 -> [w1581 w1584]
            disable-tunnel: [w1580 w1585] -> w1568
            disable-tunnel: w1564 -> [w1579 _]
            disable-tunnel: w1567 -> [w1578 _]
            frame Enabled {
              n226 = call "hModeReg2014.vi"("error in"=w1581, "Range"=w1579, "Mode"=w1578, "FPGA VI Reference In"=w1582) -> ("error out"=w1583:errorcluster, "FPGA VI Reference Out"=w1580:refnum<k20>)  [unwired: 1 in, 1 out]
            }
            frame Disabled {
            }
          }
        }
        frame 1 {
          n227 = disable-structure shown="Enabled" {
            disable-tunnel: w1621 -> [w1649 w1650]
            disable-tunnel: w1620 -> [w1648 w1651]
            disable-tunnel: [w1647 w1651] -> w1618
            disable-tunnel: [w1646 w1650] -> w1617
            disable-tunnel: w1609 -> [w1645 _]
            frame Disabled {
              n228 = call "hModeReg2014.vi"("error in"=w1649, "Range"=w1645, "FPGA VI Reference In"=w1648) -> ("error out"=w1646:errorcluster, "FPGA VI Reference Out"=w1647:refnum<k20>)  [unwired: 2 in, 1 out]
            }
            frame Enabled {
            }
          }
          n229 = disable-structure shown="Enabled" {
            disable-tunnel: w1618 -> [w1642 w1644]
            disable-tunnel: w1617 -> [w1641 w1643]
            disable-tunnel: [w1640 w1644] -> w1616
            disable-tunnel: [w1639 w1643] -> w1615
            disable-tunnel: w1609 -> [w1638 _]
            frame Disabled {
              n230 = call "hModeReg2014.vi"("error in"=w1641, "Range"=w1638, "FPGA VI Reference In"=w1642) -> ("error out"=w1639:errorcluster, "FPGA VI Reference Out"=w1640:refnum<k20>)  [unwired: 2 in, 1 out]
            }
            frame Enabled {
            }
          }
          n231 = disable-structure shown="Enabled" {
            disable-tunnel: w1616 -> [w1635 w1637]
            disable-tunnel: w1615 -> [w1634 w1636]
            disable-tunnel: [w1633 w1637] -> w1614
            disable-tunnel: [w1632 w1636] -> w1613
            disable-tunnel: w1609 -> [w1631 _]
            disable-tunnel: w1610 -> [w1630 _]
            frame Enabled {
              n232 = call "hModeReg2014.vi"("error in"=w1634, "Range"=w1631, "Mode"=w1630, "FPGA VI Reference In"=w1635) -> ("error out"=w1632:errorcluster, "FPGA VI Reference Out"=w1633:refnum<k20>)  [unwired: 1 in, 1 out]
            }
            frame Disabled {
            }
          }
          n233 = disable-structure shown="Enabled" {
            disable-tunnel: [w1627 w1628] -> w1619
            disable-tunnel: w1614 -> [w1626 w1629]
            disable-tunnel: w1613 -> [w1625 w1628]
            disable-tunnel: [w1624 w1629] -> w1612
            disable-tunnel: w1609 -> [w1623 _]
            disable-tunnel: w1611 -> [w1622 _]
            frame Enabled {
              n234 = call "hModeReg2014.vi"("error in"=w1625, "Range"=w1623, "Mode"=w1622, "FPGA VI Reference In"=w1626) -> ("error out"=w1627:errorcluster, "FPGA VI Reference Out"=w1624:refnum<k20>)  [unwired: 1 in, 1 out]
            }
            frame Disabled {
            }
          }
        }
      }
      n235 = To Double Precision Float(number=w491) -> (double precision float=w496:dbl)
      n236 = Multiply(x=w496, y=w396) -> (x*y=w497:dbl)
      n237 = Multiply(x=w497, y=1000.0) -> (x*y=→"predicted time [ms] to finalize DAQ":dbl)
      n238 = disable-structure shown="Enabled" {
        disable-tunnel: w635 -> [w1194 w1195]
        disable-tunnel: w634 -> [w1193 w1196]
        disable-tunnel: w536 -> [w1192 _]
        disable-tunnel: [w1191 _] -> w615
        disable-tunnel: [w1190 w1195] -> w612
        disable-tunnel: [w1189 w1196] -> w568
        frame Disabled {
          n239 = call "hDACsubtract2013.vi"("FPGA VI Reference In"=w1194, "Ranges"=w1192, "error in"=w1193) -> ("FPGA VI Reference Out"=w1190:refnum<k20>, "DACbits"=w1191:u16[], "error out"=w1189:errorcluster)  [unwired: 10 in]
        }
        frame Enabled {
        }
      }
      n240 = Subtract(x=w615, y=u16 1024 ("NSample")) -> (x-y=→"DACbits 2":u16[])
      n241 = property on="Acquired Samples:" class="Slide (strict)"(error in=w568, "Scale.Range:Maximum"=w491) -> (error out=w567:errorcluster)  [unwired: 1 in, 1 out]
      n242 = local read "Switch to fixed \nCalibration Values"() -> (w689:bool)
      n243 = Scale By Power Of 2(n=w536, x=sgl 10.0 ("Scale(mV)")) -> (x*2^n=w441:sgl[])
      "x*2^n" <- w441
      n244 = disable-structure shown="Enabled" {
        frame Disabled {
          n245 = case shown="False" "SkipVoltageOut" {
            frame True {
            }
            frame False {
              w802 = 5 items=["verify"=2, "reserve"=4, "commit"=3, "unreserve"=5, "abort"=6] ("ending task action")
              w801 = u16 0 items=["OK message + warnings"]
              # "channel preselection for output AO"
              n246 = call-poly <vilib>:"DAQmx Create Virtual Channel.vi"("maximum value"=10.0 ("maximum voltage @ 10MW single channel"), "minimum value"=-1.0, "physical channels"=tag "Dev1/ao0:1" ("Single Channel Output AO")) -> ("task out"=w819:refnum<k21>, "error out"=w816:errorcluster)  [unwired: 11 in]
              n247 = local write "voltage out state"("before SCVO loop") -> ()
              n248 = property class="DAQmx Write" props=["RegenMode", "NumChans"](reference=w819, error in=w816, "RegenMode"="RegenMode") -> (reference out=w817:refnum<k21>, error out=w794:errorcluster)  [unwired: 1 out]
              n249 = property class="DAQmx Channel"(reference=w817, error in=w794, "AO.DataXferReqCond"="AO.DataXferReqCond 2", "AO.DataXferMech"="AO.DataXferMech 2") -> (reference out=w795:refnum<k21>, error out=w793:errorcluster)
              n250 = call-poly <vilib>:"DAQmx Timing.vi"("task/channels in"=w795, "sample mode"="sample mode", "samples per channel"="samples per channel", "rate"="Manual Timing of AO", "source"="source clock", "error in"=w793) -> ("task out"=w785:refnum<k21>, "error out"=w784:errorcluster)  [unwired: 8 in]
              n251 = call-poly <vilib>:"DAQmx Write.vi"("task/channels in"=w785, "data"=dbl[] [0.0, 0.0], "error in"=w784) -> ("task out"=w787:refnum<k21>, "error out"=w786:errorcluster)  [unwired: 10 in, 1 out]
              n252 = Tick Count (ms)() -> (millisecond timer value=w796:u32)
              n253 = while {
                shift-right: [w848] -> w815
                shift-left: w787 -> [w824]
                shift-right: [w847] -> w814
                shift-left: w786 -> [w825]
                tunnel: w796 -> [w831]
                i -> [w827]
                stop <- w844 stop-if-true
                w843 = 9.9 ("AO Cutoff")
                w835 = 0.02 ("y")
                n254 = Tick Count (ms)() -> (millisecond timer value=w832:u32)
                n255 = Subtract(x=w832, y=w831) -> (x-y=w828:u32)
                n256 = Divide(x=w828, y=w827) -> (x/y=→"AO output loop timing":dbl)
                n257 = local write "voltage out state"("inside voltage loop") -> ()
                n258 = local read "single channel voltage"() -> (w839:dbl)
                n259 = Greater Or Equal?(x=w839, y=w843) -> (x >= y?=w840:bool)
                n260 = case shown="True" w840 {
                  tunnel: [w853 w854] -> w833
                  tunnel: w839 -> [w853 _]
                  tunnel: w843 -> [_ w854]
                  frame False {
                  }
                  frame True {
                  }
                }
                n261 = Less Or Equal?(x=w833, y=w835) -> (x <= y?=w837:bool)
                n262 = case shown="True" w837 {
                  tunnel: [w851 0.025 ("AO Cutoff")] -> w823
                  tunnel: w833 -> [w851 _]
                  frame False {
                  }
                  frame True {
                  }
                }
                "SCVO current val" <- w823
                n263 = local read "real time P_rad"() -> (w841:dbl)
                n264 = Greater Or Equal?(x=w841, y=w843) -> (x >= y?=w842:bool)
                n265 = case shown="False" w842 {
                  tunnel: [w855 w856] -> w834
                  tunnel: w841 -> [w855 _]
                  tunnel: w843 -> [_ w856]
                  frame False {
                  }
                  frame True {
                  }
                }
                n266 = Less Or Equal?(x=w834, y=w835) -> (x <= y?=w836:bool)
                n267 = case shown="True" w836 {
                  tunnel: [w849 0.025 ("AO Cutoff")] -> w822
                  tunnel: w834 -> [w849 _]
                  frame False {
                  }
                  frame True {
                  }
                }
                "RTPVO current val" <- w822
                n268 = Build Array(w823, w822) -> (w821:dbl[])
                n269 = local read "Acquired Samples:"() -> (w830:u32)
                n270 = local read "No. of Samples:"() -> (w829:u32)
                n271 = call-poly <vilib>:"DAQmx Write.vi"("task/channels in"=w824, "data"=w821, "error in"=w825) -> ("task out"=w848:refnum<k21>, "error out"=w847:errorcluster)  [unwired: 10 in, 1 out]
                n272 = Unbundle By Name(w825) -> ("status"=w845:bool)  [unwired: 2 out]
                n273 = Greater Or Equal?(x=w830, y=w829) -> (x >= y?=w838:bool)
                n274 = Or(x=w845, y=w838) -> (x .or. y?=w844:bool)
                n275 = Not(x=w844) -> (.not. x?=→"loop status":bool)
                "loop counter" <- w827
                "AO error" <- w825
              }
              n276 = call-poly <vilib>:"DAQmx Write.vi"("task/channels in"=w815, "data"=dbl[] [0.0, 0.0], "error in"=w814) -> ("task out"=w807:refnum<k21>, "error out"=w806:errorcluster)  [unwired: 10 in, 1 out]
              n277 = call <vilib>:"DAQmx Control Task.vi"("task/channels in"=w807, "action"=w802, "error in"=w806) -> ("task out"=w804:refnum<k21>, "error out"=w805:errorcluster)  [unwired: 11 in]
              n278 = call <vilib>:"DAQmx Clear Task.vi"("task in"=w804, "error in"=w805) -> ("error out"=w798:errorcluster)  [unwired: 13 in]
              n279 = call <vilib>:"Simple Error Handler.vi"("type of dialog (OK msg:1)"=w801, "error in (no error)"=w798) -> ()  [unwired: 3 in, 5 out]
              n280 = Unbundle By Name(w798) -> ("status"=→"voltage status":bool, "source"=→"voltage errorsource":string)  [unwired: 1 out]
              "voltage out state" <- "passed SCVO loop"
            }
          }
        }
        frame Disabled {
          n281 = local read "SkipVoltageOut"() -> (w857:bool)
          n282 = case shown="False" w857 {
            frame True {
            }
            frame False {
              w858 = 5 items=["verify"=2, "reserve"=4, "commit"=3, "unreserve"=5, "abort"=6] ("action")
              w870 = u16 0 items=["OK message + warnings"]
              # "channel preselection for output AO"
              n283 = call-poly <vilib>:"DAQmx Create Virtual Channel.vi"("maximum value"=10.0 ("maximum voltage @ 10MW single channel"), "minimum value"=-1.0, "physical channels"=tag "Dev1/ao0:1" ("Single Channel Output AO")) -> ("task out"=w867:refnum<k21>, "error out"=w866:errorcluster)  [unwired: 11 in]
              n284 = local write "voltage out state"("before SCVO loop") -> ()
              n285 = call <vilib>:"DAQmx Start Task.vi"("task/channels in"=w867, "error in"=w866) -> ("task out"=w865:refnum<k21>, "error out"=w864:errorcluster)  [unwired: 12 in]
              n286 = Tick Count (ms)() -> (millisecond timer value=w868:u32)
              n287 = while {
                shift-right: [w905] -> w863
                shift-left: w865 -> [w885]
                shift-right: [w904] -> w862
                shift-left: w864 -> [w880]
                tunnel: w868 -> [w889]
                i -> [w881]
                stop <- w902 stop-if-true
                w901 = 9.9 ("AO Cutoff")
                w893 = 0.02 ("y")
                n288 = Tick Count (ms)() -> (millisecond timer value=w890:u32)
                n289 = Subtract(x=w890, y=w889) -> (x-y=w886:u32)
                n290 = Divide(x=w886, y=w881) -> (x/y=w882:dbl)
                n291 = local write "loop counter"(w881) -> ()
                n292 = local write "AO output loop timing"(w882) -> ()
                n293 = local write "voltage out state"("inside voltage loop") -> ()
                n294 = local read "single channel voltage"() -> (w897:dbl)
                n295 = Greater Or Equal?(x=w897, y=w901) -> (x >= y?=w898:bool)
                n296 = case shown="True" w898 {
                  tunnel: [w910 w911] -> w891
                  tunnel: w897 -> [w910 _]
                  tunnel: w901 -> [_ w911]
                  frame False {
                  }
                  frame True {
                  }
                }
                n297 = Less Or Equal?(x=w891, y=w893) -> (x <= y?=w895:bool)
                n298 = case shown="True" w895 {
                  tunnel: [w908 0.025 ("AO Cutoff")] -> w878
                  tunnel: w891 -> [w908 _]
                  frame False {
                  }
                  frame True {
                  }
                }
                n299 = local write "SCVO current val"(w878) -> ()
                n300 = local read "real time P_rad"() -> (w899:dbl)
                n301 = Greater Or Equal?(x=w899, y=w901) -> (x >= y?=w900:bool)
                n302 = case shown="False" w900 {
                  tunnel: [w912 w913] -> w892
                  tunnel: w899 -> [w912 _]
                  tunnel: w901 -> [_ w913]
                  frame False {
                  }
                  frame True {
                  }
                }
                n303 = Less Or Equal?(x=w892, y=w893) -> (x <= y?=w894:bool)
                n304 = case shown="True" w894 {
                  tunnel: [w906 0.025 ("AO Cutoff")] -> w877
                  tunnel: w892 -> [w906 _]
                  frame False {
                  }
                  frame True {
                  }
                }
                n305 = Build Array(w878, w877) -> (w884:dbl[])
                n306 = local write "RTPVO current val"(w877) -> ()
                n307 = local read "Acquired Samples:"() -> (w888:u32)
                n308 = local read "No. of Samples:"() -> (w887:u32)
                n309 = local write "AO error"(w880) -> ()
                n310 = call-poly <vilib>:"DAQmx Write.vi"("task/channels in"=w885, "data"=w884, "error in"=w880) -> ("task out"=w905:refnum<k21>, "error out"=w904:errorcluster)  [unwired: 10 in, 1 out]
                n311 = Unbundle By Name(w880) -> ("status"=w903:bool)  [unwired: 2 out]
                n312 = Greater Or Equal?(x=w888, y=w887) -> (x >= y?=w896:bool)
                n313 = Or(x=w903, y=w896) -> (x .or. y?=w902:bool)
                n314 = Not(x=w902) -> (.not. x?=w879:bool)
                n315 = local write "loop status"(w879) -> ()
              }
              n316 = local write "voltage out state"("passed SCVO loop") -> ()
              n317 = call <vilib>:"DAQmx Control Task.vi"("task/channels in"=w863, "action"=w858, "error in"=w862) -> ("task out"=w871:refnum<k21>, "error out"=w872:errorcluster)  [unwired: 11 in]
              n318 = call <vilib>:"DAQmx Clear Task.vi"("task in"=w871, "error in"=w872) -> ("error out"=w869:errorcluster)  [unwired: 13 in]
              n319 = call <vilib>:"Simple Error Handler.vi"("type of dialog (OK msg:1)"=w870, "error in (no error)"=w869) -> ()  [unwired: 3 in, 5 out]
              n320 = Unbundle By Name(w869) -> ("status"=w861:bool, "source"=w860:string)  [unwired: 1 out]
              n321 = local write "voltage errorsource"(w860) -> ()
              n322 = local write "voltage status"(w861) -> ()
            }
          }
        }
        frame Enabled {
          n323 = local read "SkipVoltageOut"() -> (w914:bool)
          n324 = case shown="False" w914 {
            frame True {
            }
            frame False {
              w915 = 5 items=["verify"=2, "reserve"=4, "commit"=3, "unreserve"=5, "abort"=6] ("action")
              w927 = u16 0 items=["OK message + warnings"]
              # "channel preselection for output AO"
              n325 = call-poly <vilib>:"DAQmx Create Virtual Channel.vi"("maximum value"=10.0 ("maximum voltage @ 10MW single channel"), "minimum value"=-1.0, "physical channels"=tag "Dev1/ao0:1" ("Single Channel Output AO")) -> ("task out"=w924:refnum<k21>, "error out"=w923:errorcluster)  [unwired: 11 in]
              n326 = local write "voltage out state"("before SCVO loop") -> ()
              n327 = call <vilib>:"DAQmx Start Task.vi"("task/channels in"=w924, "error in"=w923) -> ("task out"=w922:refnum<k21>, "error out"=w921:errorcluster)  [unwired: 12 in]
              n328 = Tick Count (ms)() -> (millisecond timer value=w925:u32)
              n329 = while {
                shift-right: [w963] -> w920
                shift-left: w922 -> [w944]
                shift-right: [w962] -> w919
                shift-left: w921 -> [w939]
                tunnel: w925 -> [w948]
                i -> [w940]
                stop <- w960 stop-if-true
                w959 = 9.9 ("AO Cutoff")
                w952 = 0.02 ("y")
                n330 = Tick Count (ms)() -> (millisecond timer value=w949:u32)
                n331 = Subtract(x=w949, y=w948) -> (x-y=w945:u32)
                n332 = control-ref of="single channel voltage"() -> (w935:refnum<vi>)
                n333 = Divide(x=w945, y=w940) -> (x/y=w941:dbl)
                n334 = local write "loop counter"(w940) -> ()
                n335 = local write "AO output loop timing"(w941) -> ()
                n336 = local write "voltage out state"("inside voltage loop") -> ()
                n337 = property class="DigNum (strict)"(reference=w935) -> ("Value"=w934:dbl)  [unwired: 1 in, 2 out]
                n338 = Greater Or Equal?(x=w934, y=w959) -> (x >= y?=w956:bool)
                n339 = case shown="True" w956 {
                  tunnel: [w968 w969] -> w950
                  tunnel: w934 -> [w968 _]
                  tunnel: w959 -> [_ w969]
                  frame False {
                  }
                  frame True {
                  }
                }
                n340 = Less Or Equal?(x=w950, y=w952) -> (x <= y?=w954:bool)
                n341 = case shown="True" w954 {
                  tunnel: [w966 0.025 ("AO Cutoff")] -> w937
                  tunnel: w950 -> [w966 _]
                  frame False {
                  }
                  frame True {
                  }
                }
                n342 = local write "SCVO current val"(w937) -> ()
                n343 = local read "real time P_rad"() -> (w957:dbl)
                n344 = Greater Or Equal?(x=w957, y=w959) -> (x >= y?=w958:bool)
                n345 = case shown="False" w958 {
                  tunnel: [w970 w971] -> w951
                  tunnel: w957 -> [w970 _]
                  tunnel: w959 -> [_ w971]
                  frame False {
                  }
                  frame True {
                  }
                }
                n346 = Less Or Equal?(x=w951, y=w952) -> (x <= y?=w953:bool)
                n347 = case shown="True" w953 {
                  tunnel: [w964 0.025 ("AO Cutoff")] -> w936
                  tunnel: w951 -> [w964 _]
                  frame False {
                  }
                  frame True {
                  }
                }
                n348 = Build Array(w937, w936) -> (w943:dbl[])
                n349 = local write "RTPVO current val"(w936) -> ()
                n350 = local read "Acquired Samples:"() -> (w947:u32)
                n351 = local read "No. of Samples:"() -> (w946:u32)
                n352 = local write "AO error"(w939) -> ()
                n353 = call-poly <vilib>:"DAQmx Write.vi"("task/channels in"=w944, "data"=w943, "error in"=w939) -> ("task out"=w963:refnum<k21>, "error out"=w962:errorcluster)  [unwired: 10 in, 1 out]
                n354 = Unbundle By Name(w939) -> ("status"=w961:bool)  [unwired: 2 out]
                n355 = Greater Or Equal?(x=w947, y=w946) -> (x >= y?=w955:bool)
                n356 = Or(x=w961, y=w955) -> (x .or. y?=w960:bool)
                n357 = Not(x=w960) -> (.not. x?=w938:bool)
                n358 = local write "loop status"(w938) -> ()
              }
              n359 = local write "voltage out state"("passed SCVO loop") -> ()
              n360 = call <vilib>:"DAQmx Control Task.vi"("task/channels in"=w920, "action"=w915, "error in"=w919) -> ("task out"=w928:refnum<k21>, "error out"=w929:errorcluster)  [unwired: 11 in]
              n361 = call <vilib>:"DAQmx Clear Task.vi"("task in"=w928, "error in"=w929) -> ("error out"=w926:errorcluster)  [unwired: 13 in]
              n362 = call <vilib>:"Simple Error Handler.vi"("type of dialog (OK msg:1)"=w927, "error in (no error)"=w926) -> ()  [unwired: 3 in, 5 out]
              n363 = Unbundle By Name(w926) -> ("status"=w918:bool, "source"=w917:string)  [unwired: 1 out]
              n364 = local write "voltage errorsource"(w917) -> ()
              n365 = local write "voltage status"(w918) -> ()
            }
          }
        }
        frame Disabled {
          n366 = local read "SkipVoltageOut"() -> (w972:bool)
          n367 = case shown="False" w972 {
            frame True {
            }
            frame False {
              w1010 = 5 items=["verify"=2, "reserve"=4, "commit"=3, "unreserve"=5, "abort"=6] ("ending task action 2")
              w1009 = u16 0 items=["OK message + warnings"]
              # "channel preselection for output AO"
              n368 = call "error handler.vi"("Status"=enum16{"Init", "Read"}."Init") -> ("error out"=w1001:errorcluster)  [unwired: 9 in, 1 out]
              n369 = call-poly <vilib>:"DAQmx Create Virtual Channel.vi"("maximum value"=10.0 ("maximum voltage @ 10MW single channel 2"), "minimum value"=-1.0 ("minimum value 2"), "physical channels"=tag "Dev1/ao0:1" ("Single Channel Output AO 2"), "error in"=w1001) -> ("task out"=w1024:refnum<k21>, "error out"=w1022:errorcluster)  [unwired: 10 in]
              n370 = local write "voltage out state"("before SCVO loop") -> ()
              n371 = local read "RegenMode"() -> (w981:i32)
              n372 = property class="DAQmx Write"(reference=w1024, error in=w1022, "RegenMode"=w981) -> (reference out=w1023:refnum<k21>, error out=w1003:errorcluster)
              n373 = local read "AO.DataXferReqCond 2"() -> (w980:i32)
              n374 = local read "AO.DataXferMech 2"() -> (w979:i32)
              n375 = property class="DAQmx Channel"(reference=w1023, error in=w1003, "AO.DataXferReqCond"=w980, "AO.DataXferMech"=w979) -> (reference out=w1004:refnum<k21>, error out=w1002:errorcluster)
              n376 = local read "samples per channel"() -> (w977:i32)
              n377 = local read "sample mode"() -> (w978:i32)
              n378 = local read "Manual Timing of AO"() -> (w982:dbl)
              n379 = local read "source clock"() -> (w1007:tag)
              n380 = call-poly <vilib>:"DAQmx Timing.vi"("task/channels in"=w1004, "sample mode"=w978, "samples per channel"=w977, "rate"=w982, "source"=w1007, "error in"=w1002) -> ("task out"=w1000:refnum<k21>, "error out"=w998:errorcluster)  [unwired: 8 in]
              n381 = call <vilib>:"DAQmx Configure Output Buffer.vi"("task/channels in"=w1000, "buffer size (in samples per channel)"="Samples per channel to write\n(write chunk)", "error in"=w998) -> ("task out"=w999:refnum<k21>, "error out"=w997:errorcluster)  [unwired: 11 in]
              n382 = Initialize Array(0.0 ("element"), 2 ("dimension size"), "Samples per channel to write\n(write chunk)") -> (w994:dbl[][])
              n383 = call-poly <vilib>:"DAQmx Write.vi"("task/channels in"=w999, "data"=w994, "error in"=w997) -> ("task out"=w1005:refnum<k21>, "error out"=w993:errorcluster)  [unwired: 10 in, 1 out]
              n384 = call <vilib>:"DAQmx Start Task.vi"("task/channels in"=w1005, "error in"=w993) -> ("task out"=w991:refnum<k21>, "error out"=w990:errorcluster)  [unwired: 12 in]
              n385 = property class="DAQmx Buffer"(reference=w991, error in=w990) -> (reference out=w992:refnum<k21>, error out=w973:errorcluster, "Output.OnbrdBufSize"=w988:u32, "Output.BufSize"=→"Output.BufSize":u32)
              "Output.OnbrdBufSize" <- w988
              n386 = Tick Count (ms)() -> (millisecond timer value=w1006:u32)
              n387 = while {
                tunnel: w992 -> [w1037]
                tunnel: "Samples per channel to write\n(write chunk)" -> [w1036]
                tunnel: w988 -> [w1035]
                tunnel: w982 -> [w1034]
                tunnel: w988 -> [w1033]
                tunnel: w973 -> [w1030]
                i -> [w1031]
                stop <- w1032 stop-if-true
                n388 = local read "Acquired Samples:"() -> (w1027:u32)
                n389 = local read "No. of Samples:"() -> (w1028:u32)
                n390 = Wait (ms)(milliseconds to wait=u32 10) -> ()  [unwired: 1 out]
                n391 = Decrement(x=w1027) -> (x-1=w1029:u32)
                n392 = Greater Or Equal?(x=w1029, y=w1028) -> (x >= y?=w1026:bool)
                n393 = case shown="True" w1026 {
                  selector: w1026 -> [w1041 w1043]
                  tunnel: w1037 -> [_ w1067]
                  tunnel: w1036 -> [_ w1064]
                  tunnel: w1035 -> [_ w1061]
                  tunnel: w1034 -> [_ w1058]
                  tunnel: w1033 -> [_ w1052]
                  tunnel: [w1038 w1047] -> w1032
                  tunnel: w1031 -> [_ w1045]
                  tunnel: w1030 -> [w1040 w1044]
                  frame False {
                    n394 = local read "voltage watchdog stop"() -> (w1039:bool)
                    n395 = call "error handler.vi"("error in (no error)"=w1040, "error"=w1039) -> ("error"=w1042:bool)  [unwired: 8 in, 1 out]
                    n396 = Or(x=w1041, y=w1042) -> (x .or. y?=w1038:bool)
                  }
                  frame True {
                    w1050 = u8 100 ("y")
                    n397 = property class="DAQmx Write"(reference=w1067, error in=w1044) -> (error out=w1057:errorcluster, "CurrWritePos"=w1066:dbl, "SpaceAvail"=w1062:u32, "TotalSampPerChanGenerated"=w1065:dbl)  [unwired: 1 out]
                    "PC Buffer CurrWritePos 2" <- w1066
                    "PC Buffer SpaceAvail" <- w1062
                    "Board TotalSampPerChanGenerated" <- w1065
                    n398 = Subtract(x=w1061, y=w1062) -> (x-y=w1054:u32)
                    n399 = Subtract(x=w1066, y=w1065) -> (x-y=w1055:dbl)
                    "How many samples stored in the \nPC buffer + board buffer?" <- w1055
                    n400 = call "error handler.vi"("error in (no error)"=w1057, "error"="voltage watchdog stop") -> ("error"=w1046:bool)  [unwired: 8 in, 1 out]
                    n401 = Divide(x=w1055, y=w1064) -> (x/y=→"How many \"Write Chunk\" (periods of latency)\nstored in the PC buffer + board buffer?":dbl)
                    n402 = Divide(x=w1055, y=w1058) -> (x/y=→"How many seconds to empty the \nPC buffer+ board buffer? 2":dbl)
                    n403 = Subtract(x=w1055, y=w1054) -> (x-y=w1053:dbl)
                    n404 = Divide(x=w1054, y=w1061) -> (x/y=w1060:dbl)
                    n405 = Or(x=w1043, y=w1046) -> (x .or. y?=w1047:bool)
                    n406 = Divide(x=w1053, y=w1052) -> (x/y=w1051:dbl)
                    n407 = Multiply(x=w1060, y=w1050) -> (x*y=→"Percentage of PC buffer occupied":dbl)
                    n408 = Multiply(x=w1051, y=w1050) -> (x*y=→"Percentage of OnBoard buffer occupied":dbl)
                    "watchdog loop counter" <- w1045
                  }
                }
              }
              n409 = while {
                shift-right: [w1099] -> w1021
                shift-left: w992 -> [w1075]
                shift-right: [w1098] -> w1020
                shift-left: w973 -> [w1074]
                tunnel: w1006 -> [w1083]
                tunnel: "Samples per channel to write\n(write chunk)" -> [w1078]
                tunnel: [w1078] -> w985
                i -> [w1070]
                stop <- w1096 stop-if-true
                w1095 = 9.9 ("AO Cutoff 2")
                w1087 = 0.02 ("y")
                n410 = Tick Count (ms)() -> (millisecond timer value=w1084:u32)
                n411 = Subtract(x=w1084, y=w1083) -> (x-y=w1080:u32)
                n412 = Divide(x=w1080, y=w1070) -> (x/y=w1071:dbl)
                n413 = local write "AO output loop timing"(w1071) -> ()
                n414 = local write "loop counter"(w1070) -> ()
                n415 = local write "voltage out state"("inside voltage loop") -> ()
                n416 = local read "single channel voltage"() -> (w1091:dbl)
                n417 = Greater Or Equal?(x=w1091, y=w1095) -> (x >= y?=w1092:bool)
                n418 = case shown="True" w1092 {
                  tunnel: [w1104 w1105] -> w1085
                  tunnel: w1091 -> [w1104 _]
                  tunnel: w1095 -> [_ w1105]
                  frame False {
                  }
                  frame True {
                  }
                }
                n419 = Less Or Equal?(x=w1085, y=w1087) -> (x <= y?=w1089:bool)
                n420 = case shown="True" w1089 {
                  tunnel: [w1102 0.025 ("AO Cutoff")] -> w1072
                  tunnel: w1085 -> [w1102 _]
                  frame False {
                  }
                  frame True {
                  }
                }
                n421 = local write "SCVO current val"(w1072) -> ()
                n422 = local read "real time P_rad"() -> (w1093:dbl)
                n423 = Initialize Array(w1072, w1078) -> (w1077:dbl[])
                n424 = Greater Or Equal?(x=w1093, y=w1095) -> (x >= y?=w1094:bool)
                n425 = case shown="False" w1094 {
                  tunnel: [w1106 w1107] -> w1086
                  tunnel: w1093 -> [w1106 _]
                  tunnel: w1095 -> [_ w1107]
                  frame False {
                  }
                  frame True {
                  }
                }
                n426 = Less Or Equal?(x=w1086, y=w1087) -> (x <= y?=w1088:bool)
                n427 = case shown="True" w1088 {
                  tunnel: [w1100 0.025 ("AO Cutoff")] -> w1073
                  tunnel: w1086 -> [w1100 _]
                  frame False {
                  }
                  frame True {
                  }
                }
                n428 = local write "RTPVO current val"(w1073) -> ()
                n429 = Initialize Array(w1073, w1078) -> (w1076:dbl[])
                n430 = Build Array(w1077, w1076) -> (w1079:dbl[][])
                n431 = local read "Acquired Samples:"() -> (w1082:u32)
                n432 = local read "No. of Samples:"() -> (w1081:u32)
                n433 = local write "AO error"(w1074) -> ()
                n434 = call-poly <vilib>:"DAQmx Write.vi"("task/channels in"=w1075, "data"=w1079, "error in"=w1074) -> ("task out"=w1099:refnum<k21>, "error out"=w1098:errorcluster)  [unwired: 10 in, 1 out]
                n435 = Unbundle By Name(w1074) -> ("status"=w1097:bool)  [unwired: 2 out]
                n436 = Greater Or Equal?(x=w1082, y=w1081) -> (x >= y?=w1090:bool)
                n437 = Or(x=w1097, y=w1090) -> (x .or. y?=w1096:bool)
                n438 = Not(x=w1096) -> (.not. x?=w1069:bool)
                n439 = local write "loop status"(w1069) -> ()
              }
              n440 = Initialize Array(0.0 ("element"), 2 ("dimension size"), w985) -> (w984:dbl[][])
              n441 = local write "voltage out state"("passed SCVO loop") -> ()
              n442 = call-poly <vilib>:"DAQmx Write.vi"("task/channels in"=w1021, "data"=w984, "error in"=w1020) -> ("task out"=w1015:refnum<k21>, "error out"=w1014:errorcluster)  [unwired: 10 in, 1 out]
              n443 = call <vilib>:"DAQmx Control Task.vi"("task/channels in"=w1015, "action"=w1010, "error in"=w1014) -> ("task out"=w1012:refnum<k21>, "error out"=w1013:errorcluster)  [unwired: 11 in]
              n444 = call <vilib>:"DAQmx Clear Task.vi"("task in"=w1012, "error in"=w1013) -> ("error out"=w1008:errorcluster)  [unwired: 13 in]
              n445 = call <vilib>:"Simple Error Handler.vi"("type of dialog (OK msg:1)"=w1009, "error in (no error)"=w1008) -> ()  [unwired: 3 in, 5 out]
              n446 = Unbundle By Name(w1008) -> ("status"=w976:bool, "source"=w975:string)  [unwired: 1 out]
              n447 = local write "voltage errorsource"(w975) -> ()
              n448 = local write "voltage status"(w976) -> ()
            }
          }
        }
      }
      n449 = local read "Pre-start time (ms) of\nDAQ Typically set to 1000 ms"() -> (w381:i32)
      n450 = local read "samples to exclude"() -> (w385:u32)
      n451 = Divide(x=w750, y=w677) -> (x/y=w582:dbl[][])
      n452 = local read "No. of Samples:"() -> (w380:u32)
      n453 = local read "SampleTime"() -> (w386:sgl)
      n454 = Initialize Array(0.0, w380) -> (w384:dbl[])
      n455 = Multiply(x=w386, y=w385) -> (x*y=w387:sgl)
      n456 = Divide(x=w381, y=1000) -> (x/y=w388:dbl)
      n457 = local write "Nsample array"(w384) -> ()
      n458 = flat-sequence {
        tunnel: w567 -> [w1258]
        tunnel: w612 -> [w1260]
        tunnel: [w1259] -> w570
        tunnel: [w1257] -> w569
        tunnel: [w1255] -> w464
        tunnel: w463 -> [w1253]
        tunnel: w462 -> [w1254]
        tunnel: w461 -> [w1252]
        tunnel: [w1254] -> w456
        tunnel: [w1253] -> w455
        tunnel: [w1252] -> w454
        tunnel: w441 -> [w1247]
        tunnel: [w1246] -> w440
        tunnel: [w1245] -> w435
        tunnel: w396 -> [w1245]
        tunnel: [w1244] -> w434
        tunnel: w433 -> [w1244]
        tunnel: w570 -> [w1303]
        tunnel: [w1303] -> w564
        tunnel: w569 -> [w1302]
        tunnel: [w1302] -> w562
        tunnel: w529 -> [w1293]
        tunnel: w390 -> [w1289]
        tunnel: w473 -> [w1290]
        tunnel: w376 -> [w1291]
        tunnel: [w1288] -> w469
        tunnel: [w1287] -> w465
        tunnel: w464 -> [w1286]
        tunnel: [w1286] -> w457
        tunnel: w456 -> [w1284]
        tunnel: w455 -> [w1285]
        tunnel: w454 -> [w1283]
        tunnel: [w1285] -> w453
        tunnel: [w1284] -> w452
        tunnel: [w1283] -> w451
        tunnel: w440 -> [w1282]
        tunnel: [w1282] -> w436
        tunnel: w435 -> [w1281]
        tunnel: w434 -> [w1280]
        tunnel: [w1281] -> w429
        tunnel: [w1280] -> w427
        tunnel: w564 -> [w1321]
        tunnel: [w1320] -> w563
        tunnel: w562 -> [w1319]
        tunnel: [w1318] -> w561
        tunnel: w491 -> [w1317]
        tunnel: [w1316] -> w470
        tunnel: w469 -> [w1316]
        tunnel: [w1315] -> w466
        tunnel: w465 -> [w1315]
        tunnel: [w1314] -> w458
        tunnel: w457 -> [w1314]
        tunnel: w453 -> [w1312]
        tunnel: w452 -> [w1313]
        tunnel: w451 -> [w1311]
        tunnel: [w1313] -> w448
        tunnel: [w1312] -> w445
        tunnel: [w1311] -> w442
        tunnel: [w1310] -> w437
        tunnel: w436 -> [w1310]
        tunnel: [w1309] -> w430
        tunnel: w429 -> [w1309]
        tunnel: [w1308] -> w428
        tunnel: w427 -> [w1308]
        tunnel: w563 -> [w1331]
        tunnel: w561 -> [w1332]
        tunnel: w529 -> [w1333]
        tunnel: [w1331] -> w556
        tunnel: [w1332] -> w555
        tunnel: [w1322] -> w471
        tunnel: w470 -> [w1322]
        tunnel: [w1330] -> w467
        tunnel: w466 -> [w1330]
        tunnel: [w1329] -> w459
        tunnel: w458 -> [w1329]
        tunnel: [w1328] -> w449
        tunnel: w448 -> [w1328]
        tunnel: [w1327] -> w446
        tunnel: w445 -> [w1327]
        tunnel: [w1326] -> w443
        tunnel: w442 -> [w1326]
        tunnel: [w1325] -> w438
        tunnel: w437 -> [w1325]
        tunnel: [w1324] -> w431
        tunnel: w430 -> [w1324]
        tunnel: w428 -> [w1323]
        tunnel: [w1323] -> w425
        tunnel: w556 -> [w1348]
        tunnel: w555 -> [w1347]
        tunnel: [w1348] -> w554
        tunnel: [w1347] -> w553
        tunnel: [w1346] -> w552
        tunnel: [w1345] -> w472
        tunnel: w471 -> [w1345]
        tunnel: [w1344] -> w468
        tunnel: w467 -> [w1344]
        tunnel: [w1343] -> w460
        tunnel: w459 -> [w1343]
        tunnel: [w1342] -> w450
        tunnel: w449 -> [w1342]
        tunnel: [w1341] -> w447
        tunnel: w446 -> [w1341]
        tunnel: [w1340] -> w444
        tunnel: w443 -> [w1340]
        tunnel: [w1339] -> w439
        tunnel: w438 -> [w1339]
        tunnel: [w1338] -> w432
        tunnel: w431 -> [w1338]
        tunnel: [w1337] -> w426
        tunnel: w425 -> [w1337]
        tunnel: w554 -> [w1378]
        tunnel: w553 -> [w1379]
        tunnel: w552 -> [w1371]
        tunnel: w491 -> [w1377]
        tunnel: w528 -> [w1367]
        tunnel: w551 -> [w1370]
        tunnel: w424 -> [w1368]
        tunnel: w441 -> [w1369]
        tunnel: [w1376] -> w550
        tunnel: [w1371] -> w549
        tunnel: [w1375] -> w548
        tunnel: [w1374] -> w547
        tunnel: [w1373] -> w546
        tunnel: [w1372] -> w545
        tunnel: w472 -> [w1366]
        tunnel: w468 -> [w1365]
        tunnel: w460 -> [w1363]
        tunnel: w450 -> [w1364]
        tunnel: w447 -> [w1361]
        tunnel: w444 -> [w1362]
        tunnel: w439 -> [w1360]
        tunnel: w432 -> [w1356]
        tunnel: w426 -> [w1355]
        tunnel: w376 -> [w1349]
        tunnel: [w1353] -> w421
        tunnel: [w1352] -> w418
        tunnel: [w1351] -> w406
        tunnel: w549 -> [w1419]
        tunnel: w548 -> [w1418]
        tunnel: w547 -> [w1417]
        tunnel: w546 -> [w1416]
        tunnel: w545 -> [w1415]
        tunnel: [w1419] -> w483
        tunnel: [w1418] -> w482
        tunnel: [w1417] -> w481
        tunnel: [w1416] -> w480
        tunnel: [w1415] -> w479
        tunnel: [w1413] -> w478
        tunnel: [w1412] -> w422
        tunnel: w421 -> [w1412]
        tunnel: [w1411] -> w419
        tunnel: w418 -> [w1411]
        tunnel: [w1410] -> w407
        tunnel: w406 -> [w1410]
        tunnel: w483 -> [w1424]
        tunnel: w482 -> [w1429]
        tunnel: w481 -> [w1428]
        tunnel: w480 -> [w1423]
        tunnel: w479 -> [w1427]
        tunnel: w478 -> [w1425]
        tunnel: [w1429] -> w477
        tunnel: [w1428] -> w476
        tunnel: [w1423] -> w475
        tunnel: [w1427] -> w474
        tunnel: [w1422] -> w423
        tunnel: w422 -> [w1422]
        tunnel: [w1421] -> w420
        tunnel: w419 -> [w1421]
        tunnel: [w1420] -> w408
        tunnel: w407 -> [w1420]
        tunnel: [w1437] -> w543
        tunnel: [w1434] -> w378
        tunnel: [w1433] -> w488
        tunnel: [w1438] -> w544
        tunnel: w477 -> [w1438]
        tunnel: w476 -> [w1435]
        tunnel: w475 -> [w1434]
        tunnel: w474 -> [w1437]
        tunnel: w423 -> [w1432]
        tunnel: w420 -> [w1431]
        tunnel: [w1430] -> w391
        tunnel: w408 -> [w1430]
        frame #0 {
          w1248 = 0.002  # Range=2*RawScale (mV)
          n459 = Multiply(x=w1248, y=w1247) -> (x*y=w1249:dbl[])
          n460 = Scale By Power Of 2 "Volts/bit"(n=i16 -16, x=w1249) -> (x*2^n=w1250:dbl[])
          n461 = To Single Precision Float(number=w1250) -> (single precision float=w1246:sgl[])
          n462 = disable-structure shown="Enabled" {
            disable-tunnel: w1252 -> [w1266 _]
            disable-tunnel: [w1265 _] -> w1255
            disable-tunnel: w1253 -> [w1264 _]
            disable-tunnel: w1254 -> [w1263 _]
            frame Enabled {
              n463 = for {
                N: w1264 -> [_]
                tunnel: w1263 -> [w1275]
                tunnel: w1266 -> [w1273]
                shift-right: [w1267] -> w1265
                shift-left: 0.0 -> [w1268]
                i -> [w1274]
                n464 = Index Array(array=w1273, index (row)=w1274, index (col)=0 ("disabled index (col)")) -> (element=w1270:i64)
                n465 = Index Array(array=w1275, index (row)=w1270, index (col)=1 ("disabled index (col)")) -> (element=w1271:dbl)
                n466 = disable-structure shown="Enabled" {
                  disable-tunnel: w1274 -> [w1278 _]
                  disable-tunnel: w1271 -> [w1277 _]
                  disable-tunnel: w1270 -> [w1276 _]
                  frame Enabled {
                    "volume element" <- w1277
                    "channel selected" <- w1276
                    "iterator" <- w1278
                  }
                  frame Disabled {
                  }
                }
                n467 = Add(x=w1268, y=w1271) -> (x+y=w1267:dbl)
              }
            }
            frame Disabled {
            }
          }
          n468 = call "hComRegStart2013.vi"("error in"=w1258, "FPGA VI Reference In"=w1260) -> ("error out"=w1257:errorcluster, "FPGA VI Reference Out"=w1259:refnum<k20>)  [unwired: 3 in, 1 out]
          n469 = local write "state"("Calibration Done" ("state")) -> ()
          n470 = call "Wait4"("Count(mSec)"=u32 1000) -> ()  [unwired: 1 out]
        }
        frame #1 {
          n471 = local read "Pre-start time (ms) of\nDAQ Typically set to 1000 ms"() -> (w1279:i32)
          n472 = Subtract(x="Fixed T-60sec before T1 = T0", y=w1279) -> (x-y=w1296:i32)
          "Total wait time (TWT) Typically 59 s" <- w1296
          n473 = Tick Count (ms)() -> (millisecond timer value=w1298:u32)
          n474 = Add(x=w1293, y=w1296) -> (x+y=w1295:u32)
          n475 = call "power_factors.vi"("TauM"=w1291, "KappaM"=w1289, "RMESS"=w1290) -> ("F_ch"=w1288:dbl[], "tau_fact"=w1287:dbl[])  [unwired: 7 in]
          "F_ch" <- w1288
          "tau_fact" <- w1287
          n476 = Subtract(x=w1295, y=w1298) -> (x-y=w1299:u32)
          "Calibration Time" <- w1299
          n477 = Subtract(x=w1299, y=u32 50) -> (x-y=w1292:u32)
          "Countdown Time" <- w1292
          n478 = Add(x=w1298, y=w1292) -> (x+y=w1300:u32)
          n479 = while {
            tunnel: w1300 -> [w1306]
            stop <- w1307 continue-if-true
            n480 = Tick Count (ms)() -> (millisecond timer value=w1305:u32)
            n481 = Subtract(x=w1306, y=w1305) -> (x-y=w1304:u32)
            "DAQ Timer" <- w1304
            n482 = Greater?(x=w1306, y=w1305) -> (0:w1307:bool)
            n483 = local write "DAQ Timer"(w1304) -> ()
          }
          n484 = local write "state"("Countdown Timer" ("state")) -> ()
          "V_Cam" <- w1286
        }
        frame #2 {
          # "takes 50 ms"
          n485 = call "hSync&StartSampling2013.vi"("error in"=w1319, "#Samples"=w1317, "FPGA VI Reference In"=w1321) -> ("error out"=w1318:errorcluster, "FPGA VI Reference Out"=w1320:refnum<k20>)  [unwired: 1 in]
        }
        frame #3 {
          n486 = Tick Count (ms)() -> (millisecond timer value=w1334:u32)
          n487 = local write "state"("SyncRun" ("state")) -> ()
          n488 = Subtract(x=w1334, y=w1333) -> (x-y=→"DAQ wait time (should be = TWT":u32)
        }
        frame #4 {
          n489 = call "Tick Count"() -> ("Tick Count(mSec)"=w1346:u32)
        }
        frame #5 {
          # "RTPr factor"
          n490 = local read "single channel signal factor"() -> (w1359:dbl)
          n491 = local read "RTPRad voltage factor"() -> (w1350:dbl)
          n492 = local read "single channel number"() -> (w1358:i64)
          n493 = local read "samples to exclude"() -> (w1357:u32)
          n494 = Bundle("Array"=w1370, w1369, "Array 2"=w1368, "Tau00"=w1367, "F_ch"=w1366, "tau_fact"=w1365, "all rows"=w1364, w1363, w1360, "single channel signal factor"=w1359, "RTPRad voltage factor"=w1350, "SampleTime"=w1356, w1355, "ArrayOutput"=w1349, "all rows"=w1362, w1361, "single channel number"=w1358, "samples to exclude"=w1357) -> (w1354:T48)  [unwired: 1 in]
          n495 = disable-structure shown="Enabled" {
            disable-tunnel: w1379 -> [w1401 w1408]
            disable-tunnel: w1378 -> [w1400 w1409]
            disable-tunnel: w1377 -> [w1393 w1407]
            disable-tunnel: [w1399 w1406] -> w1375
            disable-tunnel: [w1398 w1405] -> w1372
            disable-tunnel: [w1397 _] -> w1376
            disable-tunnel: [w1396 _] -> w1374
            disable-tunnel: [w1395 w1403] -> w1373
            disable-tunnel: w1354 -> [w1381 _]
            disable-tunnel: [w1387 _] -> w1353
            disable-tunnel: [w1386 _] -> w1352
            disable-tunnel: [w1382 _] -> w1351
            frame Enabled {
              n496 = control-ref of="real time P_rad array"() -> (w1391:refnum<vi>)
              n497 = control-ref of="single channel voltage"() -> (w1390:refnum<vi>)
              n498 = control-ref of="real time P_rad"() -> (w1392:refnum<vi>)
              n499 = control-ref of="single channel voltage array"() -> (w1389:refnum<vi>)
              n500 = Bundle("real time P_rad"=w1392, "real time P_rad array"=w1391, "single channel voltage"=w1390, "single channel voltage array"=w1389) -> (w1388:T49)  [unwired: 1 in]
              n501 = call "hReadChannels-UandP-2013.vi"("FPGA VI Reference In"=w1400, "SavGol side points"="SavGol side points", "Use Voltage or Power for AO?"="Use Voltage or Power for\nsingel channel AO?", "order polynomial"="order polynomial", "Nsamples"=w1393, "error in"=w1401, "output cluster"=w1388, "variables cluster"=w1381) -> ("Fehler"=w1397:bool, "AdjustedArray"=w1382:sgl[][], "single channel voltage array"=w1386:dbl[], "real time P_rad array"=w1387:dbl[], "FPGA VI Reference Out"=w1399:refnum<k20>, "PowerArray"=w1396:sgl[][], "RawArray"=w1395:sgl[][], "error out"=w1398:errorcluster)  [unwired: 12 in]
              "single channel voltage array" <- w1386
              "real time P_rad array" <- w1387
              n502 = local write "state"("Acquiring Data..." ("state")) -> ()
              "voltage on\nsingle channel AO" <- "Use Voltage or Power for\nsingel channel AO?"
            }
            frame Disabled {
              n503 = call "hReadChannelsRTDMA2013.vi"("FPGA VI Reference In"=w1409, "Nsamples"=w1407, "error in"=w1408) -> ("FPGA VI Reference Out"=w1406:refnum<k20>, "RawArray"=w1404:i16[][], "error out"=w1405:errorcluster)  [unwired: 2 in, 1 out]
              n504 = call "Int2Volt2D.vi"("IntegerArray"=w1404, "Scale(mV)"=sgl 80.0) -> ("RealArray"=w1403:sgl[][])
            }
          }
          n505 = disable-structure shown="Disabled" {
            disable-tunnel: w1354 -> [w1380 _]
            frame Disabled {
              "variables cluster" <- w1380
            }
            frame Enabled {
            }
          }
        }
        frame #6 {
          n506 = call "Tick Count2"() -> ("Tick Count(mSec)"=w1413:u32)
          n507 = local write "state"("Acquiring done" ("state")) -> ()
        }
        frame #7 {
          n508 = Subtract(x=w1425, y=w1424) -> (x-y=→"Measured Time for DAQ [ms]":u32)
        }
        frame #8 {
          n509 = disable-structure shown="Enabled" {
            disable-tunnel: w1435 -> [w1439 w1456]
            disable-tunnel: [w1439 w1450] -> w1433
            disable-tunnel: w1432 -> [_ w1444]
            disable-tunnel: w1431 -> [_ w1445]
            frame Disabled {
            }
            frame Enabled {
              n510 = local read "kbolott_and_volume"() -> (w1452:dbl[][])
              n511 = local read "samples to exclude"() -> (w1454:u32)
              n512 = local read "No. of Samples:"() -> (w1455:u32)
              n513 = local read "Nsample array"() -> (w1443:dbl[])
              n514 = Subtract(x=w1455, y=w1454) -> (x-y=w1453:u32)
              n515 = call "rawpower2totalprad.vi"("PowerArray [W]"=w1456, "No. of Samples\n[TOA / Sample Rate]"=w1453, "kbolott_and_volume"=w1452) -> ("full P_rad [MW] HBC"=w1451:dbl[], "full P_rad [MW] VBC"=w1442:dbl[], "corrected PowerArray"=w1450:dbl[][])
              "full P_rad [MW] HBC" <- w1451
              "full P_rad [MW] VBC" <- w1442
              n516 = Bundle("Nsample array"=w1443, "full P_rad [MW] HBC"=w1451) -> (→"full P_rad plot":T7)  [unwired: 1 in]
              n517 = Bundle("Nsample array"=w1443, "single channel voltage array"=w1445) -> ()  [unwired: 1 in, 1 out]
              n518 = Bundle("Nsample array"=w1443, "real time P_rad array"=w1444) -> ()  [unwired: 1 in, 1 out]
              n519 = Bundle("Nsample array"=w1443, "full P_rad [MW] VBC"=w1442) -> ()  [unwired: 1 in, 1 out]
              n520 = Build Cluster Array(w1443, w1451) -> (w1446:cluster{dbl, "element":dbl}[])
              n521 = Build Cluster Array(w1443, w1444) -> (w1448:cluster{dbl, "element":dbl}[])
              n522 = Build Cluster Array(w1443, w1445) -> (w1449:cluster{dbl, "element":dbl}[])
              n523 = Build Cluster Array(w1443, w1442) -> (w1441:cluster{dbl, "element":dbl}[])
              n524 = Build Cluster Array(w1446, w1449, w1448, w1441) -> (→"all plot":cluster{cluster{dbl, "element":dbl}[]}[])
            }
          }
          n525 = local write "state"("Calculating full radiated power of HBCm ..." ("state")) -> ()
        }
      }
      n526 = for {
        N: w380 -> [_]
        shift-right: [w767] -> w383
        shift-left: w384 -> [w766]
        tunnel: w386 -> [w765]
        tunnel: w387 -> [w759]
        tunnel: w388 -> [w761]
        i -> [w763]
        n527 = To Double Precision Float(number=w763) -> (double precision float=w764:dbl)
        n528 = Multiply(x=w765, y=w764) -> (x*y=w762:dbl)
        n529 = Subtract(x=w762, y=w761) -> (x-y=w760:dbl)
        n530 = Add(x=w760, y=w759) -> (x+y=w758:dbl)
        n531 = Replace Array Subset(array=w766, new element=w758, index=w763) -> (w767:dbl[])
      }
      n532 = call "CalFaktor-128.vi"("CalCurrent(t)"=w582, "Rload"=w677, "Rcable"=w539) -> ("FitData"=w377:dbl[][], "Kappa"=w390:dbl[], "Tau"=w578:dbl[], "RB01"=w522:dbl[])  [unwired: 1 out]
      "KappaM" <- w390
      n533 = local write "Nsample array"(w383) -> ()
      n534 = call "Cal(SubVI)-2013.vi"("Array"=w582, "dt"=w696, "StartChan"=64 ("ChanStart"), "tstart"=w697, "FitData"=w377) -> ("plot(Signals) 1-32"=→"MessCal 65 - 80":T50, "plot(Signals) 33-64"=→"MessCal 81 - 96":T51)  [unwired: 9 in]
      n535 = call "Cal(SubVI)-2013.vi"("Array"=w582, "dt"=w696, "StartChan"=96 ("ChanStart"), "tstart"=w697, "FitData"=w377) -> ("plot(Signals) 1-32"=→"MessCal 97 - 112":T50, "plot(Signals) 33-64"=→"MessCal 113 - 128":T51)  [unwired: 9 in]
      n536 = call "Cal(SubVI)-2013.vi"("Array"=w582, "dt"=w696, "StartChan"=32 ("ChanStart"), "tstart"=w697, "FitData"=w377) -> ("plot(Signals) 1-32"=→"MessCal 33 - 49":T50, "plot(Signals) 33-64"=→"MessCal 49 - 64":T51)  [unwired: 9 in]
      n537 = call "Cal(SubVI)-2013.vi"("Array"=w582, "dt"=w696, "StartChan"=0 ("ChanStart"), "tstart"=w697, "FitData"=w377) -> ("plot(Signals) 1-32"=→"MessCal 1-16":T50, "plot(Signals) 33-64"=→"MessCal 17-32":T51)  [unwired: 9 in]
      n538 = Array Subset(array=w582, index (row)=0 ("index"), length (row)=128 ("length")) -> (w581:dbl[][])  [unwired: 2 in]
      n539 = case shown="True" w689 {
        tunnel: [w1653 "RB000"] -> w375
        tunnel: [w1652 "Kappa00"] -> w673
        tunnel: [w1654 "Tau00"] -> w528
        tunnel: w578 -> [w1654 _]
        tunnel: w522 -> [w1653 _]
        tunnel: w390 -> [w1652 _]
        frame False {
        }
        frame True {
        }
      }
      n540 = call "Arraylimit128.vi"("LowerLimit"=400.0, "Array Input"=w522, "UpperLimit"=2000.0) -> ("BoolArray"=w741:bool[], "ArrayOutput"=w473:dbl[])
      "RMESS" <- w473
      n541 = call "Arraylimit128.vi"("LowerLimit"=2e-05, "Array Input"=w390, "UpperLimit"=0.002) -> ("BoolArray"=w743:bool[])  [unwired: 1 out]
      n542 = call "Arraylimit128.vi"("LowerLimit"=0.001, "Array Input"=w578, "UpperLimit"=0.8) -> ("BoolArray"=w742:bool[], "ArrayOutput"=w376:dbl[])
      "TauM" <- w376
      n543 = Add(x=w539, y=w677) -> (x+y=w676:dbl)
      n544 = Multiply(x=w676, y=2.0) -> (x*y=w674:dbl)
      n545 = call "U2PCoeff.vi"("Numeric"=w674, "Kappa00"=w673, "RB000"=w375) -> ("Array"=w551:dbl[], "Array 2"=w424:dbl[])
      n546 = Compound Arithmetic op=OR(w743, w742, w741) -> (w726:bool[])
      n547 = Array Subset(array=w726, index=0, length=32) -> (→"MessStatus 1-32":bool[])
      n548 = Array Subset(array=w726, index=32, length=32) -> (→"MessStatus 33-64":bool[])
      n549 = Array Subset(array=w726, index=96, length=32) -> (→"MessStatus 97-128":bool[])
      n550 = Array Subset(array=w726, index=64, length=32) -> (→"MessStatus 65-96":bool[])
      n551 = Divide(x=w701, y=w677) -> (x/y=w590:dbl[][])
      n552 = call "CalFaktor-128.vi"("CalCurrent(t)"=w590, "Rload"=w677, "Rcable"=w539) -> ("FitData"=w540:dbl[][], "Kappa"=w523:dbl[], "Tau"=w576:dbl[], "RB01"=w577:dbl[])  [unwired: 1 out]
      n553 = local read "Pre-start time (ms) of\nDAQ Typically set to 1000 ms"() -> (w566:i32)
      n554 = local read "samples to exclude"() -> (w416:u32)
      n555 = local read "SampleTime"() -> (w417:sgl)
      n556 = Multiply(x=w417, y=w416) -> (x*y=w413:sgl)
      n557 = Divide(x=w566, y=sgl -1000.0 ("Scale(mV)")) -> (x/y=w415:sgl)
      n558 = Multiply(x=w413, y="timing of plots fix factor") -> (x*y=w414:sgl)
      n559 = Add(x=w415, y=w414) -> (x+y=w397:sgl)
      "T-Start [for Display)\nShould be -1 [s]" <- w397
      n560 = Array Subset(array=w590, index (row)=0 ("index"), length (row)=128 ("length")) -> (w484:dbl[][])  [unwired: 2 in]
      n561 = call "Arraylimit128.vi"("LowerLimit"=2e-05, "Array Input"=w523, "UpperLimit"=0.002) -> ("BoolArray"=w708:bool[], "ArrayOutput"=→"KappaR":dbl[])
      n562 = call "Arraylimit128.vi"("LowerLimit"=0.001, "Array Input"=w576, "UpperLimit"=0.8) -> ("BoolArray"=w709:bool[], "ArrayOutput"=w524:dbl[])
      "TauR" <- w524
      n563 = Array Subset(array=w391, index (row)=64, length (row)=64, index (col)=0) -> (w398:sgl[][])  [unwired: 1 in]
      n564 = Array Subset(array=w391, index (row)=0, length (row)=64, index (col)=0) -> (w399:sgl[][])  [unwired: 1 in]
      n565 = call "Cal(SubVI)-2013.vi"("Array"=w590, "dt"=w692, "StartChan"=0 ("ChanStart"), "tstart"=w693, "FitData"=w540) -> ("plot(Signals) 1-32"=→"RefCal 1-16":T50, "plot(Signals) 33-64"=→"RefCal 17-32":T51)  [unwired: 9 in]
      n566 = call "Cal(SubVI)-2013.vi"("Array"=w590, "dt"=w692, "StartChan"=32 ("ChanStart"), "tstart"=w693, "FitData"=w540) -> ("plot(Signals) 1-32"=→"RefCal 33 - 48":T50, "plot(Signals) 33-64"=→"RefCal 49 - 64":T51)  [unwired: 9 in]
      n567 = call "Cal(SubVI)-2013.vi"("Array"=w590, "dt"=w692, "StartChan"=64 ("ChanStart"), "tstart"=w693, "FitData"=w540) -> ("plot(Signals) 1-32"=→"RefCal 65 - 80":T50, "plot(Signals) 33-64"=→"RefCal 81 - 96":T51)  [unwired: 9 in]
      n568 = call "Cal(SubVI)-2013.vi"("Array"=w590, "dt"=w692, "StartChan"=96 ("ChanStart"), "tstart"=w693, "FitData"=w540) -> ("plot(Signals) 1-32"=→"RefCal 97 - 112":T50, "plot(Signals) 33-64"=→"RefCal 113 - 128":T51)  [unwired: 9 in]
      n569 = Array Subset(array=w540, index (row)=0 ("index"), length (row)=128 ("length")) -> (w585:dbl[][])  [unwired: 2 in]
      n570 = call "Visualize_Signals64.vi"("FPGSampleTime"=w396, "tstart"=w397, "Signals"=w398) -> ("plot(Signals) 33-64"=→"Adjusted 97 - 129":T47, "plot(Signals) 1-32"=→"Adjusted 65 - 98":T4)  [unwired: 7 in]
      n571 = call "Visualize_Signals64.vi"("FPGSampleTime"=w396, "tstart"=w397, "Signals"=w399) -> ("plot(Signals) 33-64"=→"Adjusted 33-64":T47, "plot(Signals) 1-32"=→"Adjusted 1-32":T4)  [unwired: 7 in]
      n572 = call "Arraylimit128.vi"("LowerLimit"=400.0, "Array Input"=w577, "UpperLimit"=2000.0) -> ("BoolArray"=w710:bool[], "ArrayOutput"=w558:dbl[])
      "RREF" <- w558
      n573 = Array Size(array=w378) -> (size(s)=→"BoloSignalRaw Sizes (debug)":i32[])
      n574 = Array Subset(array=w488, index (row)=0 ("index"), length (row)=128 ("length")) -> (w487:dbl[][])  [unwired: 2 in]
      n575 = Array Subset(array=w488, index (row)=64, length (row)=64, index (col)=0) -> (w663:dbl[][])  [unwired: 1 in]
      n576 = Array Subset(array=w488, index (row)=0, length (row)=64, index (col)=0) -> (w667:dbl[][])  [unwired: 1 in]
      n577 = Array Subset(array=w378, index (row)=0 ("index"), length (row)=128 ("length")) -> (w559:sgl[][])  [unwired: 2 in]
      n578 = Array Subset(array=w378, index (row)=64, length (row)=64, index (col)=0) -> (w560:sgl[][])  [unwired: 1 in]
      n579 = Array Subset(array=w378, index (row)=0, length (row)=64, index (col)=0) -> (w557:sgl[][])  [unwired: 1 in]
      n580 = call "Visualize_Signals64.vi"("FPGSampleTime"=w396, "tstart"=w397, "Signals"=w663) -> ("plot(Signals) 33-64"=→"Pow 97 - 128":T47, "plot(Signals) 1-32"=→"Pow 65 - 96":T4)  [unwired: 7 in]
      n581 = call "Visualize_Signals64.vi"("FPGSampleTime"=w396, "tstart"=w397, "Signals"=w667) -> ("plot(Signals) 33-64"=→"Pow 33-64":T47, "plot(Signals) 1-32"=→"Pow 1-32":T4)  [unwired: 7 in]
      n582 = call "Visualize_Signals64.vi"("FPGSampleTime"=w396, "tstart"=w397, "Signals"=w560) -> ("plot(Signals) 33-64"=→"Raw 97 - 128":T47, "plot(Signals) 1-32"=→"Raw 65 - 97":T4)  [unwired: 7 in]
      n583 = call "Visualize_Signals64.vi"("FPGSampleTime"=w396, "tstart"=w397, "Signals"=w557) -> ("plot(Signals) 33-64"=→"Raw 33-64":T47, "plot(Signals) 1-32"=→"Raw 1-32":T4)  [unwired: 7 in]
      n584 = Compound Arithmetic op=OR(w708, w709, w710) -> (w725:bool[])
      n585 = Array Subset(array=w377, index (row)=0 ("index"), length (row)=128 ("length")) -> (w525:dbl[][])  [unwired: 2 in]
      n586 = Array Subset(array=w725, index=0, length=32) -> (→"RefStatus 1-32":bool[])
      n587 = Array Subset(array=w725, index=32, length=32) -> (→"RefStatus 33-64":bool[])
      n588 = Array Subset(array=w725, index=64, length=32) -> (→"RefStatus 65-96":bool[])
      n589 = Array Subset(array=w725, index=96, length=32) -> (→"RefStatus 97-128":bool[])
      n590 = disable-structure shown="Disabled" {
        disable-tunnel: w378 -> [w1175 _]
        disable-tunnel: w524 -> [w1174 _]
        disable-tunnel: w523 -> [w1173 _]
        disable-tunnel: w558 -> [w1172 _]
        disable-tunnel: w557 -> [w1171 _]
        disable-tunnel: w376 -> [w1170 _]
        disable-tunnel: w390 -> [w1169 _]
        disable-tunnel: w473 -> [w1168 _]
        disable-tunnel: w397 -> [w1167 _]
        disable-tunnel: w396 -> [w1166 _]
        frame Disabled {
          n591 = call "W7-X-Bolo-TMDS-LOCAL.vi"("Kappa 2"=w1173, "ArrayOutput 4"=w1174, "ArrayOutput 3"=w1172, "Array"=w1171, "RawArray"=w1175, "Numeric"=w1167, "ArrayOutput"=w1168, "Kappa"=w1169, "ArrayOutput 2"=w1170, "SampleTime"=w1166) -> ()  [unwired: 5 in, 1 out]
        }
        frame Enabled {
        }
      }
      "Fehler READ U+P" <- w550
    }
    frame True {
      n592 = local write "state"("Error->NoRead" ("state")) -> ()
    }
  }
  n593 = Multiply(x=w153, y=w152) -> (x*y=w135:i64)
  n594 = xnode "Read/Write Control"("FPGA VI Reference In"=w176) -> ("FPGA VI Reference Out"=w175:refnum<k20>, "SampleTrigger2"=w177:u32)  [unwired: 1 in, 1 out]
  n595 = To Quad Integer(1:w177) -> (0:w171:i64)
  "Presamples If -1, then no trigger detected)" <- w171
  n596 = flat-sequence {
    tunnel: w179 -> [w1699]
    tunnel: w215 -> [w1700]
    tunnel: w175 -> [w1701]
    tunnel: [w1701] -> w174
    tunnel: [w1700] -> w173
    tunnel: [w1699] -> w172
    tunnel: w135 -> [w1698]
    tunnel: w171 -> [w1697]
    tunnel: w151 -> [w1676]
    tunnel: w150 -> [w1675]
    tunnel: w149 -> [w1674]
    tunnel: w148 -> [w1673]
    tunnel: w147 -> [w1672]
    tunnel: w146 -> [w1671]
    tunnel: w145 -> [w1670]
    tunnel: [w1694] -> w144
    tunnel: [w1693] -> w143
    tunnel: [w1692] -> w142
    tunnel: [w1691] -> w141
    tunnel: [w1690] -> w140
    tunnel: [w1689] -> w139
    tunnel: [w1688] -> w138
    tunnel: [w1687] -> w137
    tunnel: [w1686] -> w136
    tunnel: w135 -> [w1686]
    tunnel: [w1685] -> w131
    tunnel: [w1683] -> w126
    tunnel: w67 -> [w1683]
    tunnel: [w1684] -> w123
    tunnel: w122 -> [w1684]
    tunnel: [w1682] -> w120
    tunnel: w119 -> [w1682]
    tunnel: [w1681] -> w117
    tunnel: w116 -> [w1681]
    tunnel: [w1680] -> w114
    tunnel: w94 -> [w1680]
    tunnel: [w1679] -> w93
    tunnel: w90 -> [w1679]
    tunnel: [w1678] -> w65
    tunnel: [w1677] -> w58
    tunnel: [w1676] -> w54
    tunnel: [w1675] -> w53
    tunnel: [w1674] -> w52
    tunnel: [w1673] -> w51
    tunnel: [w1672] -> w50
    tunnel: [w1671] -> w49
    tunnel: [w1670] -> w48
    tunnel: [w1669] -> w47
    tunnel: [w1668] -> w46
    tunnel: [w1667] -> w17
    tunnel: [w1666] -> w10
    tunnel: [w1662] -> w6
    tunnel: [w1661] -> w2
    tunnel: w1 -> [w1661]
    tunnel: [w1745] -> w170
    tunnel: [w1744] -> w169
    tunnel: [w1743] -> w168
    tunnel: w174 -> [w1745]
    tunnel: w173 -> [w1744]
    tunnel: w172 -> [w1743]
    tunnel: w144 -> [w1732]
    tunnel: w143 -> [w1731]
    tunnel: w142 -> [w1730]
    tunnel: w141 -> [w1729]
    tunnel: w140 -> [w1728]
    tunnel: w139 -> [w1727]
    tunnel: w138 -> [w1726]
    tunnel: w137 -> [w1725]
    tunnel: w136 -> [w1738]
    tunnel: [w1739] -> w132
    tunnel: w131 -> [w1739]
    tunnel: [w1738] -> w130
    tunnel: [w1737] -> w127
    tunnel: w126 -> [w1737]
    tunnel: [w1736] -> w124
    tunnel: w123 -> [w1736]
    tunnel: [w1735] -> w121
    tunnel: w120 -> [w1735]
    tunnel: [w1734] -> w118
    tunnel: w117 -> [w1734]
    tunnel: [w1733] -> w115
    tunnel: w114 -> [w1733]
    tunnel: [w1732] -> w109
    tunnel: [w1731] -> w107
    tunnel: [w1730] -> w105
    tunnel: [w1729] -> w103
    tunnel: [w1728] -> w101
    tunnel: [w1727] -> w99
    tunnel: [w1726] -> w97
    tunnel: [w1725] -> w95
    tunnel: w93 -> [w1724]
    tunnel: [w1724] -> w92
    tunnel: w65 -> [w1723]
    tunnel: [w1723] -> w62
    tunnel: [w1722] -> w59
    tunnel: w58 -> [w1722]
    tunnel: w54 -> [w1713]
    tunnel: w53 -> [w1714]
    tunnel: w52 -> [w1715]
    tunnel: w51 -> [w1716]
    tunnel: w50 -> [w1717]
    tunnel: w49 -> [w1718]
    tunnel: w48 -> [w1719]
    tunnel: w47 -> [w1720]
    tunnel: w46 -> [w1721]
    tunnel: [w1721] -> w45
    tunnel: [w1720] -> w44
    tunnel: [w1719] -> w43
    tunnel: [w1718] -> w42
    tunnel: [w1717] -> w41
    tunnel: [w1716] -> w40
    tunnel: [w1715] -> w39
    tunnel: [w1714] -> w38
    tunnel: [w1713] -> w37
    tunnel: w17 -> [w1712]
    tunnel: [w1712] -> w16
    tunnel: [w1711] -> w11
    tunnel: w10 -> [w1711]
    tunnel: [w1710] -> w7
    tunnel: w6 -> [w1710]
    tunnel: [w1709] -> w3
    tunnel: w2 -> [w1709]
    tunnel: w170 -> [w1792]
    tunnel: [w1792] -> w167
    tunnel: w169 -> [w1791]
    tunnel: [w1791] -> w166
    tunnel: w168 -> [w1790]
    tunnel: [w1790] -> w164
    tunnel: [w1786] -> w134
    tunnel: [w1785] -> w133
    tunnel: w132 -> [w1785]
    tunnel: w130 -> [w1784]
    tunnel: [w1784] -> w129
    tunnel: [w1783] -> w128
    tunnel: w127 -> [w1783]
    tunnel: [w1782] -> w125
    tunnel: w124 -> [w1782]
    tunnel: w121 -> [w1780]
    tunnel: w118 -> [w1779]
    tunnel: w115 -> [w1781]
    tunnel: [w1781] -> w113
    tunnel: [w1780] -> w112
    tunnel: [w1779] -> w111
    tunnel: [w1778] -> w110
    tunnel: w109 -> [w1778]
    tunnel: [w1777] -> w108
    tunnel: w107 -> [w1777]
    tunnel: [w1776] -> w106
    tunnel: w105 -> [w1776]
    tunnel: [w1775] -> w104
    tunnel: w103 -> [w1775]
    tunnel: [w1774] -> w102
    tunnel: w101 -> [w1774]
    tunnel: [w1773] -> w100
    tunnel: w99 -> [w1773]
    tunnel: [w1772] -> w98
    tunnel: w97 -> [w1772]
    tunnel: [w1771] -> w96
    tunnel: w95 -> [w1771]
    tunnel: w92 -> [w1770]
    tunnel: [w1770] -> w91
    tunnel: [w1760] -> w63
    tunnel: w62 -> [w1760]
    tunnel: [w1759] -> w60
    tunnel: w59 -> [w1759]
    tunnel: w45 -> [w1750]
    tunnel: w44 -> [w1751]
    tunnel: w43 -> [w1752]
    tunnel: w42 -> [w1753]
    tunnel: w41 -> [w1754]
    tunnel: w40 -> [w1755]
    tunnel: w39 -> [w1756]
    tunnel: w38 -> [w1757]
    tunnel: w37 -> [w1758]
    tunnel: [w1758] -> w35
    tunnel: [w1757] -> w33
    tunnel: [w1756] -> w31
    tunnel: [w1755] -> w29
    tunnel: [w1754] -> w27
    tunnel: [w1753] -> w25
    tunnel: [w1752] -> w23
    tunnel: [w1751] -> w21
    tunnel: [w1750] -> w19
    tunnel: w16 -> [w1749]
    tunnel: [w1749] -> w14
    tunnel: [w1748] -> w12
    tunnel: w11 -> [w1748]
    tunnel: [w1747] -> w8
    tunnel: w7 -> [w1747]
    tunnel: [w1746] -> w4
    tunnel: w3 -> [w1746]
    tunnel: w167 -> [w1855]
    tunnel: w166 -> [w1854]
    tunnel: [w1854] -> w165
    tunnel: w164 -> [w1856]
    tunnel: [w1856] -> w163
    tunnel: w134 -> [w1807]
    tunnel: w133 -> [w1868]
    tunnel: w129 -> [w1803]
    tunnel: w128 -> [w1867]
    tunnel: w125 -> [w1866]
    tunnel: w113 -> [w1845]
    tunnel: w112 -> [w1844]
    tunnel: w111 -> [w1843]
    tunnel: w110 -> [w1864]
    tunnel: w108 -> [w1863]
    tunnel: w106 -> [w1862]
    tunnel: w104 -> [w1861]
    tunnel: w102 -> [w1860]
    tunnel: w100 -> [w1859]
    tunnel: w98 -> [w1858]
    tunnel: w96 -> [w1857]
    tunnel: w91 -> [w1865]
    tunnel: [w1845] -> w86
    tunnel: [w1844] -> w85
    tunnel: [w1867] -> w84
    tunnel: [w1866] -> w83
    tunnel: [w1865] -> w82
    tunnel: [w1864] -> w81
    tunnel: [w1863] -> w80
    tunnel: [w1862] -> w79
    tunnel: [w1861] -> w78
    tunnel: [w1860] -> w77
    tunnel: [w1859] -> w76
    tunnel: [w1858] -> w75
    tunnel: [w1857] -> w74
    tunnel: [w1855] -> w73
    tunnel: [w1853] -> w72
    tunnel: [w1852] -> w71
    tunnel: [w1851] -> w70
    tunnel: [w1850] -> w69
    tunnel: [w1849] -> w68
    tunnel: [w1843] -> w66
    tunnel: [w1827] -> w64
    tunnel: w63 -> [w1827]
    tunnel: [w1826] -> w61
    tunnel: w60 -> [w1826]
    tunnel: [w1825] -> w36
    tunnel: w35 -> [w1825]
    tunnel: [w1824] -> w34
    tunnel: w33 -> [w1824]
    tunnel: [w1823] -> w32
    tunnel: w31 -> [w1823]
    tunnel: [w1822] -> w30
    tunnel: w29 -> [w1822]
    tunnel: [w1821] -> w28
    tunnel: w27 -> [w1821]
    tunnel: [w1820] -> w26
    tunnel: w25 -> [w1820]
    tunnel: [w1819] -> w24
    tunnel: w23 -> [w1819]
    tunnel: [w1818] -> w22
    tunnel: w21 -> [w1818]
    tunnel: [w1817] -> w20
    tunnel: w19 -> [w1817]
    tunnel: [w1808] -> w18
    tunnel: [w1804] -> w15
    tunnel: w14 -> [w1804]
    tunnel: [w1802] -> w13
    tunnel: w12 -> [w1802]
    tunnel: [w1801] -> w9
    tunnel: w8 -> [w1801]
    tunnel: [w1800] -> w5
    tunnel: w4 -> [w1800]
    tunnel: w165 -> [w1924]
    tunnel: w163 -> [w1926]
    tunnel: [w1926] -> w89
    tunnel: [w1925] -> w88
    tunnel: [w1924] -> w87
    tunnel: w86 -> [w1928]
    tunnel: w85 -> [w1927]
    tunnel: w84 -> [w1920]
    tunnel: w83 -> [w1923]
    tunnel: w82 -> [w1922]
    tunnel: w81 -> [w1935]
    tunnel: w80 -> [w1934]
    tunnel: w79 -> [w1933]
    tunnel: w78 -> [w1932]
    tunnel: w77 -> [w1931]
    tunnel: w76 -> [w1930]
    tunnel: w75 -> [w1929]
    tunnel: w74 -> [w1918]
    tunnel: w73 -> [w1925]
    tunnel: w72 -> [w1917]
    tunnel: w71 -> [w1916]
    tunnel: w70 -> [w1914]
    tunnel: w69 -> [w1915]
    tunnel: w68 -> [w1921]
    tunnel: w66 -> [w1919]
    tunnel: w64 -> [w1913]
    tunnel: w61 -> [w1912]
    tunnel: w36 -> [w1908]
    tunnel: w34 -> [w1907]
    tunnel: w32 -> [w1906]
    tunnel: w30 -> [w1905]
    tunnel: w28 -> [w1904]
    tunnel: w26 -> [w1903]
    tunnel: w24 -> [w1902]
    tunnel: w22 -> [w1901]
    tunnel: w20 -> [w1900]
    tunnel: w18 -> [w1899]
    tunnel: w15 -> [w1898]
    tunnel: w13 -> [w1897]
    tunnel: w9 -> [w1896]
    tunnel: w5 -> [w1895]
    tunnel: w89 -> [w2568]
    tunnel: w88 -> [w2567]
    tunnel: w87 -> [w2566]
    frame #0 {
      n597 = local read "single channel voltage array"() -> (w1669:dbl[])
      n598 = local read "samples to exclude"() -> (w1695:u32)
      n599 = local read "No. of Samples:"() -> (w1696:u32)
      n600 = local read "real time P_rad array"() -> (w1663:dbl[])
      n601 = local read "full P_rad [MW] HBC"() -> (w1668:dbl[])
      n602 = local read "full P_rad [MW] VBC"() -> (w1667:dbl[])
      n603 = Subtract(x=w1696, y=w1695) -> (x-y=w1665:u32)
      n604 = case "Correct timebase depending on if Trigger detected" shown="Default" w1697 {
        selector: w1697 -> [w1704 _]
        tunnel: [w1705 w1707] -> w1685
        tunnel: w1698 -> [w1703 _]
        frame Default {
          # "1 Trigger nur während OP"
          # "4294967295"
          # "Trigger deviation [ns]"
          # "Input Sample Frequency"
          n605 = Multiply(x=w1704, y=w1703) -> (x*y=w1702:i64)
          n606 = To Quad Integer(1:w1702) -> (0:w1705:i64)
        }
        frame 4294967295 {
          # "ms to ns conversion"
          # "4294967295\n=default if not Trigger"
          n607 = local read "DAQ wait time (should be = TWT"() -> (w1706:i32)
          n608 = Multiply(x=i64 1000000, y=w1706) -> (x*y=w1707:i64)
        }
      }
      n609 = To Long Integer(number=w1665) -> (32bit integer=w1664:i32)
      n610 = call "Array_Trans.vi"("RB01"=w1673, "Kappa 2"=w1674, "Single Channel Voltage"=w1669, "RB01 2"=w1672, "Tau 2"=w1670, "NSamples"=w1664, "Mean [mV]"=w1676, "Kappa"=w1675, "full P_rad VBC"=w1667, "full P_rad HBC"=w1668, "Tau"=w1671, "real time P_rad"=w1663) -> ("full P_rad VBC"=w1666:dbl[][], "Mean [mV]"=w1688:dbl[][], "Tau2"=w1691:dbl[][], 17:"RB01"=w1693:dbl[][], "real time P_rad"=w1662:dbl[][], "Tau"=w1694:dbl[][], "Kappa"=w1692:dbl[][], "full P_rad HBC"=w1678:dbl[][], "Kappa2"=w1689:dbl[][], 25:"RB01"=w1690:dbl[][], "Single Channel Voltage"=w1687:dbl[][])  [unwired: 5 in]
      n611 = local read "kbolott_and_volume"() -> (w1677:dbl[][])
    }
    frame #1 {
      n612 = control-ref of="DAQ Timer"() -> (w1740:refnum<vi>)
      n613 = call "W7X-Bolo-Timer.vi"("Wait-Time until Trigger\npublished on CODA\ntypically 10 s"="Wait-Time until Trigger; published on CODAC", "Digital in"=w1740) -> ()  [unwired: 10 in]
      n614 = local write "state"("Wait for published Shot Time" ("state")) -> ()
    }
    frame #2 {
      n615 = call <vilib>:"OpenHandle.vi"() -> ("client handle out"=w1764:T52, "error out"=w1768:errorcluster)  [unwired: 14 in]
      n616 = call <vilib>:"GET.vi"("client handle"=w1764, "url"="http://sv-coda-wsvc-3.ipp-hgw.mpg.de/last_trigger", "error in (no error)"=w1768) -> ("client handle out"=w1763:T52, "body"=w1766:string, "error out"=w1762:errorcluster)  [unwired: 9 in, 1 out]
      n617 = call <vilib>:"CloseHandle.vi"("client handle"=w1763, "error in (no error)"=w1762) -> ("error out"=w1761:errorcluster)  [unwired: 13 in]
      n618 = case shown="0" "Trigger Source" {
        tunnel: [w1793 w1795 "Set Manual Time [ns]" w1797] -> w1786
        tunnel: "Trigger No Choice from MDS+ Website\n0 for old 1 during OP" -> [_ w1794 _ _]
        frame 0 {
          n619 = call "Get UTC from NTP.vi"() -> ("UTC Time"=w1793:i64)  [unwired: 10 in, 1 out]
        }
        frame 1, Default {
          n620 = call "GetTriggerTime.vi"("TriggerIndex (1)"=w1794) -> ("TriggerTime [ns]"=w1795:i64)  [unwired: 9 in, 1 out]
        }
        frame 2 {
        }
        frame 3 {
          n621 = local read "start time"() -> (w1797:i64)
        }
      }
      "final trigger time" <- w1786
      n622 = Scan From String(input string=w1766, error in=w1761, default 1=i64 0 ("default (0 I32)")) -> (output 1=→"last trigger time by codac":i64)  [unwired: 2 in, 3 out]
      n623 = local write "state"("Reading Trigger Time" ("state")) -> ()
    }
    frame #3 {
      w1874 = i64 -1  # Time Array needs to be positive!
      w1816 = 10000 ("dimension size")
      # "DAQ start"
      # "10000"
      # "10000"
      # "offset the daq timing with\nthe excluded samples"
      # "time when DAQ started [ns]"
      # "TriggerT0"
      # "SampleRate in negative ns"
      # "Time array for Bolo Signal"
      # "Sample rate for Calibration Arrays\n should be hardwired to calirbation settings"
      # "Sample Rate in [ns]"
      # "NSample"
      # "Creating virtual Time Stamp\nfor Shot and for Calibration (Hardwired to 10000 samples)\nShot is depending on set sample rate"
      n624 = local read "samples to exclude"() -> (w1814:u32)
      n625 = local read "No. of Samples:"() -> (w1875:u32)
      n626 = local read "predicted time [ms] to finalize DAQ"() -> (w1840:dbl)
      n627 = local read "Measured Time for DAQ [ms]"() -> (w1841:u32)
      n628 = local read "single channel signal factor"() -> (w1837:dbl)
      n629 = local read "single channel number"() -> (w1839:i64)
      n630 = Initialize Array(w1807, w1816) -> (w1872:i64[])
      n631 = local read "SampleTime"() -> (w1833:sgl)
      n632 = local read "start time"() -> (w1838:i64)
      n633 = local read "Global DAC Range Setting"() -> (w1842:u8)
      n634 = To Quad Integer(1:w1814) -> (0:w1813:i64)
      n635 = local read "DAC and AD Settings"() -> (w1846:i32)
      n636 = local read "AD 7730 Bit Settings"() -> (w1847:i32)
      n637 = Multiply(x=w1813, y=w1803) -> (x*y=w1815:i64)
      n638 = Subtract(x=w1875, y=w1814) -> (x-y=w1853:u32)
      n639 = Multiply(x=w1815, y=i64 -1) -> (x*y=w1810:i64)
      n640 = Add(x=w1807, y=w1868) -> (x+y=w1811:i64)
      n641 = Divide(x=sgl 1.0, y=w1833) -> (x/y=w1831:sgl)
      n642 = Multiply(x=w1803, y=w1874) -> (x*y=w1809:i64)
      n643 = Add(x=w1810, y=w1811) -> (x+y=w1806:i64)
      "DAQ Start (epoch) [ns]" <- w1806
      n644 = To Quad Integer(1:w1806) -> (0:w1870:i64)
      n645 = Replace Array Subset(array=i64[] [1399090569999999999, -1] ("dimensions"), new element=w1870, index=0) -> (w1850:i64[])
      n646 = call "Parlog_creation.vi"("DAC Range Setting"=w1842, "DAC and AD Settings"=w1846, "AD 7730 Bit Settings"=w1847, "predicted time [ms] to finalize DAQ"=w1840, "Measured Time for DAQ [ms]"=w1841, "start time"=w1838, "single channel voltage factor"=w1837, "Single Channel Voltage Output AO"=tag "Dev1/ao0:1" ("Single Channel Output AO"), "single channel number"=w1839, "maximum voltage @ 10MW single channel"=10.0, "sample_rate"=w1831, "pulse_length"=w1833, "sample_period"=w1833) -> ("chanDescs_defaultInd"=w1835:T21, "chanDescs_ArrayOfArray"=w1834:T29, "cluster"=w1830:T27, "reduced cluster array"=w1829:T26, "reduced cluster"=w1828:T28, "chanDescsInd"=w1836:T21, "cluster array"=w1808:T25)
      n647 = local write "state"("Setting up time arrays and trigger" ("state")) -> ()
      n648 = Build Array(w1806) -> (w1849:i64[])
      n649 = Initialize Array(w1806, w1853) -> (w1871:i64[])
      n650 = disable-structure shown="Disabled" {
        disable-tunnel: w1836 -> [w1882 _]
        disable-tunnel: w1835 -> [w1881 _]
        disable-tunnel: w1834 -> [w1880 _]
        disable-tunnel: w1830 -> [w1879 _]
        disable-tunnel: w1829 -> [w1878 _]
        disable-tunnel: w1828 -> [w1877 _]
        disable-tunnel: w1808 -> [w1876 _]
        frame Disabled {
          "reduced cluster" <- w1877
          "chanDescsInd" <- w1882
          "reduced cluster array" <- w1878
          "chanDescs_defaultInd" <- w1881
          "chanDescs_ArrayClust" <- w1880
          "cluster" <- w1879
          "cluster array" <- w1876
        }
        frame Enabled {
        }
      }
      n651 = Subtract(x=w1806, y=w1807) -> (x-y=→"Downtime after T0 until DAQ [ns]":i64)
      n652 = for {
        N: w1853 -> [_]
        shift-right: [w1893] -> w1851
        shift-left: w1871 -> [w1894]
        shift-right: [w1890] -> _
        shift-left: w1806 -> [w1891]
        tunnel: w1809 -> [w1889]
        i -> [w1892]
        n653 = Add(x=w1891, y=w1889) -> (x+y=w1890:i64)
        n654 = Replace Array Subset(array=w1894, new element=w1891, index=w1892) -> (w1893:i64[])
      }
      n655 = for {
        N: w1816 -> [_]
        shift-right: [w1887] -> w1852
        shift-left: w1872 -> [w1888]
        shift-right: [w1884] -> _
        shift-left: w1806 -> [w1885]
        tunnel: w1809 -> [w1883]
        i -> [w1886]
        n656 = Add(x=w1885, y=w1883) -> (x+y=w1884:i64)
        n657 = Replace Array Subset(array=w1888, new element=w1885, index=w1886) -> (w1887:i64[])
      }
    }
    frame #4 {
      # "BoloAdjusted"
      # "real time P_rad"
      # "full P_rad VBC"
      # "FullP_radVBC"
      # "A2"
      # "A"
      # "B"
      # "C"
      # "D"
      # "FullP_radHBCM"
      # "singleChannelVoltage"
      # "TauRef"
      # "TauM"
      # "RRes"
      # "MRes"
      # "KappaRef"
      # "KappaM"
      # "Mean [mV]"
      # "SampleFInt"
      # "Samplefrequency"
      # "samplePeriod"
      # "DimensionA: 10000 points at sampel time in nanoseconds and epoch time, for calibration etc.\n\nDimensionA2: Number of Samples\n\nDimensionB: [No. of Samples] points at sample time (epoch and nanoseconds) for measurement etc.\n\nDimensionC: Start time (epoch and nanoseconds) and -1 for until next entry\n\nDimensionD: Start time only"
      # "BoloPowerRaw"
      # "BoloSignal"
      # "BoloCalibRefFoilFit"
      # "kbolott&volume"
      # "HBCmPrad"
      # "SingleChannelFeedback"
      # "BoloCalibMeasFoilCurrent"
      # "BoloCalibRefFoilCurrent"
      # "BoloCalibMeasFoilFit"
      # "Offset"
      # "RKappa"
      # "RRes"
      # "RTau"
      # "MKappa"
      # "MRes"
      # "MTau"
      n658 = local read "SampleTime"() -> (w1909:sgl)
      n659 = Reciprocal(x=w1909) -> (1/x=w1910:sgl)
      n660 = To Unsigned Word Integer(number=w1910) -> (unsigned 16bit integer=w1911:u16)
      n661 = disable-structure shown="Enabled" {
        disable-tunnel: w1935 -> [w1949 _]
        disable-tunnel: w1934 -> [w1951 _]
        disable-tunnel: w1933 -> [w1953 _]
        disable-tunnel: w1932 -> [w1954 _]
        disable-tunnel: w1931 -> [w1952 _]
        disable-tunnel: w1930 -> [w1950 _]
        disable-tunnel: w1929 -> [w1955 _]
        disable-tunnel: w1928 -> [w1965 _]
        disable-tunnel: w1927 -> [w1959 _]
        disable-tunnel: w1923 -> [w1967 _]
        disable-tunnel: w1922 -> [w1964 _]
        disable-tunnel: w1921 -> [w1957 _]
        disable-tunnel: w1920 -> [w1960 _]
        disable-tunnel: w1919 -> [w1963 _]
        disable-tunnel: w1918 -> [w1944 _]
        disable-tunnel: w1917 -> [w1942 _]
        disable-tunnel: w1916 -> [w1947 _]
        disable-tunnel: w1915 -> [w1938 _]
        disable-tunnel: w1914 -> [w1941 _]
        disable-tunnel: w1913 -> [w1948 _]
        disable-tunnel: w1912 -> [_ _]
        disable-tunnel: w1911 -> [w1939 _]
        disable-tunnel: w1910 -> [_ _]
        disable-tunnel: w1909 -> [w1940 _]
        disable-tunnel: w1908 -> [w1971 _]
        disable-tunnel: w1907 -> [w1970 _]
        disable-tunnel: w1906 -> [w1968 _]
        disable-tunnel: w1905 -> [w1961 _]
        disable-tunnel: w1904 -> [w1966 _]
        disable-tunnel: w1903 -> [w1943 _]
        disable-tunnel: w1902 -> [w1969 _]
        disable-tunnel: w1901 -> [w1962 _]
        disable-tunnel: w1900 -> [w1958 _]
        disable-tunnel: w1899 -> [w1937 _]
        disable-tunnel: w1898 -> [w1956 _]
        disable-tunnel: w1897 -> [w1946 _]
        disable-tunnel: w1896 -> [w1945 _]
        disable-tunnel: w1895 -> [w1936 _]
        frame Enabled {
          n662 = disable-structure shown="Enabled" {
            disable-tunnel: w1937 -> [w2091 w2122]
            disable-tunnel: w1957 -> [_ w2118]
            disable-tunnel: w1938 -> [w2092 w2116]
            disable-tunnel: w1947 -> [w2093 _]
            frame Enabled {
              w2097 = "Number"  # Unit
              w2106 = "Integer"  # datatype
              w2100 = "ChannelSelection"  # label
              n663 = local read "final channel selection"() -> (w2105:i64[][])
              n664 = Array Size(array=w2105) -> (size(s)=w2104:i32[])
              n665 = Index Array(array=w2104, index=0) -> (element=w2099:i32)
              n666 = Index Array(array=w2104, index=1) -> (element=w2101:i32)
              n667 = call "W7X2DJSON.vi"("values"=w2105, "label"=w2100, "dimensionSize"=w2099, "dimensions"=w2093, "dimensionCount"=w2101, "sampleCount"=w2099, "datatype"=w2106) -> ("JSON string"=w2098:string)  [unwired: 4 in]
              n668 = disable-structure shown="Disabled" {
                disable-tunnel: w2098 -> [w2107 _]
                frame Disabled {
                  "ChannelSelectionJSON" <- w2107
                }
                frame Enabled {
                }
              }
              n669 = call "W7X2DPut.vi"("SigLabel"=w2100, "Unit"=w2097, "SigJSONbuffer"=w2098, "values"=w2091, "dimensions"=w2092) -> ("headers parms"=→"ChannelSelection headers parms":string, "headers"=→"ChannelSelection headers":string, "body"=→"ChannelSelection body":string, "body Parlog"=→"ChannelSelection body Parlog":string, "file path written"=→"ChannelSelection path":string, "Parlog error out"=w2095:errorcluster)  [unwired: 5 in]
              "ChannelSelection ErrorOut" <- w2095
              n670 = Unbundle(w2095) -> ("status"=→"ChannelSelection status":bool)  [unwired: 2 out]
            }
            frame Disabled {
              w2124 = "Number"  # Unit
              w2125 = "Integer"  # datatype
              w2123 = "ChannelSelection"  # label
              n671 = local read "final channel selection"() -> (w2121:i64[][])
              n672 = Array Size(array=w2121) -> (size(s)=w2126:i32[])
              n673 = Index Array(array=w2126, index=0) -> (element=w2117:i32)
              n674 = Index Array(array=w2121, index (col)=0 ("disabled index (col)")) -> (element=w2119:i64[])  [unwired: 1 in]
              n675 = call "W7X1DJSON.vi"("values"=w2119, "label"=w2123, "Unit"=w2124, "dimensions"=w2118, "dimensionCount"=w2117, "datatype"=w2125) -> ("JSON string"=w2112:string)  [unwired: 5 in]
              n676 = disable-structure shown="Disabled" {
                disable-tunnel: w2112 -> [w2128 _]
                frame Disabled {
                  n677 = local write "ChannelSelectionJSON"(w2128) -> ()
                }
                frame Enabled {
                }
              }
              n678 = call "W7X1DPut.vi"("dimensions"=w2116, "Unit"=w2124, "values"=w2122, "SigJSONbuffer"=w2112, "SigLabel"=w2123) -> ("Parlog error out"=w2114:errorcluster, "file path written"=w2115:string, "headers parms"=w2109:string, "body Parlog"=w2110:string, "body"=w2111:string, "headers"=w2108:string)  [unwired: 1 in]
              n679 = local write "ChannelSelection ErrorOut"(w2114) -> ()
              n680 = local write "ChannelSelection path"(w2115) -> ()
              n681 = Unbundle(w2114) -> ("status"=w2113:bool)  [unwired: 2 out]
              n682 = local write "ChannelSelection status"(w2113) -> ()
            }
          }
          n683 = disable-structure shown="Enabled" {
            disable-tunnel: w1957 -> [w2501 w2526]
            disable-tunnel: w1970 -> [_ w2525]
            disable-tunnel: w1938 -> [w2500 w2524]
            disable-tunnel: w1937 -> [w2502 w2518]
            disable-tunnel: w1953 -> [w2503 _]
            frame Enabled {
              w2510 = 1 ("sampleCount")
              w2512 = "Float"  # datatype
              w2507 = "W"  # Unit
              w2509 = "MKappa"  # label
              n684 = call "W7X2DJSON.vi"("values"=w2503, "label"=w2509, "dimensionSize"=w2510, "dimensions"=w2501, "dimensionCount"=128, "sampleCount"=w2510, "datatype"=w2512) -> ("JSON string"=w2508:string)  [unwired: 4 in]
              n685 = disable-structure shown="Disabled" {
                disable-tunnel: w2508 -> [w2513 _]
                frame Disabled {
                  # "DimensionC"
                  "MKappaJSON" <- w2513
                }
                frame Enabled {
                }
              }
              n686 = call "W7X1DPut.vi"("dimensions"=w2500, "Unit"=w2507, "values"=w2502, "SigJSONbuffer"=w2508, "SigLabel"=w2509) -> ("Parlog error out"=w2506:errorcluster, "file path written"=→"MKappa path":string, "headers parms"=w2497:string, "body Parlog"=w2498:string, "body"=w2499:string, "headers"=w2496:string)  [unwired: 1 in]
              "MKappaErrorOut" <- w2506
              n687 = Unbundle(w2506) -> ("status"=→"MKappa Status":bool)  [unwired: 2 out]
              n688 = local write "headers 2"(w2496) -> ()
              n689 = local write "headers parms 2"(w2497) -> ()
              n690 = local write "body Parlog 2"(w2498) -> ()
              n691 = local write "body 2"(w2499) -> ()
            }
            frame Disabled {
              w2527 = "W" ("Unit")
              w2528 = "Float"  # datatype
              w2529 = "MKappa"  # label
              n692 = call "W7X1DJSON.vi"("values"=w2525, "label"=w2529, "Unit"=w2527, "dimensions"=w2526, "dimensionCount"=128, "datatype"=w2528) -> ("JSON string"=w2522:string)  [unwired: 5 in]
              n693 = disable-structure shown="Disabled" {
                disable-tunnel: w2522 -> [w2530 _]
                frame Disabled {
                  n694 = local write "MKappaJSON"(w2530) -> ()
                }
                frame Enabled {
                }
              }
              n695 = call "W7X1DPut.vi"("dimensions"=w2524, "Unit"=w2527, "values"=w2518, "SigJSONbuffer"=w2522, "SigLabel"=w2529) -> ("Parlog error out"=w2521:errorcluster, "file path written"=w2519:string, "headers parms"=→"headers parms 2":string, "body Parlog"=→"body Parlog 2":string, "body"=→"body 2":string, "headers"=→"headers 2":string)  [unwired: 1 in]
              n696 = local write "MKappaErrorOut"(w2521) -> ()
              n697 = local write "MKappa path"(w2519) -> ()
              n698 = Unbundle(w2521) -> ("status"=w2520:bool)  [unwired: 2 out]
              n699 = local write "MKappa Status"(w2520) -> ()
            }
          }
          n700 = disable-structure shown="Enabled" {
            disable-tunnel: w1957 -> [w2398 w2423]
            disable-tunnel: w1938 -> [w2396 w2422]
            disable-tunnel: w1968 -> [_ w2419]
            disable-tunnel: w1937 -> [w2397 w2414]
            disable-tunnel: w1950 -> [w2399 _]
            frame Enabled {
              w2405 = 1 ("sampleCount")
              w2408 = "Float"  # datatype
              w2406 = "W"  # Unit
              w2403 = "RKappa"  # label
              n701 = call "W7X2DJSON.vi"("values"=w2399, "label"=w2403, "dimensionSize"=w2405, "dimensions"=w2398, "dimensionCount"=128, "sampleCount"=w2405, "datatype"=w2408) -> ("JSON string"=w2404:string)  [unwired: 4 in]
              n702 = disable-structure shown="Disabled" {
                disable-tunnel: w2404 -> [w2409 _]
                frame Disabled {
                  # "DimensionC"
                  "RKappaJSON" <- w2409
                }
                frame Enabled {
                }
              }
              n703 = call "W7X1DPut.vi"("dimensions"=w2396, "Unit"=w2406, "values"=w2397, "SigJSONbuffer"=w2404, "SigLabel"=w2403) -> ("Parlog error out"=w2402:errorcluster, "file path written"=→"RKappa path":string, "headers parms"=w2393:string, "body Parlog"=w2394:string, "body"=w2395:string, "headers"=w2392:string)  [unwired: 1 in]
              "RKappaErrorOut" <- w2402
              n704 = Unbundle(w2402) -> ("status"=→"RKappa Status":bool)  [unwired: 2 out]
              n705 = local write "headers 3"(w2392) -> ()
              n706 = local write "headers parms 3"(w2393) -> ()
              n707 = local write "body Parlog 3"(w2394) -> ()
              n708 = local write "body 3"(w2395) -> ()
            }
            frame Disabled {
              w2420 = "W" ("Unit")
              w2425 = "Float"  # datatype
              w2421 = "RKappa"  # label
              n709 = call "W7X1DJSON.vi"("values"=w2419, "label"=w2421, "Unit"=w2420, "dimensions"=w2423, "dimensionCount"=128, "datatype"=w2425) -> ("JSON string"=w2418:string)  [unwired: 5 in]
              n710 = disable-structure shown="Disabled" {
                disable-tunnel: w2418 -> [w2426 _]
                frame Disabled {
                  n711 = local write "RKappaJSON"(w2426) -> ()
                }
                frame Enabled {
                }
              }
              n712 = call "W7X1DPut.vi"("dimensions"=w2422, "Unit"=w2420, "values"=w2414, "SigJSONbuffer"=w2418, "SigLabel"=w2421) -> ("Parlog error out"=w2417:errorcluster, "file path written"=w2415:string, "headers parms"=→"headers parms 3":string, "body Parlog"=→"body Parlog 3":string, "body"=→"body 3":string, "headers"=→"headers 3":string)  [unwired: 1 in]
              n713 = local write "RKappaErrorOut"(w2417) -> ()
              n714 = local write "RKappa path"(w2415) -> ()
              n715 = Unbundle(w2417) -> ("status"=w2416:bool)  [unwired: 2 out]
              n716 = local write "RKappa Status"(w2416) -> ()
            }
          }
          n717 = disable-structure shown="Enabled" {
            disable-tunnel: w1971 -> [_ w2561]
            disable-tunnel: w1938 -> [w2535 w2560]
            disable-tunnel: w1957 -> [w2538 w2559]
            disable-tunnel: w1937 -> [w2536 w2556]
            disable-tunnel: w1955 -> [w2537 _]
            frame Enabled {
              w2543 = 1 ("sampleCount")
              w2547 = "Float"  # datatype
              w2544 = "mV"  # Unit
              w2540 = "Offset"  # label
              n718 = call "W7X2DJSON.vi"("values"=w2537, "label"=w2540, "dimensionSize"=w2543, "dimensions"=w2538, "dimensionCount"=128, "sampleCount"=w2543, "datatype"=w2547) -> ("JSON string"=w2545:string)  [unwired: 4 in]
              n719 = disable-structure shown="Disabled" {
                disable-tunnel: w2545 -> [w2548 _]
                frame Disabled {
                  # "DimensionC"
                  "OffsetJSON" <- w2548
                }
                frame Enabled {
                }
              }
              n720 = call "W7X1DPut.vi"("dimensions"=w2535, "Unit"=w2544, "values"=w2536, "SigJSONbuffer"=w2545, "SigLabel"=w2540) -> ("Parlog error out"=w2542:errorcluster, "file path written"=→"Offset path":string, "headers parms"=w2531:string, "body Parlog"=w2532:string, "body"=w2534:string, "headers"=w2533:string)  [unwired: 1 in]
              "OffsetErrorOut" <- w2542
              n721 = Unbundle(w2542) -> ("status"=→"Offset Status":bool)  [unwired: 2 out]
              n722 = local write "body 15"(w2534) -> ()
              n723 = local write "body Parlog 15"(w2532) -> ()
              n724 = local write "headers parms 15"(w2531) -> ()
              n725 = local write "headers 15"(w2533) -> ()
            }
            frame Disabled {
              w2564 = "Offset" ("label")
              w2557 = "mV" ("Unit")
              n726 = call "W7X1DJSON.vi"("values"=w2561, "label"=w2564, "Unit"=w2557, "dimensions"=w2559, "dimensionCount"=128, "datatype"="Float") -> ("JSON string"=w2558:string)  [unwired: 5 in]
              n727 = disable-structure shown="Disabled" {
                disable-tunnel: w2558 -> [w2565 _]
                frame Disabled {
                  n728 = local write "OffsetJSON"(w2565) -> ()
                }
                frame Enabled {
                }
              }
              n729 = call "W7X1DPut.vi"("dimensions"=w2560, "Unit"=w2557, "values"=w2556, "SigJSONbuffer"=w2558, "SigLabel"=w2564) -> ("Parlog error out"=w2555:errorcluster, "file path written"=w2553:string, "headers parms"=→"headers parms 15":string, "body Parlog"=→"body Parlog 15":string, "body"=→"body 15":string, "headers"=→"headers 15":string)  [unwired: 1 in]
              n730 = local write "OffsetErrorOut"(w2555) -> ()
              n731 = local write "Offset path"(w2553) -> ()
              n732 = Unbundle(w2555) -> ("status"=w2554:bool)  [unwired: 2 out]
              n733 = local write "Offset Status"(w2554) -> ()
            }
          }
          n734 = disable-structure shown="Enabled" {
            disable-tunnel: w1942 -> [w2139 _]
            disable-tunnel: w1963 -> [w2138 _]
            disable-tunnel: w1941 -> [w2129 _]
            disable-tunnel: w1937 -> [w2137 _]
            disable-tunnel: w1939 -> [w2136 _]
            disable-tunnel: w1940 -> [w2135 _]
            disable-tunnel: w1938 -> [w2130 _]
            frame Enabled {
              w2147 = "W"  # Unit
              w2144 = "Float"  # datatype
              w2146 = "BoloPowerRaw"  # label
              n735 = call "W7X2DJSON.vi"("values"=w2138, "label"=w2146, "dimensionSize"=w2139, "dimensions"=w2129, "dimensionCount"=128, "sampleCount"=w2139, "datatype"=w2144) -> ("JSON string"=w2145:string)  [unwired: 4 in]
              n736 = disable-structure shown="Disabled" {
                disable-tunnel: w2145 -> [w2148 _]
                frame Disabled {
                  # "DimensionB"
                  "PowerRawJSON" <- w2148
                }
                frame Enabled {
                }
              }
              n737 = call "W7X2DPut.vi"("SigLabel"=w2146, "Unit"=w2147, "SigJSONbuffer"=w2145, "values"=w2137, "dimensions"=w2130, "sample rate"=w2136, "sample period"=w2135, "pulse_length"=w2135) -> ("headers parms"=→"headers parms 10":string, "headers"=→"headers 10":string, "body"=→"body 10":string, "body Parlog"=→"body Parlog 10":string, "file path written"=→"BoloPower path":string, "Parlog error out"=w2142:errorcluster)  [unwired: 2 in]
              "BoloPowerRawErrorOut" <- w2142
              n738 = Unbundle(w2142) -> ("status"=→"BoloPower status":bool)  [unwired: 2 out]
            }
            frame Disabled {
            }
          }
          n739 = disable-structure shown="Enabled" {
            disable-tunnel: w1938 -> [w2060 _]
            frame Disabled {
              # "DimensionC"
              n740 = call "chanDescQSB.vi"("dimensions"=w2060, "values"=T29 [{"chanDescs"=[{"name"="E_Chan_1", "active"=1}, {"name"="E_Chan_2", "active"=1}, {"name"="E_Chan_3", "active"=1}, {"name"="E_Chan_4", "active"=1}, {"name"="E_Chan_5", "active"=1}, {"name"="E_Chan_6", "active"=1}, {"name"="E_Chan_7", "active"=1}, {"name"="E_Chan_8", "active"=1}, {"name"="E_Chan_9", "active"=1}, {"name"="E_Chan_10", "active"=1}, {"name"="E_Chan_11", "active"=1}, {"name"="E_Chan_12", "active"=1}, {"name"="E_Chan_13", "active"=1}, {"name"="E_Chan_14", "active"=1}, {"name"="E_Chan_15", "active"=1}, {"name"="E_Chan_16", "active"=1}, {"name"="E_Chan_17", "active"=1}, {"name"="E_Chan_18", "active"=1}, {"name"="E_Chan_19", "active"=1}, {"name"="E_Chan_20", "active"=1}, {"name"="E_Chan_21", "active"=1}, {"name"="E_Chan_22", "active"=1}, {"name"="E_Chan_23", "active"=1}, {"name"="E_Chan_24", "active"=1}, {"name"="E_Chan_25", "active"=1}, {"name"="E_Chan_26", "active"=1}, {"name"="E_Chan_27", "active"=1}, {"name"="E_Chan_28", "active"=1}, {"name"="E_Chan_29", "active"=1}, {"name"="E_Chan_30", "active"=1}, {"name"="E_Chan_31", "active"=1}, {"name"="E_Chan_32", "active"=1}, {"name"="E_Chan_33", "active"=1}, {"name"="E_Chan_34", "active"=1}, {"name"="E_Chan_35", "active"=1}, {"name"="E_Chan_36", "active"=1}, {"name"="E_Chan_37", "active"=1}, {"name"="E_Chan_38", "active"=1}, {"name"="E_Chan_39", "active"=1}, {"name"="E_Chan_40", "active"=1}, {"name"="E_Chan_41", "active"=1}, {"name"="E_Chan_42", "active"=1}, {"name"="E_Chan_43", "active"=1}, {"name"="E_Chan_44", "active"=1}, {"name"="E_Chan_45", "active"=1}, {"name"="E_Chan_46", "active"=1}, {"name"="E_Chan_47", "active"=1}, {"name"="E_Chan_48", "active"=1}, {"name"="E_Chan_49", "active"=1}, {"name"="E_Chan_50", "active"=1}, {"name"="E_Chan_51", "active"=1}, {"name"="E_Chan_52", "active"=1}, {"name"="E_Chan_53", "active"=1}, {"name"="E_Chan_54", "active"=1}, {"name"="E_Chan_55", "active"=1}, {"name"="E_Chan_56", "active"=1}, {"name"="E_Chan_57", "active"=1}, {"name"="E_Chan_58", "active"=1}, {"name"="E_Chan_59", "active"=1}, {"name"="E_Chan_60", "active"=1}, {"name"="E_Chan_61", "active"=1}, {"name"="E_Chan_62", "active"=1}, {"name"="E_Chan_63", "active"=1}, {"name"="E_Chan_64", "active"=1}, {"name"="E_Chan_65", "active"=1}, {"name"="E_Chan_66", "active"=1}, {"name"="E_Chan_67", "active"=1}, {"name"="E_Chan_68", "active"=1}, {"name"="E_Chan_69", "active"=1}, {"name"="E_Chan_70", "active"=1}, {"name"="E_Chan_71", "active"=1}, {"name"="E_Chan_72", "active"=1}, {"name"="E_Chan_73", "active"=1}, {"name"="E_Chan_74", "active"=1}, {"name"="E_Chan_75", "active"=1}, {"name"="E_Chan_76", "active"=1}, {"name"="E_Chan_77", "active"=1}, {"name"="E_Chan_78", "active"=1}, {"name"="E_Chan_79", "active"=1}, {"name"="E_Chan_80", "active"=1}, {"name"="E_Chan_81", "active"=1}, {"name"="E_Chan_82", "active"=1}, {"name"="E_Chan_83", "active"=1}, {"name"="E_Chan_84", "active"=1}, {"name"="E_Chan_85", "active"=1}, {"name"="E_Chan_86", "active"=1}, {"name"="E_Chan_87", "active"=1}, {"name"="E_Chan_88", "active"=1}, {"name"="E_Chan_89", "active"=1}, {"name"="E_Chan_90", "active"=1}, {"name"="E_Chan_91", "active"=1}, {"name"="E_Chan_92", "active"=1}, {"name"="E_Chan_93", "active"=1}, {"name"="E_Chan_94", "active"=1}, {"name"="E_Chan_95", "active"=1}, {"name"="E_Chan_96", "active"=1}, {"name"="E_Chan_97", "active"=1}, {"name"="E_Chan_98", "active"=1}, {"name"="E_Chan_99", "active"=1}, {"name"="E_Chan_100", "active"=1}, {"name"="E_Chan_101", "active"=1}, {"name"="E_Chan_102", "active"=1}, {"name"="E_Chan_103", "active"=1}, {"name"="E_Chan_104", "active"=1}, {"name"="E_Chan_105", "active"=1}, {"name"="E_Chan_106", "active"=1}, {"name"="E_Chan_107", "active"=1}, {"name"="E_Chan_108", "active"=1}, {"name"="E_Chan_109", "active"=1}, {"name"="E_Chan_110", "active"=1}, {"name"="E_Chan_111", "active"=1}, {"name"="E_Chan_112", "active"=1}, {"name"="E_Chan_113", "active"=1}, {"name"="E_Chan_114", "active"=1}, {"name"="E_Chan_115", "active"=1}, {"name"="E_Chan_116", "active"=1}, {"name"="E_Chan_117", "active"=1}, {"name"="E_Chan_118", "active"=1}, {"name"="E_Chan_119", "active"=1}, {"name"="E_Chan_120", "active"=1}, {"name"="E_Chan_121", "active"=1}, {"name"="E_Chan_122", "active"=1}, {"name"="E_Chan_123", "active"=1}, {"name"="E_Chan_124", "active"=1}, {"name"="E_Chan_125", "active"=1}, {"name"="E_Chan_126", "active"=1}, {"name"="E_Chan_127", "active"=1}, {"name"="E_Chan_128", "active"=1}]}], "label"="parms") -> ()  [unwired: 1 out]
            }
            frame Enabled {
            }
          }
          n741 = disable-structure shown="Enabled" {
            disable-tunnel: w1965 -> [w2232 _]
            disable-tunnel: w1938 -> [w2231 _]
            disable-tunnel: w1947 -> [w2230 _]
            disable-tunnel: w1937 -> [w2229 _]
            disable-tunnel: w1939 -> [w2228 _]
            disable-tunnel: w1940 -> [w2227 _]
            frame Enabled {
              w2233 = 10000 ("sampleCount")
              w2241 = "Float"  # datatype
              w2238 = "A"  # Unit
              w2239 = "BoloCalibRefFoilFit"  # label
              n742 = call "W7X2DJSON.vi"("values"=w2232, "label"=w2239, "dimensionSize"=w2233, "dimensions"=w2230, "dimensionCount"=128, "sampleCount"=w2233, "datatype"=w2241) -> ("JSON string"=w2237:string)  [unwired: 4 in]
              n743 = disable-structure shown="Disabled" {
                disable-tunnel: w2237 -> [w2242 _]
                frame Disabled {
                  "CalibRefFoilFitJSON" <- w2242
                }
                frame Enabled {
                }
              }
              n744 = call "W7X2DPut.vi"("SigLabel"=w2239, "Unit"=w2238, "SigJSONbuffer"=w2237, "values"=w2229, "dimensions"=w2231, "sample rate"=w2228, "sample period"=w2227, "pulse_length"=w2227) -> ("headers parms"=→"headers parms 11":string, "headers"=→"headers 11":string, "body"=→"body 11":string, "body Parlog"=→"body Parlog 11":string, "file path written"=→"CalibRefFoilFit path":string, "Parlog error out"=w2235:errorcluster)  [unwired: 2 in]
              "BoloCalibRefFoilFitErrorOut" <- w2235
              n745 = Unbundle(w2235) -> ("status"=→"BoloCalibRefFoilFit Satus":bool)  [unwired: 2 out]
            }
            frame Disabled {
            }
          }
          n746 = disable-structure shown="Enabled" {
            disable-tunnel: w1957 -> [w2468 w2492]
            disable-tunnel: w1969 -> [_ w2491]
            disable-tunnel: w1938 -> [w2466 w2490]
            disable-tunnel: w1937 -> [w2467 w2484]
            disable-tunnel: w1954 -> [w2469 _]
            frame Enabled {
              w2477 = 1 ("sampleCount")
              w2478 = "Float"  # datatype
              w2474 = "s"  # Unit
              w2476 = "RTau"  # label
              n747 = call "W7X2DJSON.vi"("values"=w2469, "label"=w2476, "dimensionSize"=w2477, "dimensions"=w2468, "dimensionCount"=128, "sampleCount"=w2477, "datatype"=w2478) -> ("JSON string"=w2475:string)  [unwired: 4 in]
              n748 = disable-structure shown="Disabled" {
                disable-tunnel: w2475 -> [w2479 _]
                frame Disabled {
                  # "DimensionC"
                  "RTauJSON" <- w2479
                }
                frame Enabled {
                }
              }
              n749 = call "W7X1DPut.vi"("dimensions"=w2466, "Unit"=w2474, "values"=w2467, "SigJSONbuffer"=w2475, "SigLabel"=w2476) -> ("Parlog error out"=w2472:errorcluster, "file path written"=→"RTau Path":string, "headers parms"=w2463:string, "body Parlog"=w2464:string, "body"=w2465:string, "headers"=w2462:string)  [unwired: 1 in]
              "RTauErrorOut" <- w2472
              n750 = Unbundle(w2472) -> ("status"=→"RTau Status":bool)  [unwired: 2 out]
              n751 = local write "headers parms 4"(w2463) -> ()
              n752 = local write "headers 4"(w2462) -> ()
              n753 = local write "body 4"(w2465) -> ()
              n754 = local write "body Parlog 4"(w2464) -> ()
            }
            frame Disabled {
              w2493 = "s" ("Unit")
              w2494 = "Float"  # datatype
              w2495 = "RTau"  # label
              n755 = call "W7X1DJSON.vi"("values"=w2491, "label"=w2495, "Unit"=w2493, "dimensions"=w2492, "dimensionCount"=128, "datatype"=w2494) -> ("JSON string"=w2489:string)  [unwired: 5 in]
              n756 = disable-structure shown="Disabled" {
                disable-tunnel: w2489 -> [_ _]
                frame Disabled {
                  n757 = local read "RTauJSON"() -> ()  [unwired: 1 in]
                }
                frame Enabled {
                }
              }
              n758 = call "W7X1DPut.vi"("dimensions"=w2490, "Unit"=w2493, "values"=w2484, "SigJSONbuffer"=w2489) -> ("Parlog error out"=w2487:errorcluster, "file path written"=w2485:string, "headers parms"=→"headers parms 4":string, "body Parlog"=→"body Parlog 4":string, "body"=→"body 4":string, "headers"=→"headers 4":string)  [unwired: 2 in]
              n759 = local write "RTauErrorOut"(w2487) -> ()
              n760 = local write "RTau Path"(w2485) -> ()
              n761 = Unbundle(w2487) -> ("status"=w2486:bool)  [unwired: 2 out]
              n762 = local write "RTau Status"(w2486) -> ()
            }
          }
          n763 = disable-structure shown="Enabled" {
            disable-tunnel: w1957 -> [w2433 w2456]
            disable-tunnel: w1937 -> [w2432 w2455]
            disable-tunnel: w1966 -> [_ w2450]
            disable-tunnel: w1938 -> [w2431 w2449]
            disable-tunnel: w1952 -> [w2434 _]
            frame Enabled {
              w2441 = 1 ("sampleCount")
              w2443 = "Float"  # datatype
              w2438 = "Ohms"  # Unit
              w2440 = "RRes"  # label
              n764 = call "W7X2DJSON.vi"("values"=w2434, "label"=w2440, "dimensionSize"=w2441, "dimensions"=w2433, "dimensionCount"=128, "sampleCount"=w2441, "datatype"=w2443) -> ("JSON string"=w2439:string)  [unwired: 4 in]
              n765 = disable-structure shown="Disabled" {
                disable-tunnel: w2439 -> [w2444 _]
                frame Disabled {
                  "RResJSON" <- w2444
                }
                frame Enabled {
                }
              }
              n766 = call "W7X1DPut.vi"("dimensions"=w2431, "Unit"=w2438, "values"=w2432, "SigJSONbuffer"=w2439, "SigLabel"=w2440) -> ("Parlog error out"=w2437:errorcluster, "file path written"=→"RRes path":string, "headers parms"=w2428:string, "body Parlog"=w2429:string, "body"=w2430:string, "headers"=w2427:string)  [unwired: 1 in]
              "RResErrorOut" <- w2437
              n767 = Unbundle(w2437) -> ("status"=→"RRes Status":bool)  [unwired: 2 out]
              n768 = local write "headers parms 5"(w2428) -> ()
              n769 = local write "headers 5"(w2427) -> ()
              n770 = local write "body Parlog 5"(w2429) -> ()
              n771 = local write "body 5"(w2430) -> ()
            }
            frame Disabled {
              w2459 = "Float"  # datatype
              w2458 = "RRes"  # label
              w2460 = "Ohms" ("Unit")
              n772 = call "W7X1DJSON.vi"("values"=w2450, "label"=w2458, "Unit"=w2460, "dimensions"=w2456, "dimensionCount"=128, "datatype"=w2459) -> ("JSON string"=w2451:string)  [unwired: 5 in]
              n773 = disable-structure shown="Disabled" {
                disable-tunnel: w2451 -> [w2461 _]
                frame Disabled {
                  n774 = local write "RResJSON"(w2461) -> ()
                }
                frame Enabled {
                }
              }
              n775 = call "W7X1DPut.vi"("dimensions"=w2449, "Unit"=w2460, "values"=w2455, "SigJSONbuffer"=w2451, "SigLabel"=w2458) -> ("Parlog error out"=w2454:errorcluster, "file path written"=w2452:string, "headers parms"=→"headers parms 5":string, "body Parlog"=→"body Parlog 5":string, "body"=→"body 5":string, "headers"=→"headers 5":string)  [unwired: 1 in]
              n776 = local write "RResErrorOut"(w2454) -> ()
              n777 = local write "RRes path"(w2452) -> ()
              n778 = Unbundle(w2454) -> ("status"=w2453:bool)  [unwired: 2 out]
              n779 = local write "RRes Status"(w2453) -> ()
            }
          }
          n780 = disable-structure shown="Enabled" {
            disable-tunnel: w1947 -> [w2380 _]
            disable-tunnel: w1967 -> [w2381 _]
            disable-tunnel: w1938 -> [w2379 _]
            disable-tunnel: w1937 -> [w2378 _]
            disable-tunnel: w1939 -> [w2377 _]
            disable-tunnel: w1940 -> [w2376 _]
            frame Enabled {
              w2385 = "A"  # Unit
              w2388 = 10000 ("sampleCount")
              w2390 = "Float"  # datatype
              w2387 = "BoloCalibMeasFoilFit"  # label
              n781 = call "W7X2DJSON.vi"("values"=w2381, "label"=w2387, "dimensionSize"=w2388, "dimensions"=w2380, "dimensionCount"=128, "sampleCount"=w2388, "datatype"=w2390) -> ("JSON string"=w2386:string)  [unwired: 4 in]
              n782 = disable-structure shown="Disabled" {
                disable-tunnel: w2386 -> [w2391 _]
                frame Disabled {
                  # "DimensionC"
                  "CalibMeasFoilFit" <- w2391
                }
                frame Enabled {
                }
              }
              n783 = call "W7X2DPut.vi"("SigLabel"=w2387, "Unit"=w2385, "SigJSONbuffer"=w2386, "values"=w2378, "dimensions"=w2379, "sample rate"=w2377, "sample period"=w2376, "pulse_length"=w2376) -> ("headers parms"=→"headers parms":string, "headers"=→"headers":string, "body"=→"body":string, "body Parlog"=→"body Parlog":string, "file path written"=→"CalibMeasFoilFit path":string, "Parlog error out"=w2383:errorcluster)  [unwired: 2 in]
              "CalibMeasFoilFit 2" <- w2383
              n784 = Unbundle(w2383) -> ("status"=→"CalibMeasFoilFit status":bool)  [unwired: 2 out]
            }
            frame Disabled {
            }
          }
          n785 = disable-structure shown="Enabled" {
            disable-tunnel: w1937 -> [w2156 w2181]
            disable-tunnel: w1957 -> [_ _]
            disable-tunnel: w1942 -> [w2158 w2180]
            disable-tunnel: w1962 -> [_ w2179]
            disable-tunnel: w1941 -> [w2153 w2170]
            disable-tunnel: w1938 -> [w2159 w2169]
            disable-tunnel: w1944 -> [w2157 _]
            disable-tunnel: w1940 -> [w2155 _]
            disable-tunnel: w1939 -> [w2154 _]
            frame Enabled {
              w2167 = "V"  # Unit
              w2163 = "Float"  # datatype
              w2166 = "BoloSingleChannelFeedback"  # label
              # "DimensionB"
              n786 = call "W7X2DJSON.vi"("values"=w2157, "label"=w2166, "dimensionSize"=w2158, "dimensions"=w2153, "dimensionCount"=1, "sampleCount"=w2158, "datatype"=w2163) -> ("JSON string"=w2165:string)  [unwired: 4 in]
              n787 = disable-structure shown="Disabled" {
                disable-tunnel: w2165 -> [w2168 _]
                frame Disabled {
                  "SingleChannelFeedbackJSON" <- w2168
                }
                frame Enabled {
                }
              }
              n788 = call "W7X2DPut.vi"("SigLabel"=w2166, "Unit"=w2167, "SigJSONbuffer"=w2165, "values"=w2156, "dimensions"=w2159, "sample rate"=w2154, "sample period"=w2155, "pulse_length"=w2155) -> ("headers parms"=→"headers parms 12":string, "headers"=→"headers 12":string, "body"=→"body 12":string, "body Parlog"=→"body Parlog 12":string, "file path written"=→"SingleChannelFeedback path":string, "Parlog error out"=w2161:errorcluster)  [unwired: 2 in]
              "SingleChannelFeedbackErrorOut" <- w2161
              n789 = Unbundle(w2161) -> ("status"=→"SingleChannelFeedback status":bool)  [unwired: 2 out]
            }
            frame Disabled {
              w2183 = "V"  # Unit
              w2184 = "Float"  # datatype
              w2178 = "BoloSingleChannelFeedback"  # label
              n790 = call "W7X1DJSON.vi"("values"=w2179, "label"=w2178, "Unit"=w2183, "dimensions"=w2170, "dimensionCount"=w2180, "datatype"=w2184) -> ("JSON string"=w2182:string)  [unwired: 5 in]
              n791 = disable-structure shown="Disabled" {
                disable-tunnel: w2182 -> [w2185 _]
                frame Disabled {
                  n792 = local write "SingleChannelFeedbackJSON"(w2185) -> ()
                }
                frame Enabled {
                }
              }
              n793 = call "W7X1DPut.vi"("dimensions"=w2169, "Unit"=w2183, "values"=w2181, "SigJSONbuffer"=w2182, "SigLabel"=w2178) -> ("Parlog error out"=w2176:errorcluster, "file path written"=w2177:string, "headers parms"=w2172:string, "body Parlog"=w2173:string, "body"=w2174:string, "headers"=w2171:string)  [unwired: 1 in]
              n794 = local write "SingleChannelFeedbackErrorOut"(w2176) -> ()
              n795 = local write "SingleChannelFeedback path"(w2177) -> ()
              n796 = Unbundle(w2176) -> ("status"=w2175:bool)  [unwired: 2 out]
              n797 = local write "SingleChannelFeedback status"(w2175) -> ()
            }
          }
          n798 = disable-structure shown="Enabled" {
            disable-tunnel: w1947 -> [w2252 _]
            disable-tunnel: w1938 -> [w2251 _]
            disable-tunnel: w1937 -> [w2250 _]
            disable-tunnel: w1964 -> [w2249 _]
            disable-tunnel: w1940 -> [w2247 _]
            disable-tunnel: w1939 -> [w2248 _]
            frame Enabled {
              w2258 = "A"  # Unit
              w2259 = 10000 ("sampleCount")
              w2261 = "Float"  # datatype
              w2257 = "BoloCalibRefFoilCurrent"  # label
              n799 = call "W7X2DJSON.vi"("values"=w2249, "label"=w2257, "dimensionSize"=w2259, "dimensions"=w2252, "dimensionCount"=128, "sampleCount"=w2259, "datatype"=w2261) -> ("JSON string"=w2256:string)  [unwired: 4 in]
              n800 = disable-structure shown="Disabled" {
                disable-tunnel: w2256 -> [w2262 _]
                frame Disabled {
                  # "DimensionC"
                  "CalibRefFoilCurrentJSON" <- w2262
                }
                frame Enabled {
                }
              }
              n801 = call "W7X2DPut.vi"("SigLabel"=w2257, "Unit"=w2258, "SigJSONbuffer"=w2256, "values"=w2250, "dimensions"=w2251, "sample rate"=w2248, "sample period"=w2247, "pulse_length"=w2247) -> ("headers parms"=→"headers parms 8":string, "headers"=→"headers 8":string, "body"=→"body 8":string, "body Parlog"=→"body Parlog 8":string, "file path written"=→"CalibRefFoilCurrent path":string, "Parlog error out"=w2255:errorcluster)  [unwired: 2 in]
              "CalibRefFoilCurrentErrorOut" <- w2255
              n802 = Unbundle(w2255) -> ("status"=→"CalibRefFoilCurrent status":bool)  [unwired: 2 out]
            }
            frame Disabled {
            }
          }
          n803 = disable-structure shown="Enabled" {
            disable-tunnel: w1938 -> [w2065 _]
            disable-tunnel: w1947 -> [w2064 _]
            disable-tunnel: w1937 -> [w2063 _]
            frame Enabled {
              n804 = call <vilib>:"OpenHandle.vi"() -> ("client handle out"=w2082:T52, "error out"=w2081:errorcluster)  [unwired: 14 in]
              n805 = call <vilib>:"AddHeader.vi"("client handle"=w2082, "header"="Content-Type", "value"="application/json", "error in (no error)"=w2081) -> ("client handle out"=w2080:T52, "error out"=w2079:errorcluster)  [unwired: 10 in]
              n806 = call "parmsQSB.vi"("dimensions"=w2065, "values"=w2063, "label"="parms") -> ("JSON string"=w2068:string)
              n807 = disable-structure shown="Disabled" {
                disable-tunnel: w2068 -> [w2086 _]
                frame Disabled {
                  "QSB Parms JSON string" <- w2086
                }
                frame Enabled {
                }
              }
              n808 = call "saveToFile.vi"("SigJSONbuffer"=w2068, "dimensions"=w2064, "String"="File_PARLOG" ("name or relative path")) -> ("error out"=w2069:errorcluster, "resulting string"=→"QSBParms path":string)  [unwired: 7 in]
              n809 = Unbundle(w2069) -> ("status"=→"QSBParms status":bool)  [unwired: 2 out]
              n810 = call-poly <vilib>:"POST.vi"("client handle"=w2080, "url"="http://archive-webapi/Test/raw/W7X/QSB_Bolometry/File_PARLOG/", "buffer"=w2068, "error in (no error)"=w2079, "timeout (10000)"=400000 ("timeout for upload")) -> ("client handle out"=w2084:T52, "headers"=→"QSB Parms Out headers chanDesc":string, "body"=→"QSB Parms Out body chanDesc":string, "error out"=w2070:errorcluster)  [unwired: 7 in]
              n811 = call <vilib>:"CloseHandle.vi"("client handle"=w2084, "error in (no error)"=w2070) -> ("error out"=w2074:errorcluster)  [unwired: 13 in]
              n812 = Merge Errors(w2074, w2069) -> (→"parms error out":errorcluster)
            }
            frame Disabled {
            }
          }
          n813 = disable-structure shown="Enabled" {
            disable-tunnel: w1957 -> [w2343 w2367]
            disable-tunnel: w1961 -> [_ w2366]
            disable-tunnel: w1937 -> [w2345 w2365]
            disable-tunnel: w1938 -> [w2342 w2364]
            disable-tunnel: w1951 -> [w2344 _]
            frame Enabled {
              w2349 = 1 ("sampleCount")
              w2354 = "Float"  # datatype
              w2352 = "Ohms"  # Unit
              w2351 = "MRes"  # label
              n814 = call "W7X2DJSON.vi"("values"=w2344, "label"=w2351, "dimensionSize"=w2349, "dimensions"=w2343, "dimensionCount"=128, "sampleCount"=w2349, "datatype"=w2354) -> ("JSON string"=w2350:string)  [unwired: 4 in]
              n815 = disable-structure shown="Disabled" {
                disable-tunnel: w2350 -> [w2355 _]
                frame Disabled {
                  # "DimensionC"
                  "MResJSON" <- w2355
                }
                frame Enabled {
                }
              }
              n816 = call "W7X1DPut.vi"("dimensions"=w2342, "Unit"=w2352, "values"=w2345, "SigJSONbuffer"=w2350, "SigLabel"=w2351) -> ("Parlog error out"=w2348:errorcluster, "file path written"=→"MRes path":string, "headers parms"=w2339:string, "body Parlog"=w2340:string, "body"=w2341:string, "headers"=w2338:string)  [unwired: 1 in]
              "MResErrorOut" <- w2348
              n817 = Unbundle(w2348) -> ("status"=→"MRes status":bool)  [unwired: 2 out]
              n818 = local write "headers parms 6"(w2339) -> ()
              n819 = local write "headers 6"(w2338) -> ()
              n820 = local write "body Parlog 6"(w2340) -> ()
              n821 = local write "body 6"(w2341) -> ()
            }
            frame Disabled {
              w2368 = "Ohms"  # Unit
              w2370 = "Float"  # datatype
              w2369 = "MRes"  # label
              n822 = call "W7X1DJSON.vi"("values"=w2366, "label"=w2369, "Unit"=w2368, "dimensions"=w2367, "dimensionCount"=128, "datatype"=w2370) -> ("JSON string"=w2363:string)  [unwired: 5 in]
              n823 = disable-structure shown="Disabled" {
                disable-tunnel: w2363 -> [_ _]
                frame Disabled {
                  n824 = local read "MKappaJSON"() -> ()  [unwired: 1 in]
                }
                frame Enabled {
                }
              }
              n825 = call "W7X1DPut.vi"("dimensions"=w2364, "Unit"=w2368, "values"=w2365, "SigJSONbuffer"=w2363, "SigLabel"=w2369) -> ("Parlog error out"=w2362:errorcluster, "file path written"=w2360:string, "headers parms"=→"headers parms 6":string, "body Parlog"=→"body Parlog 6":string, "body"=→"body 6":string, "headers"=→"headers 6":string)  [unwired: 1 in]
              n826 = local write "MResErrorOut"(w2362) -> ()
              n827 = local write "MRes path"(w2360) -> ()
              n828 = Unbundle(w2362) -> ("status"=w2361:bool)  [unwired: 2 out]
              n829 = local write "MRes status"(w2361) -> ()
            }
          }
          n830 = disable-structure shown="Enabled" {
            disable-tunnel: w1943 -> [_ w2336]
            disable-tunnel: w1937 -> [w2309 w2331]
            disable-tunnel: w1938 -> [w2307 w2330]
            disable-tunnel: w1957 -> [w2308 w2329]
            disable-tunnel: w1949 -> [w2310 _]
            frame Enabled {
              w2314 = 1 ("sampleCount")
              w2317 = "s"  # Unit
              w2319 = "Float"  # datatype
              w2316 = "MTau"  # label
              n831 = call "W7X2DJSON.vi"("values"=w2310, "label"=w2316, "dimensionSize"=w2314, "dimensions"=w2308, "dimensionCount"=128, "sampleCount"=w2314, "datatype"=w2319) -> ("JSON string"=w2315:string)  [unwired: 4 in]
              n832 = disable-structure shown="Disabled" {
                disable-tunnel: w2315 -> [w2320 _]
                frame Disabled {
                  # "DimensionC"
                  "MTauJSON" <- w2320
                }
                frame Enabled {
                }
              }
              n833 = call "W7X1DPut.vi"("dimensions"=w2307, "Unit"=w2317, "values"=w2309, "SigJSONbuffer"=w2315, "SigLabel"=w2316) -> ("Parlog error out"=w2313:errorcluster, "file path written"=→"MTau path":string, "headers parms"=w2303:string, "body Parlog"=w2305:string, "body"=w2306:string, "headers"=w2304:string)  [unwired: 1 in]
              "MTauErrorOut" <- w2313
              n834 = Unbundle(w2313) -> ("status"=→"MTau status":bool)  [unwired: 2 out]
              n835 = local write "headers parms 16"(w2303) -> ()
              n836 = local write "headers 16"(w2304) -> ()
              n837 = local write "body Parlog 16"(w2305) -> ()
              n838 = local write "body 16"(w2306) -> ()
            }
            frame Disabled {
              w2334 = "s"  # Unit
              w2333 = "Float"  # datatype
              w2332 = "MTau"  # label
              n839 = call "W7X1DJSON.vi"("values"=w2336, "label"=w2332, "Unit"=w2334, "dimensions"=w2329, "dimensionCount"=128, "datatype"=w2333) -> ("JSON string"=w2328:string)  [unwired: 5 in]
              n840 = disable-structure shown="Disabled" {
                disable-tunnel: w2328 -> [w2337 _]
                frame Disabled {
                  n841 = local write "MTauJSON"(w2337) -> ()
                }
                frame Enabled {
                }
              }
              n842 = call "W7X1DPut.vi"("dimensions"=w2330, "values"=w2331, "SigJSONbuffer"=w2328, "SigLabel"=w2332) -> ("Parlog error out"=w2327:errorcluster, "file path written"=w2325:string, "headers parms"=→"headers parms 16":string, "body Parlog"=→"body Parlog 16":string, "body"=→"body 16":string, "headers"=→"headers 16":string)  [unwired: 2 in]
              n843 = local write "MTauErrorOut"(w2327) -> ()
              n844 = local write "MTau path"(w2325) -> ()
              n845 = Unbundle(w2327) -> ("status"=w2326:bool)  [unwired: 2 out]
              n846 = local write "MTau status"(w2326) -> ()
            }
          }
          n847 = local write "state"("Uploading to archive ...." ("state")) -> ()
          n848 = disable-structure shown="Enabled" {
            disable-tunnel: w1960 -> [w2292 _]
            disable-tunnel: w1947 -> [w2283 _]
            disable-tunnel: w1940 -> [w2291 _]
            disable-tunnel: w1939 -> [w2290 _]
            disable-tunnel: w1937 -> [w2289 _]
            disable-tunnel: w1938 -> [w2284 _]
            frame Enabled {
              w2298 = "A"  # Unit
              w2299 = 10000 ("sampleCount")
              w2301 = "Float"  # datatype
              w2297 = "BoloCalibMeasFoilCurrent"  # label
              n849 = call "W7X2DJSON.vi"("values"=w2292, "label"=w2297, "dimensionSize"=w2299, "dimensions"=w2283, "dimensionCount"=128, "sampleCount"=w2299, "datatype"=w2301) -> ("JSON string"=w2296:string)  [unwired: 4 in]
              n850 = disable-structure shown="Disabled" {
                disable-tunnel: w2296 -> [w2302 _]
                frame Disabled {
                  # "DimensionC"
                  "CalibMeasFoilCurrentJSON" <- w2302
                }
                frame Enabled {
                }
              }
              n851 = call "W7X2DPut.vi"("SigLabel"=w2297, "Unit"=w2298, "SigJSONbuffer"=w2296, "values"=w2289, "dimensions"=w2284, "sample rate"=w2290, "sample period"=w2291, "pulse_length"=w2291) -> ("headers parms"=→"headers parms 7":string, "headers"=→"headers 7":string, "body"=→"body 7":string, "body Parlog"=→"body Parlog 7":string, "file path written"=→"CalibMeasFoilCurrent path":string, "Parlog error out"=w2295:errorcluster)  [unwired: 2 in]
              "CalibMeasFoilCurrentErrorOut" <- w2295
              n852 = Unbundle(w2295) -> ("status"=→"CalibMeasFoilCurrent status":bool)  [unwired: 2 out]
            }
            frame Disabled {
            }
          }
          n853 = disable-structure shown="Enabled" {
            disable-tunnel: w1937 -> [w2273 _]
            disable-tunnel: w1942 -> [w2264 _]
            disable-tunnel: w1959 -> [w2272 _]
            disable-tunnel: w1938 -> [w2271 _]
            disable-tunnel: w1940 -> [w2270 _]
            disable-tunnel: w1939 -> [w2269 _]
            disable-tunnel: w1941 -> [w2263 _]
            frame Enabled {
              w2281 = "V"  # Unit
              w2277 = "Float"  # datatype
              w2280 = "BoloSignal"  # label
              # "DimensionB"
              n854 = call "W7X2DJSON.vi"("values"=w2272, "label"=w2280, "dimensionSize"=w2264, "dimensions"=w2263, "dimensionCount"=128, "sampleCount"=w2264, "datatype"=w2277) -> ("JSON string"=w2279:string)  [unwired: 4 in]
              n855 = disable-structure shown="Disabled" {
                disable-tunnel: w2279 -> [w2282 _]
                frame Disabled {
                  "BoloSignalJSON" <- w2282
                }
                frame Enabled {
                }
              }
              n856 = call "W7X2DPut.vi"("SigLabel"=w2280, "Unit"=w2281, "SigJSONbuffer"=w2279, "values"=w2273, "dimensions"=w2271, "sample rate"=w2269, "sample period"=w2270, "pulse_length"=w2270) -> ("headers parms"=→"headers parms 9":string, "headers"=→"headers 9":string, "body"=→"body 9":string, "body Parlog"=→"body Parlog 9":string, "file path written"=→"BoloSignal path":string, "Parlog error out"=w2276:errorcluster)  [unwired: 2 in]
              "BoloSignalErrorOut" <- w2276
              n857 = Unbundle(w2276) -> ("status"=→"BoloSignal status":bool)  [unwired: 2 out]
            }
            frame Disabled {
            }
          }
          n858 = disable-structure shown="Enabled" {
            disable-tunnel: w1957 -> [_ w2218]
            disable-tunnel: w1942 -> [w2195 w2217]
            disable-tunnel: w1958 -> [_ w2216]
            disable-tunnel: w1937 -> [w2192 w2215]
            disable-tunnel: w1941 -> [w2191 w2214]
            disable-tunnel: w1948 -> [w2196 _]
            disable-tunnel: w1940 -> [w2194 _]
            disable-tunnel: w1939 -> [w2193 _]
            disable-tunnel: w1938 -> [w2190 _]
            frame Enabled {
              w2204 = "MW"  # Unit
              w2201 = "Float"  # datatype
              w2203 = "Bolo_HBCmPrad"  # label
              n859 = call "W7X2DJSON.vi"("values"=w2196, "label"=w2203, "dimensionSize"=w2195, "dimensions"=w2191, "dimensionCount"=1, "sampleCount"=w2195, "datatype"=w2201) -> ("JSON string"=w2202:string)  [unwired: 4 in]
              n860 = disable-structure shown="Disabled" {
                disable-tunnel: w2202 -> [w2205 _]
                frame Disabled {
                  "Bolo_HBCmPrad JSON" <- w2205
                }
                frame Enabled {
                }
              }
              n861 = call "W7X2DPut.vi"("SigLabel"=w2203, "Unit"=w2204, "SigJSONbuffer"=w2202, "values"=w2192, "dimensions"=w2190, "sample rate"=w2193, "sample period"=w2194, "pulse_length"=w2194) -> ("headers parms"=w2189:string, "headers"=w2188:string, "body"=w2187:string, "body Parlog"=w2186:string, "file path written"=→"Bolo_HBCmPrad path":string, "Parlog error out"=w2199:errorcluster)  [unwired: 2 in]
              "Bolo_HBCmPrad ErrorOut" <- w2199
              n862 = local write "body Parlog 13"(w2186) -> ()
              n863 = local write "headers parms 13"(w2189) -> ()
              n864 = local write "headers 13"(w2188) -> ()
              n865 = local write "body 13"(w2187) -> ()
              n866 = Unbundle(w2199) -> ("status"=→"Bolo_HBCmPrad status":bool)  [unwired: 2 out]
            }
            frame Disabled {
              w2220 = "MW"  # Unit
              w2221 = "Float"  # datatype
              w2219 = "Bolo_HBCmPrad"  # label
              n867 = call "W7X1DJSON.vi"("values"=w2216, "label"=w2219, "Unit"=w2220, "dimensions"=w2218, "dimensionCount"=w2217, "datatype"=w2221) -> ("JSON string"=w2213:string)  [unwired: 5 in]
              n868 = disable-structure shown="Disabled" {
                disable-tunnel: w2213 -> [w2222 _]
                frame Disabled {
                  n869 = local write "Bolo_HBCmPrad JSON"(w2222) -> ()
                }
                frame Enabled {
                }
              }
              n870 = call "W7X1DPut.vi"("dimensions"=w2214, "Unit"=w2220, "values"=w2215, "SigJSONbuffer"=w2213, "SigLabel"=w2219) -> ("Parlog error out"=w2212:errorcluster, "file path written"=w2210:string, "headers parms"=→"headers parms 13":string, "body Parlog"=→"body Parlog 13":string, "body"=→"body 13":string, "headers"=→"headers 13":string)  [unwired: 1 in]
              n871 = local write "Bolo_HBCmPrad ErrorOut"(w2212) -> ()
              n872 = local write "Bolo_HBCmPrad path"(w2210) -> ()
              n873 = Unbundle(w2212) -> ("status"=w2211:bool)  [unwired: 2 out]
              n874 = local write "Bolo_HBCmPrad status"(w2211) -> ()
            }
          }
          n875 = disable-structure shown="Enabled" {
            disable-tunnel: w1937 -> [w2001 w2019]
            disable-tunnel: w1941 -> [w1998 w2014]
            disable-tunnel: w1938 -> [w2003 w2013]
            disable-tunnel: w1945 -> [w2002 _]
            disable-tunnel: w1940 -> [w2000 _]
            disable-tunnel: w1939 -> [w1999 _]
            disable-tunnel: w1942 -> [w1997 _]
            frame Enabled {
              w2011 = "V"  # Unit
              w2007 = "Float"  # datatype
              w2010 = "BoloRealTime_P_rad"  # label
              n876 = call "W7X2DJSON.vi"("values"=w2002, "label"=w2010, "dimensionSize"=w1997, "dimensions"=w1998, "dimensionCount"=1, "sampleCount"=w1997, "datatype"=w2007) -> ("JSON string"=w2009:string)  [unwired: 4 in]
              n877 = disable-structure shown="Disabled" {
                disable-tunnel: w2009 -> [w2012 _]
                frame Disabled {
                  "RT_P_rad Json" <- w2012
                }
                frame Enabled {
                }
              }
              n878 = call "W7X2DPut.vi"("SigLabel"=w2010, "Unit"=w2011, "SigJSONbuffer"=w2009, "values"=w2001, "dimensions"=w2003, "sample rate"=w1999, "sample period"=w2000, "pulse_length"=w2000) -> ("headers parms"=→"headers parms 17":string, "headers"=→"headers 17":string, "body"=→"body 17":string, "body Parlog"=→"body Parlog 17":string, "file path written"=→"RT_P_rad path":string, "Parlog error out"=w2005:errorcluster)  [unwired: 2 in]
              "RT_P_rad ErrorOut" <- w2005
              n879 = Unbundle(w2005) -> ("status"=→"RT_P_rad status":bool)  [unwired: 2 out]
            }
            frame Disabled {
              w2021 = "V"  # Unit
              w2022 = "Float"  # datatype
              w2018 = "BoloSingleChannelFeedback"  # label
              n880 = call "W7X1DJSON.vi"("label"=w2018, "Unit"=w2021, "dimensions"=w2014, "datatype"=w2022) -> ("JSON string"=w2020:string)  [unwired: 7 in]
              n881 = disable-structure shown="Disabled" {
                disable-tunnel: w2020 -> [w2023 _]
                frame Disabled {
                  n882 = local write "RT_P_rad Json"(w2023) -> ()
                }
                frame Enabled {
                }
              }
              n883 = call "W7X1DPut.vi"("dimensions"=w2013, "Unit"=w2021, "values"=w2019, "SigJSONbuffer"=w2020, "SigLabel"=w2018) -> ("Parlog error out"=w2016:errorcluster, "file path written"=w2017:string)  [unwired: 1 in, 4 out]
              n884 = local write "RT_P_rad ErrorOut"(w2016) -> ()
              n885 = local write "RT_P_rad path"(w2017) -> ()
              n886 = Unbundle(w2016) -> ("status"=w2015:bool)  [unwired: 2 out]
              n887 = local write "RT_P_rad status"(w2015) -> ()
            }
          }
          n888 = disable-structure shown="Enabled" {
            disable-tunnel: w1942 -> [w2041 w2051]
            disable-tunnel: w1957 -> [_ w2050]
            disable-tunnel: w1956 -> [_ w2049]
            disable-tunnel: w1937 -> [w2036 w2048]
            disable-tunnel: w1947 -> [_ _]
            disable-tunnel: w1946 -> [w2042 _]
            disable-tunnel: w1940 -> [w2035 _]
            disable-tunnel: w1939 -> [w2034 _]
            disable-tunnel: w1941 -> [w2029 _]
            disable-tunnel: w1938 -> [w2028 _]
            frame Enabled {
              w2038 = "MW"  # Unit
              w2039 = "Float"  # datatype
              w2037 = "Bolo_VBCPrad"  # label
              n889 = call "W7X2DJSON.vi"("values"=w2042, "label"=w2037, "dimensionSize"=w2041, "dimensions"=w2029, "dimensionCount"=1, "sampleCount"=w2041, "datatype"=w2039) -> ("JSON string"=w2030:string)  [unwired: 4 in]
              n890 = disable-structure shown="Disabled" {
                disable-tunnel: w2030 -> [w2043 _]
                frame Disabled {
                  n891 = local write "Bolo_VBCPradJson"(w2043) -> ()
                }
                frame Enabled {
                }
              }
              n892 = call "W7X2DPut.vi"("SigLabel"=w2037, "Unit"=w2038, "SigJSONbuffer"=w2030, "values"=w2036, "dimensions"=w2028, "sample rate"=w2034, "sample period"=w2035, "pulse_length"=w2035) -> ("headers parms"=→"headers parms 14":string, "headers"=→"headers 14":string, "body"=→"body 14":string, "body Parlog"=→"body Parlog 14":string, "file path written"=w2031:string, "Parlog error out"=w2033:errorcluster)  [unwired: 2 in]
              n893 = local write "Bolo_VBCPrad ErrorOut"(w2033) -> ()
              n894 = local write "Bolo_VBCPrad path"(w2031) -> ()
              n895 = Unbundle(w2033) -> ("status"=w2032:bool)  [unwired: 2 out]
              n896 = local write "Bolo_VBCPrad status"(w2032) -> ()
            }
            frame Disabled {
              w2057 = "MW"  # Unit
              w2058 = "Float"  # datatype
              w2056 = "Bolo_VBCPrad"  # label
              n897 = call "W7X1DJSON.vi"("values"=w2049, "label"=w2056, "Unit"=w2057, "dimensions"=w2050, "dimensionCount"=w2051, "datatype"=w2058) -> ("JSON string"=w2055:string)  [unwired: 5 in]
              n898 = disable-structure shown="Disabled" {
                disable-tunnel: w2055 -> [w2059 _]
                frame Disabled {
                  "Bolo_VBCPradJson" <- w2059
                }
                frame Enabled {
                }
              }
              n899 = call "W7X1DPut.vi"("Unit"=w2057, "values"=w2048, "SigJSONbuffer"=w2055, "SigLabel"=w2056) -> ("Parlog error out"=w2052:errorcluster, "file path written"=→"Bolo_VBCPrad path":string, "headers parms"=w2045:string, "body Parlog"=w2046:string, "body"=w2047:string, "headers"=w2044:string)  [unwired: 2 in]
              "Bolo_VBCPrad ErrorOut" <- w2052
              n900 = Unbundle(w2052) -> ("status"=→"Bolo_VBCPrad status":bool)  [unwired: 2 out]
            }
          }
          n901 = disable-structure shown="Enabled" {
            disable-tunnel: w1937 -> [w1983 _]
            disable-tunnel: w1942 -> [w1974 _]
            disable-tunnel: w1936 -> [w1982 _]
            disable-tunnel: w1938 -> [w1981 _]
            disable-tunnel: w1940 -> [w1980 _]
            disable-tunnel: w1939 -> [w1979 _]
            disable-tunnel: w1941 -> [w1973 _]
            frame Enabled {
              w1991 = "V"  # Unit
              w1987 = "Float"  # datatype
              w1990 = "BoloAdjusted"  # label
              # "DimensionB"
              n902 = call "W7X2DJSON.vi"("values"=w1982, "label"=w1990, "dimensionSize"=w1974, "dimensions"=w1973, "dimensionCount"=128, "sampleCount"=w1974, "datatype"=w1987) -> ("JSON string"=w1989:string)  [unwired: 4 in]
              n903 = disable-structure shown="Disabled" {
                disable-tunnel: w1989 -> [w1992 _]
                frame Disabled {
                  "BoloSignalJSON 2" <- w1992
                }
                frame Enabled {
                }
              }
              n904 = call "W7X2DPut.vi"("SigLabel"=w1990, "Unit"=w1991, "SigJSONbuffer"=w1989, "values"=w1983, "dimensions"=w1981, "sample rate"=w1979, "sample period"=w1980, "pulse_length"=w1980) -> ("headers parms"=→"headers parms 18":string, "headers"=→"headers 18":string, "body"=→"body 18":string, "body Parlog"=→"body Parlog 18":string, "file path written"=→"BoloAdjusted path":string, "Parlog error out"=w1986:errorcluster)  [unwired: 2 in]
              "BoloSignalErrorOut 2" <- w1986
              n905 = Unbundle(w1986) -> ("status"=→"BoloSignal status 2":bool)  [unwired: 2 out]
            }
            frame Disabled {
            }
          }
        }
        frame Disabled {
        }
      }
      "DimensionsA" <- w1916
      "DimensionsB" <- w1914
      "DimensionsC" <- w1915
      "DimensionsD" <- w1921
      "DimensionA2" <- w1917
    }
    frame #5 {
      n906 = local write "state"("Idle / Waiting for new Trigger" ("state")) -> ()
      n907 = case shown="True" w2568 {
        tunnel: w2567 -> [w2572 w2574]
        tunnel: w2566 -> [_ w2573]
        tunnel: [w2572 _] -> w2570
        frame False {
        }
        frame True {
          n908 = xnode "Close FPGA VI Reference"("FPGA VI Reference In"=w2574, "error in"=w2573) -> ()  [unwired: 1 out]
        }
      }
      "FPGA VI Reference Out" <- w2570
      n909 = property on="stop" class="Bool (strict)"("Val(Sgnl)"=TRUE) -> ()  [unwired: 2 in, 2 out]
    }
  }
